vi "ControlProgram6.6_7_test_image_fixedxy.vi"() -> ()   [LabVIEW 2016]
uses:
  <vilib>/Utility/miscctls.llb/LVPoint32TypeDef.ctl
  <vilib>/Platform/TimedLoop/XDataNode/timing_clust.ctl
  <vilib>/Platform/TimedLoop/XDataNode/nitl_modes.ctl
  <vilib>/Platform/TimedLoop/XDataNode/wakeup.ctl
  <vilib>/Instr/_visa.llb/Select Event Type.ctl
  <vilib>/vision/Avi1.llb/AviRefnum.ctl
  <vilib>/Utility/error.llb/DialogType.ctl
  <vilib>/DAQmx/write.llb/DAQmx Write (Analog 1D DBL NChan 1Samp).vi
  <vilib>/DAQmx/read.llb/DAQmx Read (Analog 2D DBL NChan NSamp).vi
  <vilib>/Analysis/baseanly.llb/Mean (DBL).vi
  <vilib>/DAQmx/write.llb/DAQmx Write (Digital Bool 1Line 1Point).vi
  <vilib>/DAQmx/create/channels.llb/DAQmx Create Channel (DO-Digital Output).vi
  <vilib>/DAQmx/create/channels.llb/DAQmx Create Channel (AI-Voltage-Basic).vi
  <vilib>/DAQmx/create/channels.llb/DAQmx Create Channel (AO-Voltage-Basic).vi
  <vilib>/DAQmx/configure/timing.llb/DAQmx Timing (Sample Clock).vi
  <vilib>/DAQmx/miscellaneous.llb/DAQmx Fill In Error Info.vi
  <vilib>/Instr/_visa.llb/VISA Configure Serial Port (Instr).vi
  Arnulf--joystick/git(most_up_to_date)/Logitech-joystick/Old Trap/FAST_Global_var.vi
  <vilib>/Utility/inputDevices.llb/mouseAcquire.vi
  <vilib>/Utility/inputDevices.llb/closeMouse.vi
  <vilib>/platform/TimedLoop/XDataNode/XDataNode.xnode
  <vilib>/Platform/TimedLoop/XDataNode/XDNodeRunTimeDep.lvlib
  <resource>/objmgr/daqmx.rc
  <vilib>/Analysis/NI_AALBase.lvlib
panel:
  in  "Save file index":i32
  out "Saving Move":bool
  out "Move time":string
  out "Primary Video Display":T1(plugin-control)
  out "Flush Sample Start Time":u32=2111292881
  out "Sample flush time (s)":dbl=48.0
  in  "Inject Sample":bool
  out "Cal values":T2={"AX alpha"=612.9626061060078, "BX alpha"=549.6584469744151, "AX kappa"=0.3485731373010688, "BX kappa"=0.3853424216291352, "AX offset"=-0.03900484438240665, "BX offset"=-0.11295550662085417, "AY alpha"=582.7562541114835, "BY alpha"=571.1587543790358, "AY kappa"=0.37498408087930674, "BY kappa"=0.36252029651198364, "AY offset"=-0.21125584642206058, "BY offset"=-0.12469077200400738}
  in  "Inject Pump 1":bool
  in  "Inject Pump 2":bool
  in  "Tab Control 2":T3(tab)
  in  "Force FB script":bool
  in  "Got ADig bead":bool
  in  "Move Cap. 2 (ADig Top)":bool
  in  "Dump beads":bool
  in  "Got DNA bead":bool
  in  "Flow on\ncap 2?":bool=TRUE
  in  "Flow on\ncap 1?":bool=TRUE
  in  "Flow on\ndump?":bool=TRUE
  in  "Raster set":i32=1
  in  "Fish After TA?":bool=TRUE
  in  "Delta after tether":dbl=1700.0
  in  "TA Cancel Save?":bool=TRUE
  in  "Min fish\ndelta (nm)":dbl=1425.0 min=0.0 max=5000.0 step=50.0
  in  "Max fish\ndelta (nm)":dbl=1900.0 min=0.0 max=5000.0 step=25.0
  in  "Fish Speed (ms)":i32=5000
  in  "Wait (ms)":i32=1500
  in  "# attempts":dbl=10.0
  in  "Cutoff force (pN)":dbl=4.5
  in  "Raster after\n tether?":bool=TRUE
  out "Tether":bool
  out "Attempt #":i32
  in  "Flow on\nwhile fish?":bool=TRUE
  in  "Flow on\nafter raster?":bool=TRUE
  in  "Offset raster set":i32
  in  "Offset @ Delta (nm)":dbl=1700.0
  in  "Cal @ Delta (nm)":dbl=2500.0
  in  "Cal stage position":i32=3
  out "Cal Final Sampling Rate":dbl=125000.0
  in  "Cal Averaging":i32=1
  in  "Wait before dip (s)":dbl=3.0
  in  "Start dipping after?":bool
  in  "Start trap delta (nm)":dbl=1700.0
  in  "Repeat Dip":bool
  out "Dip #":i32
  in  "Dip attempts":dbl=3.0
  in  "Cancel Rep\n Dip":bool
  out "Return elasped time":i32
  in  "Return duration":dbl=15.0
  in  "Cancel dwell":bool=TRUE
  in  "Pause dwell":bool
  in  "Start/Return position":dbl=3.0
  in  "Dip duration":dbl=15.0
  in  "Dip position":dbl=4.0
  in  "Dip":bool
  out "Dip elasped time":i32
  in  "Stop":bool=TRUE
  in  "?":T4(tab)
  out "FAST X-Y":bool
  out "FAST Z":bool
  in  "Cal time (s)":dbl=5.0
  in  "Save N sets":bool
  in  "N sets":i32=200
  out "Cal sets to save":i32=500
  in  "Reset data stream":bool
  out "Buffer Overflow":bool
  out "Stage moving":bool
  in  "Comment":string
  in  "Raster scan":bool
  out "Saving":bool
  in  "Save cal":bool
  in  "Save Data":bool
  in  "Stop saving":bool
  out "Calibrating":bool
  out "Progress":dbl(slide) scale=0.0..100.0
  in  "Read Cal":bool
  in  "Fish":bool
  in  "Averaging Number":i32=1250
  out "Final Sampling Rate":dbl=100.0
  in  "Trap position (V)":cluster{"X":dbl, "Y":dbl}={"X"=3.9042624789680316, "Y"=0.2}
  in  "Trap delta (nm)":dbl=2500.0 min=0.0 max=5000.0 step=50.0
  in  "Fixed X":dbl=1.1
  in  "Fixed Y":dbl=0.15
  in  "Shutter 1 (B)":bool
  in  "Shutter 2 (A)":bool
  in  "Pulling direction":bool
  out "Raster scanning...":bool
  out "Current file name":path=path "D:/data/160111/160111_006.dat"
  in  "AX alpha":dbl=612.9626061060078 format="%#_3p"
  in  "BX alpha":dbl=549.6584469744151 format="%#_3g"
  in  "AX kappa":dbl=0.3485731373010688 format="%#_3g"
  in  "BX kappa":dbl=0.3853424216291352 format="%#_3g"
  in  "AX offset":dbl=-0.03900484438240665 format="%#_3g"
  in  "BX offset":dbl=-0.11295550662085417 format="%#_3g"
  in  "AY alpha":dbl=582.7562541114835 format="%#_3g"
  in  "BY alpha":dbl=571.1587543790358 format="%#_3g"
  in  "AY kappa":dbl=0.37498408087930674 format="%#_3g"
  in  "BY kappa":dbl=0.36252029651198364 format="%#_3g"
  in  "AY offset":dbl=-0.21125584642206058 format="%#_3g"
  in  "BY offset":dbl=-0.12469077200400738 format="%#_3g"
  out "Buffer status":u8(slide) scale=0.0..100.0
  in  "Target":bool
  in  "Set Current\nPos to (0,0,0)":bool
  in  "dump spot":string="Dump beads spot"
  in  "up flow spot":string="Upper flow spot"
  in  "low flow spot":string="Lower flow spot"
  in  "up cap":string="Upper capillary (ADig beads)"
  in  "bottom cap":string="Lower capillary (DNA beads)"
  in  "Move to Position 5":bool
  in  "Set Position 5":bool
  in  "Saved stage positions":dbl[][](array[numeric])=[[1.0, 0.0, 0.0, 0.0], [2.0, -0.13716, -3.21132, 0.01436], [3.0, 0.45, -0.73974, 0.005], [4.0, 0.45, -2.1978, 0.005], [5.0, 0.45, -2.63158, -0.02256]]
  in  "Set Position 2":bool
  in  "Move to Position 2":bool
  in  "Set Position 1":bool
  in  "Move to Position 1":bool
  in  "Set Position 4":bool
  in  "Move to Position 4":bool
  in  "Set Position 3":bool
  in  "Move to Position 3":bool
  out "Stage error":errorcluster
  in  "Clear Volume":bool
  out "Sample Flush Meter":u8(slide) scale=0.0..100.0
  out "Flushing Sample":bool
  in  "Flush Sample":bool
  in  "Normal \nRate (ul/hr)  3":dbl=100.0
  in  "Normal \nVolume (ul) 3":dbl=250.0
  in  "Normal \nVolume (ul) 2":dbl
  in  "Normal \nRate (ul/hr)":dbl
  in  "Normal \nVolume (ul)":dbl
  in  "Flush\nRate (ul/min)":dbl
  in  "Flush\nVolume (ul)":dbl
  in  "Flush \nRate (ul/min)  2":dbl
  in  "Flush Pump 2":bool
  in  "Flush\nVolume (ul)  2":dbl
  in  "Flush Pump 1":bool
  in  "Normal \nRate (ul/hr)  2":dbl
  in  "Write Wait":i32=1000
  in  "Flush \nRate (ul/min)  3":dbl=100.0
  in  "Flush\nVolume (ul)  3":dbl=80.0
  out "error out":errorcluster
  in  "Use Mouse to Move Trap?":bool
  in  "Pause Mouse/Mirror Connection":bool
  out "Reference Voltage":cluster{dbl, dbl}={0.0, -0.0}
  out "Saved voltage":cluster{dbl, dbl}={5.766666666666665, 1.45}
  out "Real Coordinates":cluster{"Horizontal":i32, "Vertical":i32}={"Horizontal"=897, "Vertical"=-1271}
  out "CoordinatesMousePressed":T5
  in  "Force Feedback 2":bool
  in  "Offset 2":cluster{"Off Y":dbl, "Off X":dbl}={"Off Y"=1.5, "Off X"=0.17}
  in  "Setpoint voltage 2":cluster{"SP Y":dbl, "SP X":dbl}={"SP Y"=0.6, "SP X"=0.0}
  out "Sum error":dbl(knob) scale=-0.2..0.2
  out "Trap sep":waveform(dbl)[](graph)=[{"t0"=timestamp(4.489999999999949 s since 1904-01-01), "dt"=0.002, "Y"=[-1157.7639781743756, -1157.678951177374, -1157.7582331070425, -1157.7490409992681, -1157.8995617642552], "attributes"=variant("NI_ChannelName"=variant(string "T2 X"))}, {"t0"=timestamp(4.489999999999949 s since 1904-01-01), "dt"=0.002, "Y"=[-909.0775466981794, -909.1316439023619, -909.1322956759037, -909.1570630705896, -909.1264297140281], "attributes"=variant("NI_ChannelName"=variant(string "T2 Y"))}]
  in  "Set reading to\nsetpoint 1":bool
  in  "Offset Y (nm)":dbl format="%0.2f"
  in  "Offset X (nm)":dbl format="%0.2f"
  in  "Remove offsets":bool
  in  "Force Feedback 1":bool
  out "Feedback Output \nVoltage 2":cluster{dbl, dbl} {"?" format="%#_4g"; "?" format="%#_4g"}
  in  "Offset 1":cluster{"Off Y":dbl, "Off X":dbl}={"Off Y"=1.5, "Off X"=0.17}
  in  "Setpoint voltage 1":cluster{"SP Y":dbl, "SP X":dbl}={"SP Y"=0.6, "SP X"=0.0}
  in  "Feedback const":T6={"Ki_B_Y"=0.5, "Ki_B_X"=0.0, "Kp Y"=1.0, "Kp X"=0.0}
  out "Mean Trap Pos X 2 (nm)":dbl=-1157.769953044463 format="%0.2f"
  out "Mean Trp Pos Y 2 (nm)":dbl=-909.1249958122125 format="%0.2f"
  out "T2 X RMS (A)":dbl=0.7168002469275427 format="%0.2f"
  out "T2 Y RMS (A)":dbl=0.25997187037503383 format="%0.2f"
  in  "Set reading to\nsetpoint 2":bool
  in  "Scan range (nm)":dbl=425.0
  in  "Scan speed (nm/s)":dbl=100.0 min=0.0 max=100.0
  in  "Step size (nm)":dbl=1.0
  in  "Save scans":bool=TRUE
  in  "# scans":i32=1
  in  "Load param":bool
  in  "Scan Parameters":T7(array[cluster])
  in  "Trap delta\nafter (nm)":dbl=1550.0
  in  "Stop raster":bool
  out "Scan range (V)":dbl=0.47672462142456534
  out "Scan steps (mirror)":u64=425
  out "Scan increment (V)":dbl=0.0011217049915872126
  out "Time per step (ms)":dbl=10.0
  out "Total raster time (s)":dbl=8.5
  out "N sets to be saved":dbl=850.0
  out "moveX":string
  out "moveY":string
  in  "Grid Movable Trap":bool
  in  "take fixed bead\n Images":bool
  in  "Zoom Factor":sgl=7.0
  in  "Center Point":cluster{"X":i32, "Y":i32}={"X"=335, "Y"=271}
  in  "Intensity Upper":dbl=88.0
  in  "Intensity Lower":dbl=66.0
  out "Window Size":cluster{"Height":i32, "Width":i32}
  in  "Image Index":dbl=1.0 min=1.0
  in  "Save Image":bool
  in  "Averaging":bool
  in  "Reset Averaging":bool
  in  "Save Video":bool
  in  "New Video File":bool
  in  "Video Index":dbl=1.0 min=1.0 step=1.0
  in  "Video Capture Rate (Hz)":dbl=30.0
  in  "Initial Window Size":cluster{"Width":i32, "Height":i32}={"Width"=884, "Height"=619}
  in  "Initial Window Position":cluster{"X Position":i32, "Y Position":i32}={"X Position"=796, "Y Position"=4}
  out "Window Position":cluster{"X Position":i32, "Y Position":i32}={"X Position"=40, "Y Position"=40}
  out "Path Out":path
  in  "Target coordinates":cluster{"X1":dbl, "Y1":dbl, "X2":dbl, "Y2":dbl}={"X1"=328.0, "Y1"=274.0, "X2"=368.0, "Y2"=314.0}
  out "image8bitArray":u8[][](array[numeric])
  out "GreyscaleArray":u32[](array[numeric])
  in  "take background images":bool
  in  "# Samples/channel (in)":i32=40000 format="%.2f"
  out "Buffer size\n(Samples/channel)":u32=511
  out "DAQ rate\n(Samples/s)":dbl=125000.0 format="%#_6p"
  out "# Samples/channel":i32=1250
  out "# Samples/channel/s":dbl=100.0
  out "AvailSampPerChan":u32=9
  out "Data update period (s/set)":dbl=0.01 format="%#_6p"
  out "AvailSampPerChan 2":u32=110
  in  "PC samp per channel":i32=1000
  in  "Sampling Rate":dbl=125000.0 format="%0.0p"
  in  "DAQ Rate2":dbl=1000000.0 format="%#_6p"
  out "Data period (s)":dbl=8e-06 format="%#_6p"
  in  "Save user params":bool
  in  "User":string(combo)
  in  "Load user params":bool
  in  "Tether break\nforce (pN)":dbl=1.0
  in  "Path":path=path "E:/Data"
  out "Mirror task":refnum<k21>
  in  "Conv X (nm/V)":dbl=891.5
  in  "Conv Y (nm/V)":dbl=505.7
  in  "Min value Y":dbl format="%.1g"
  in  "Max value Y":dbl=10.0 format="%.1f"
  in  "Min value X":dbl format="%0.1f"
  in  "Max value X":dbl=10.0 format="%.1f"
  in  "HWP1":string="Half waveplate 1: differential trap power"
  in  "HWP0":string="Half waveplate 0: total trap power"
  in  "Move 1":bool
  in  "\"Degrees\" 1":dbl
  in  "Move 0":bool
  in  "\"Degrees\" 0":dbl
  in  "Y command":enum16{"Fish", "Dump", "Got ADig", "Got DNA"}(ring)
  in  "B command":enum16{"Got DNA", "Got ADig", "Dump", "Fish"}(ring)
  in  "A command":enum16{"Got ADig", "Dump", "Fish", "Got DNA"}(ring)
  in  "X command":enum16{"Dump", "Fish", "Got ADig", "Got DNA"}(ring)
  out "Logitech":bool
  out "START":bool
  out "BACK":bool
  out "Right stick button":bool
  out "Left Y":i8(slide) scale=-128.0..127.0
  out "Left X":i8(slide) scale=-128.0..127.0
  out "Right Y":i8(slide) scale=-128.0..127.0
  out "Right X":i8(slide) scale=-128.0..127.0
  out "X":bool
  out "Y":bool
  out "A":bool
  out "B":bool
  out "RB":bool
  out "LB":bool
  out "R":bool
  out "L":bool
  out "D":bool
  out "U":bool
  out "Left stick button":bool
  out "FAST Z":bool
  out "FAST X-Y":bool
  in  "XY Speed Definitions":T8={"Slow X velocity input"="0.05", "Slow Y velocity input"="0.05", "Fast1 X velocity input"="0.1", "Fast1 Y velocity input"="0.1", "Fast2 X velocity input"="0.2", "Fast2 Y velocity input"="0.2"}
  in  "Z Speed Definitions":cluster{"Slow Z":string, "Fast Z":string}={"Slow Z"="0.025", "Fast Z"="0.05"}
  in  "Z Wait time":string="120"
  in  "X-Y Wait time":string="125"
  in  "USB port":refnum<visa-resource-name>="USB0::0x046D::0xC21D::CC66247B::RAW"
  out "Deflection":T5
  in  "Sampling Rate":dbl=125000.0 format="%0.2f"
  in  "Averaging Number":i32=12500
  in  "DAQ Rate":dbl=1000000.0
  out "Final Sampling Rate":dbl
  in  "Tab Control":T9(tab)
  in  "Downsamp\nfact":dbl=250.0
  out "Bead sep":waveform(dbl)[](graph)=[{"t0"=timestamp(4.489999999999949 s since 1904-01-01), "dt"=0.002, "Y"=[8093.963535945606, 8103.1617772716045, 8385.72390184118, 8245.733099167523, 8154.925676756515], "attributes"=variant("NI_ChannelName"=variant(string "T2"))}, {"t0"=timestamp(4.489999999999949 s since 1904-01-01), "dt"=0.002, "Y"=[1717.924930434114, 1628.723007842151, 1787.6888378897193, 1598.475730715916, 1776.2517588078954], "attributes"=variant("NI_ChannelName"=variant(string "T1"))}]
  out "Force (pN)":waveform(dbl)[](graph)=[{"t0"=timestamp(4.489999999999949 s since 1904-01-01), "dt"=0.002, "Y"=[2821.5994183803123, 2824.8226375853515, 2923.3663028678166, 2874.5254578927593, 2842.869034836209], "attributes"=variant("NI_ChannelName"=variant(string "T2"))}, {"t0"=timestamp(4.489999999999949 s since 1904-01-01), "dt"=0.002, "Y"=[623.5850847499229, 591.0680427774053, 648.761979867749, 579.944408346982, 644.7436619059413], "attributes"=variant("NI_ChannelName"=variant(string "T1"))}]
  out "Mean force (pN)":dbl=1737.5286029210451 format="%0.2f"
  out "Force noise (pN)":dbl=26.83032703631318 format="%0.2f"
  out "Mean Bead Sep\n(nm)":dbl=4949.257225667222 format="%0.2f"
  out "Bead Sep Noise\n(A)":dbl=757.8078481959694 format="%0.2f"
  out "PSD 2":cluster{dbl[], dbl[]}(graph)
  out "PSD 1":cluster{dbl[], dbl[]}(graph)
  out "PSD 1 Sum":dbl(slide) scale=0.0..10.0
  out "PSD 2 Sum":dbl(slide) scale=0.0..10.0
  in  "Start":bool
  out "All signals 2":waveform(dbl)[](graph)=[{"t0"=timestamp(4.489999999999949 s since 1904-01-01), "dt"=0.002, "Y"=[0.0010396217068286443, 0.0010666908927528754, 0.001103298744846499, 0.0010651440823993424, 0.0010656596859401936], "attributes"=variant("NI_ChannelName"=variant(string "A y"))}, {"t0"=timestamp(4.489999999999949 s since 1904-01-01), "dt"=0.002, "Y"=[0.02000680227246931, 0.020097032918054827, 0.02003412926844257, 0.020136734401221615, 0.020087494249822452], "attributes"=variant("NI_ChannelName"=variant(string "A x"))}, {"t0"=timestamp(4.489999999999949 s since 1904-01-01), "dt"=0.002, "Y"=[-0.0014958587831537804, -0.0015046240440107857, -0.0014930229638311983, -0.001533240041751485, -0.0015262793936602433], "attributes"=variant("NI_ChannelName"=variant(string "B y"))}, {"t0"=timestamp(4.489999999999949 s since 1904-01-01), "dt"=0.002, "Y"=[0.0002901198559372817, 0.0002731049385577592, 0.00026511308349727467, 0.0002517073909711183, 0.0002916666665966012], "attributes"=variant("NI_ChannelName"=variant(string "B x"))}, {"t0"=timestamp(4.489999999999949 s since 1904-01-01), "dt"=0.002, "Y"=[-0.001511556786147372, -0.0015167122027053212, -0.0014612914746018214, -0.0014935128282145193, -0.0015064013696263116], "attributes"=variant("NI_ChannelName"=variant(string "A sum"))}, {"t0"=timestamp(4.489999999999949 s since 1904-01-01), "dt"=0.002, "Y"=[-0.0005242945138364382, -0.0005565158674093218, -0.000501095139248956, -0.0005771375336978897, -0.0005165613890095197], "attributes"=variant("NI_ChannelName"=variant(string "B sum"))}, {"t0"=timestamp(4.489999999999949 s since 1904-01-01), "dt"=0.002, "Y"=[0.0013303666019343777, 0.0014257418088905328, 0.0013368108726387405, 0.0013471217058124534, 0.0011782818123890176], "attributes"=variant("NI_ChannelName"=variant(string "Trap x"))}, {"t0"=timestamp(4.489999999999949 s since 1904-01-01), "dt"=0.002, "Y"=[0.0023382505474007294, 0.002231275652833831, 0.002229986798687363, 0.0021810103409340116, 0.002241586486003531], "attributes"=variant("NI_ChannelName"=variant(string "Trap y"))}]
  out "All signals":waveform(dbl)[](graph)=[{"t0"=timestamp(4.489999999999949 s since 1904-01-01), "dt"=0.002, "Y"=[0.0010396217068286443, 0.0010666908927528754, 0.001103298744846499, 0.0010651440823993424, 0.0010656596859401936], "attributes"=variant("NI_ChannelName"=variant(string "A y"))}, {"t0"=timestamp(4.489999999999949 s since 1904-01-01), "dt"=0.002, "Y"=[0.02000680227246931, 0.020097032918054827, 0.02003412926844257, 0.020136734401221615, 0.020087494249822452], "attributes"=variant("NI_ChannelName"=variant(string "A x"))}, {"t0"=timestamp(4.489999999999949 s since 1904-01-01), "dt"=0.002, "Y"=[-0.0014958587831537804, -0.0015046240440107857, -0.0014930229638311983, -0.001533240041751485, -0.0015262793936602433], "attributes"=variant("NI_ChannelName"=variant(string "B y"))}, {"t0"=timestamp(4.489999999999949 s since 1904-01-01), "dt"=0.002, "Y"=[0.0002901198559372817, 0.0002731049385577592, 0.00026511308349727467, 0.0002517073909711183, 0.0002916666665966012], "attributes"=variant("NI_ChannelName"=variant(string "B x"))}, {"t0"=timestamp(4.489999999999949 s since 1904-01-01), "dt"=0.002, "Y"=[-0.001511556786147372, -0.0015167122027053212, -0.0014612914746018214, -0.0014935128282145193, -0.0015064013696263116], "attributes"=variant("NI_ChannelName"=variant(string "A sum"))}, {"t0"=timestamp(4.489999999999949 s since 1904-01-01), "dt"=0.002, "Y"=[-0.0005242945138364382, -0.0005565158674093218, -0.000501095139248956, -0.0005771375336978897, -0.0005165613890095197], "attributes"=variant("NI_ChannelName"=variant(string "B sum"))}, {"t0"=timestamp(4.489999999999949 s since 1904-01-01), "dt"=0.002, "Y"=[0.0013303666019343777, 0.0014257418088905328, 0.0013368108726387405, 0.0013471217058124534, 0.0011782818123890176], "attributes"=variant("NI_ChannelName"=variant(string "Trap x"))}, {"t0"=timestamp(4.489999999999949 s since 1904-01-01), "dt"=0.002, "Y"=[0.0023382505474007294, 0.002231275652833831, 0.002229986798687363, 0.0021810103409340116, 0.002241586486003531], "attributes"=variant("NI_ChannelName"=variant(string "Trap y"))}]
  out "Chart Freq (Hz)":dbl=500.0
  # "Bead Calibration"
  # "Y"
  # "X"
  # "Pump #1 Controls"
  # "Pump #2 Controls"
  # "Sample Pump Controls"
  # "Retract the pumps manually. Change it back to INFUSE when you're done. Suck it up, don't whine."
  # "Shutter 1 (B)"
  # "Move to Lower Cap"
  # "Inject Sample"
  # "Move to Upper Cap"
  # "Shutter 2 (A)"
  # "Select the Joystick input:"
  # "Overflow happens when >40 commands\nsent in 5 seconds. Then 4 consecutive beeps."
  # "Try increasing wait time to reduce 'following error threshold exceeded' occurances."
  # "Left stick controls Z axis.\nRight on stick: neg Z-dir\nUp on stick: neg Z-dir"
  # "Toggles FAST Z"
  # "Toggles FAST X-Y"
  # "The default Newport max velocity is 0.4"
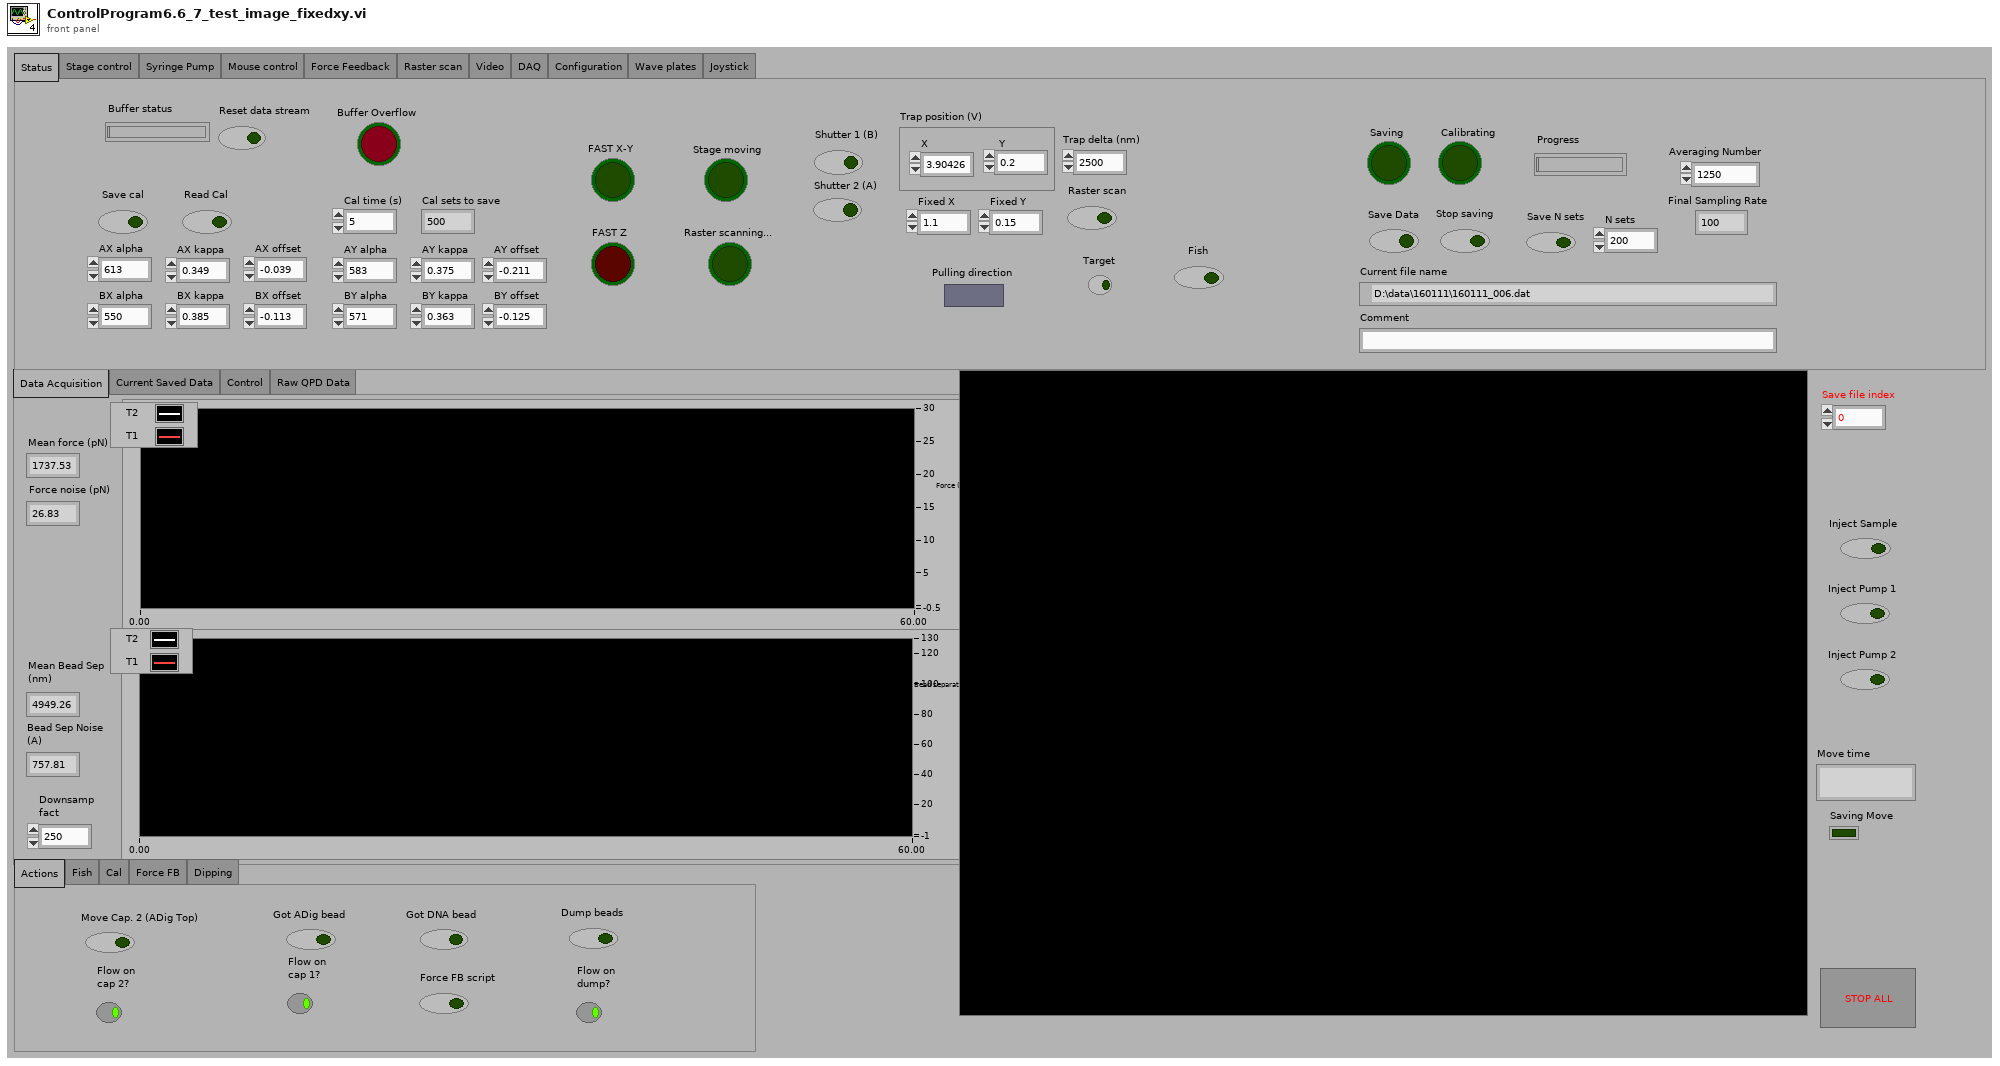
[diagram p1: front panel]
types:
  T1 = typedef "IMAQ Image.ctl" = refnum<image>
  T2 = cluster{"AX alpha":dbl, "BX alpha":dbl, "AX kappa":dbl, "BX kappa":dbl, "AX offset":dbl, "BX offset":dbl, "AY alpha":dbl, "BY alpha":dbl, "AY kappa":dbl, "BY kappa":dbl, "AY offset":dbl, "BY offset":dbl}
  T3 = enum32{"Actions", "Fish", "Cal", "Force FB", "Dipping"}
  T4 = enum32{"Status", "Stage control", "Syringe Pump", "Mouse control", "Force Feedback", "Raster scan", "Video", "DAQ", "Configuration", "Wave plates", "Joystick"}
  T5 = typedef "LVPoint32TypeDef.ctl" = cluster{"Horizontal":i32, "Vertical":i32}
  T6 = cluster{"Ki_B_Y":dbl, "Ki_B_X":dbl, "Kp Y":dbl, "Kp X":dbl}
  T7 = cluster{"Label":string, "Scan range 1":dbl, "Step size 1":dbl, "Scan speed 1":i32, "# scans 2":i32}[]
  T8 = cluster{"Slow X velocity input":string, "Slow Y velocity input":string, "Fast1 X velocity input":string, "Fast1 Y velocity input":string, "Fast2 X velocity input":string, "Fast2 Y velocity input":string}
  T9 = enum32{"Data Acquisition", "Current Saved Data", "Control", "Raw QPD Data"}
  T10 = typedef "Select Event Type.ctl" = u32
  T11 = enum32{"setting", "request", "request control", "info", "statistics", "system settings", "I/O sub system", "HRT control", "camera descriptions", "device specific data", "event sub system settings", "event sub system results", "image memory manager"}
  T12 = typedef "AviRefnum.ctl" = refnum<k1>
  T13 = typedef "XDNodeRunTimeDep.lvlib/timing_clust.ctl" = cluster{"Expected End [f-1]":u64, "Actual End [f-1]":u64, "Finished Late? [f-1]":bool, "Expected End [i-1]":u64, "Actual End [i-1]":u64, "Finished Late? [i-1]":bool, "Expected Start [i]":u64, "Actual Start [i]":u64, "Expected Start [f]":u64, "Actual Start [f]":u64, "Source Name":string, "Structure Name":string, "Period":i64, "Deadline":i64, "Offset":i64, "Start":i64, "Priority":i32, "Timeout":i32, "Mode":T14, "Wakeup Reason":T15, "Error":errorcluster, "Source Type":string, "Secondary Source Type":string, "Global End Time":u64, "Global Start Time":u64, "Frame Duration":u64, "Iteration Duration":u64, "Assigned CPU":i32, "I/O Scan Engine Mode":u32}
  T14 = typedef "XDNodeRunTimeDep.lvlib/nitl_modes.ctl" = enum32{"No Change", "Process missed periods, maintain original phase", "Discard missed periods, maintain original phase", "Process missed periods, ignore original phase", "Discard missed periods, ignore original phase"}
  T15 = typedef "XDNodeRunTimeDep.lvlib/wakeup.ctl" = enum32{"Normal", "Aborted", "Asynchronous wakeup", "Timing source error", "Timed loop error", "Timeout"}
  T16 = typedef "Image Type" = u32
  T17 = typedef "imagedata.ctl" = cluster{"image type":i32, "image depth":i32, "image":u8[], "mask":u8[], "colors":u32[], "Rectangle":cluster{"left":i16, "top":i16, "right":i16, "bottom":i16}}
  T18 = enum16{"open", "replace", "create", "open or create", "replace or create", "replace or create with confirmation"}
  T19 = enum16{"big-endian, network order", "native, host order", "little-endian"}
  T20 = cluster{string, string, string, string, string, string, string, string}
  T21 = cluster{"LB":bool, "RB":bool, "BACK":bool, "Logitech":bool, "START":bool}
  T22 = cluster{"Right X":i8, "Right Y":i8, "Left X":i8, "Left Y":i8}
  T23 = enum32{"Status", "Stage control", "Syringe Pump", "Mouse control", "Force Feedback", "Raster scan", "Video", "DAQ", "Configuration", "Wave plates"}
  T24 = typedef "DialogType.ctl" = u16
  T25 = cluster{"button 1":bool, "button 2":bool, "button 3":bool, "button 4":bool}
  T26 = cluster{"[0]":dbl, "[1]":dbl, "[2]":dbl, "[3]":dbl, "[4]":dbl, "[5]":dbl, "[6]":dbl, "[7]":dbl, "[8]":dbl, "[9]":dbl, "[10]":dbl, "[11]":dbl}
  T27 = cluster{"Label":string, "Scan range 1":dbl, "Step size 1":dbl, "Scan speed 1":i32, "# scans 2":i32}
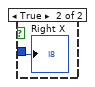
[diagram p5: hidden frame]
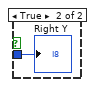
[diagram p6: hidden frame]
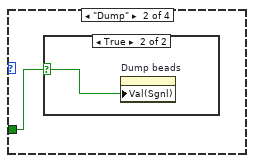
[diagram p10: hidden frame]
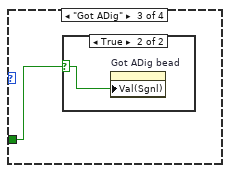
[diagram p12: hidden frame]
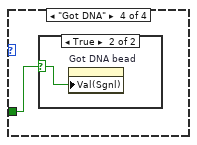
[diagram p14: hidden frame]
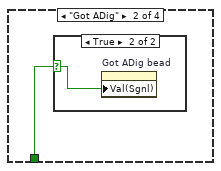
[diagram p17: hidden frame]
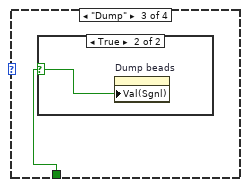
[diagram p19: hidden frame]
diagram:
  w10 = T10 1073684535 items=["Service Request"=1073684491, "Trigger"=3221168138, "Clear"=1073684493, "VXI Signal"=1073684512, "VXI/VME Interrupt"=3221168161, "VXI/VME Sysfail"=1073684509, "VXI/VME Sysreset"=1073684510, "GPIB CIC"=1073684498, "GPIB Talk"=1073684499, "GPIB Listen"=1073684500, "PXI Interrupt"=1073684514, "Serial Break"=1073684515, "Serial TermChar"=1073684516, "Serial CTS"=1073684521, "Serial DSR"=1073684522, "Serial DCD"=1073684524, "Serial RI"=1073684526, "Serial Character"=1073684533, "USB Interrupt"=1073684535, "All Enabled"=1073709055] ("Event Type")
  w49 = 10.0 ("Minimum Value")
  w50 = -10.0 ("Minimum Value")
  w52 = -2.0 ("Minimum Value")
  w53 = 2.0 ("Maximum Value")
  w78 = 10123 items=["Finite Samples"=10178, "Continuous Samples"=10123] ("sample mode")
  w98 = tag "Dev1/port2/line1"  # Shutter 2
  w101 = tag "Dev1/port1/line4"  # Shutter 1
  # "Open the RAW resource"
  # "Enable USB Interrupt Event"
  # "Create channels for movable mirror"
  # "Create channels for detectors"
  n1 = call-poly <vilib>:"DAQmx Create Virtual Channel.vi"("maximum value"=w53, "minimum value"=w52, "physical channels"=tag "Dev1/ai0" ("Physical Channel")) -> ("task out"=w54:refnum<k21>, "error out"=w77:errorcluster)  [unwired: 11 in]
  n2 = call-poly <vilib>:"DAQmx Create Virtual Channel.vi"("task in"=w54, "maximum value"=w53, "minimum value"=w52, "physical channels"=tag "Dev1/ai1", "error in"=w77) -> ("task out"=w75:refnum<k21>, "error out"=w74:errorcluster)  [unwired: 9 in]
  n3 = call-poly <vilib>:"DAQmx Create Virtual Channel.vi"("task in"=w75, "maximum value"=w53, "minimum value"=w52, "physical channels"=tag "Dev1/ai2", "error in"=w74) -> ("task out"=w66:refnum<k21>, "error out"=w65:errorcluster)  [unwired: 9 in]
  n4 = call-poly <vilib>:"DAQmx Create Virtual Channel.vi"("task in"=w66, "maximum value"=w53, "minimum value"=w52, "physical channels"=tag "Dev1/ai3" ("Physical Channel"), "error in"=w65) -> ("task out"=w51:refnum<k21>, "error out"=w71:errorcluster)  [unwired: 9 in]
  n5 = call-poly <vilib>:"DAQmx Create Virtual Channel.vi"("task in"=w51, "maximum value"=w49, "minimum value"=w50, "physical channels"=tag "Dev1/ai4", "error in"=w71) -> ("task out"=w69:refnum<k21>, "error out"=w68:errorcluster)  [unwired: 9 in]
  n6 = call-poly <vilib>:"DAQmx Create Virtual Channel.vi"("task in"=w69, "maximum value"=w49, "minimum value"=w50, "physical channels"=tag "Dev1/ai5", "error in"=w68) -> ("task out"=w64:refnum<k21>, "error out"=w63:errorcluster)  [unwired: 9 in]
  n7 = call-poly <vilib>:"DAQmx Create Virtual Channel.vi"("task in"=w64, "maximum value"=w49, "minimum value"=w50, "physical channels"=tag "Dev1/ai6", "error in"=w63) -> ("task out"=w58:refnum<k21>, "error out"=w56:errorcluster)  [unwired: 9 in]
  n8 = call-poly <vilib>:"DAQmx Create Virtual Channel.vi"("task in"=w58, "maximum value"=w49, "minimum value"=w50, "physical channels"=tag "Dev1/ai7", "error in"=w56) -> ("task out"=w57:refnum<k21>, "error out"=w55:errorcluster)  [unwired: 9 in]
  n9 = call-poly <vilib>:"DAQmx Timing.vi"("task/channels in"=w57, "sample mode"=w78, "samples per channel"="PC samp per channel", "rate"="Sampling Rate", "error in"=w55) -> ("task out"=w61:refnum<k21>, "error out"=w60:errorcluster)  [unwired: 9 in]
  n10 = call-poly <vilib>:"DAQmx Create Virtual Channel.vi"("maximum value"="Max value Y", "minimum value"="Min value Y", "physical channels"=tag "Dev1/ao1" ("Trap X Axis")) -> ("task out"=w46:refnum<k21>, "error out"=w48:errorcluster)  [unwired: 11 in]
  n11 = property class="DAQmx Timing"(reference=w61, error in=w60, "More:AI Convert:Rate"="DAQ Rate2") -> (reference out=w19:refnum<k21>, error out=w18:errorcluster, "SampClk.Rate"=→"DAQ rate\n(Samples/s)":dbl)
  n12 = call-poly <vilib>:"DAQmx Create Virtual Channel.vi"("task in"=w46, "maximum value"="Max value X", "minimum value"="Min value X", "physical channels"=tag "Dev1/ao0" ("Trap Y Axis"), "error in"=w48) -> ("task out"=w37:refnum<k21>, "error out"=w36:errorcluster)  [unwired: 9 in]
  "Mirror task" <- w37
  n13 = property class="DAQmx Buffer"(reference=w19, error in=w18) -> (reference out=w16:refnum<k21>, error out=w15:errorcluster, "Input.OnbrdBufSize"=→"Buffer size\n(Samples/channel)":u32)
  n14 = call <vilib>:"DAQmx Start Task.vi"("task/channels in"=w16, "error in"=w15) -> ("task out"=w38:refnum<k21>)  [unwired: 12 in, 1 out]
  n15 = flat-sequence "Video" {
    tunnel: [w114] -> w13
    tunnel: w13 -> [w155]
    frame #0 {
      n16 = while {
        stop <- w107 continue-if-true
        n17 = call "Close Video Capture.vi"() -> ("error code OUT"=w109:i32)
        n18 = Equal?(x=w109, y=0) -> (x = y?=w107:bool)
      }
      n19 = local write "Stop"(FALSE ("Stop All")) -> ()
    }
    frame #1 {
      n20 = call "DMR_Init.vi"() -> ()  [unwired: 3 out]
    }
    frame #2 {
      # "Setting the destination format to Mono8 makes sure that the image can be displayed in the intensity plot."
      n21 = call "DMR_GetDevice.vi"("search string IN"="DE514724602") -> ("device handle OUT"=w132:i32)  [unwired: 4 in, 2 out]
      n22 = call "DMR_OpenDevice.vi"("device handle IN"=w132) -> ("driver handle OUT"=w115:i32)  [unwired: 4 out]
      n23 = call "DMR_FindList.vi"("flags IN"=u32 0 ("flags"), "list name IN"="" ("String"), "list type IN"=T11."camera descriptions", "driver handle IN"=w115) -> ("list handle OUT"=w118:i32)  [unwired: 2 out]
      n24 = call "DMR_FindList.vi"("flags IN"=u32 0 ("flags"), "list name IN"="Base", "list type IN"=T11."setting", "driver handle IN"=w115) -> ("list handle OUT"=w116:i32)  [unwired: 2 out]
      n25 = call "OBJ_GetHandle.vi"("object name IN"="VideoStandard", "list handle IN"=w118) -> ("object handle OUT"=w112:i32)  [unwired: 3 out]
      n26 = call "OBJ_GetHandle.vi"("object name IN"="PixelFormat", "list handle IN"=w116) -> ("object handle OUT"=w126:i32)  [unwired: 3 out]
      n27 = call "OBJ_SetS.vi"("value index IN"=0, "value IN"="NTSC M", "object handle IN"=w112) -> ()  [unwired: 2 out]
      n28 = call "OBJ_SetS.vi"("value index IN"=0, "value IN"="Mono8" ("value"), "object handle IN"=w126) -> ()  [unwired: 2 out]
      n29 = call "OBJ_GetHandle.vi"("object name IN"="VideoChannel", "list handle IN"=w116) -> ("object handle OUT"=w122:i32)  [unwired: 3 out]
      n30 = while {
        tunnel: [w137] -> w114
        tunnel: w115 -> [w134]
        stop <- w135 continue-if-true
        n31 = call "DMR_ImageRequestSingle.vi"("request control IN"=0, "driver handle IN"=w134) -> ("error code OUT"=w136:i32, "driver handle OUT"=w137:i32)  [unwired: 2 out]
        n32 = Equal To 0?(x=w136) -> (x = 0?=w135:bool)
      }
      n33 = call "OBJ_SetI.vi"("value index IN"=0, "value IN"=0 ("Video channel"), "object handle IN"=w122) -> ()  [unwired: 2 out]
    }
    frame #3 {
      w143 = T16 0 items=["Grayscale (U8)", "Grayscale (I16)", "Grayscale (SGL)", "Complex (CSG)", "RGB (U32)", "HSL (U32)", "RGB (U64)"] ("Image Type")
      w151 = T16 0 items=["Grayscale (U8)", "Grayscale (I16)", "Grayscale (SGL)", "Complex (CSG)", "RGB (U32)", "HSL (U32)", "RGB (U64)"] ("Image Type")
      n34 = for "Create Greyscale map" {
        N: 256 -> [_]
        tunnel: [w157] -> w140 mode=indexing
        workers-P: _ -> [_]
        i -> [w160]
        n35 = To Unsigned Byte Integer(number=w160) -> (unsigned 8bit integer=w156:u8)
        n36 = Join Numbers(hi=w156, lo=w156) -> ((hi.lo)=w159:u16)
        n37 = Join Numbers(hi=w156, lo=w156) -> ((hi.lo)=w158:u16)
        n38 = Join Numbers(hi=w159, lo=w158) -> ((hi.lo)=w157:u32)
      }
      n39 = call "IMAQ Create"("Image Name"="Scaled video", "Image Type"=w143) -> ("New Image"=w142:T1)  [unwired: 2 in, 2 out]
      n40 = call "IMAQ Create"("Image Name"="Main video", "Image Type"=w151) -> ("New Image"=w152:T1)  [unwired: 2 in, 2 out]
      n41 = node-c288(0 ("Processor")) -> (w150:T13)  [unwired: 3 out]
      n42 = Initialize Array(u32 0 ("Window Number (0...15)"), 480 ("dimension size"), 640 ("dimension size")) -> (w145:u32[][])
      n43 = timed-loop {
        tunnel: w155 -> [w177]
        tunnel: [w176] -> w154
        tunnel: w152 -> [w175]
        timing: w150 -> [_]
        timing-out: [_] -> w149
        tunnel: w145 -> [w164]
        tunnel: w142 -> [w162]
        tunnel: w140 -> [w161]
        stop <- w163 stop-if-true
        # "This block performs the \nactual image capture."
        n44 = node-c288() -> ()  [unwired: 2 out]
        n45 = local read "Stop"() -> (w163:bool)
        n46 = Reciprocal(x="Video Capture Rate (Hz)") -> (1/x=w167:dbl)
        n47 = Multiply(x=w167, y=1000.0) -> (x*y=w165:dbl)
        n48 = call "DMR_ImageRequestWaitFor.vi"("queue number IN"=0, "timeout(ms) IN"=500, "driver handle IN"=w177) -> ("error code OUT"=w181:i32, "request number OUT"=w178:i32, "driver handle OUT"=w179:i32)
        n49 = feedback #1(T12 refnum ("Avi Refnum")) -> (w169:T12)
        n50 = case shown="True" "New Video File" {
          tunnel: [T12 refnum ("Avi Refnum") w198] -> w171
          tunnel: [FALSE TRUE] -> w172
          tunnel: w169 -> [_ w194]
          frame False {
          }
          frame True {
            n51 = call "Create new save file.vi"("Ext"=".avi" ("string"), "Index In"="Video Index") -> ("Path Out"=w190:path, "Index Out"=w191:dbl)  [unwired: 1 in]
            "Path Out" <- w190
            n52 = Not Equal?(x=w194, y=T12 refnum ("Avi Refnum")) -> (x != y?=w195:bool)
            n53 = Increment(x=w191) -> (x+1=w200:dbl)
            n54 = case shown="True" w195 {
              tunnel: w194 -> [_ w201]
              frame False {
              }
              frame True {
                n55 = call "IMAQ AVI Close"("Avi Refnum"=w201) -> ()  [unwired: 1 in, 10 out]
              }
            }
            n56 = local write "Video Index"(w200) -> ()
            n57 = call "IMAQ AVI Create"("Frames Per Second"=u32 30, "AVI Path"=w190) -> ("Avi Refnum"=w198:T12)  [unwired: 5 in, 4 out]
          }
        }
        n58 = Equal To 0?(x=w181) -> (x = 0?=w180:bool)
        n59 = Select(t=w171, s=w172, f=w169) -> (s? t:f=w170:T12)
        n60 = feedback-in #1(w170) -> ()
        n61 = case shown="True" w180 {
          tunnel: w179 -> [w202 w231]
          tunnel: w178 -> [_ w230]
          tunnel: [w202 w227] -> w176
          tunnel: w175 -> [_ w210]
          tunnel: w164 -> [_ w215]
          tunnel: w170 -> [_ w213]
          tunnel: w162 -> [_ w211]
          tunnel: w161 -> [_ w204]
          frame False {
          }
          frame True {
            w221 = u32 0 ("X-offset IN")
            n62 = call "DMR_GetImageRequestBufferData.vi"("driver handle IN"=w231, "request number IN"=w230) -> ("width OUT"=w220:i32, "height OUT"=w219:i32, "driver handle OUT"=w226:i32, "request number OUT"=w225:i32, "bytes per pixel OUT"=w222:i32)  [unwired: 13 out]
            n63 = call "DMR_GetImageRequestBufferImageData.vi"("driver handle IN"=w226, "request number IN"=w225, "bytes per pixel IN"=w222, "X-offset IN"=w221, "Y-offset IN"=w221, "height IN"=w219, "width IN"=w220) -> ("driver handle OUT"=w224:u32, "request number OUT"=w223:u32, "image OUT"=w216:u32[][])  [unwired: 10 out]
            n64 = call "DMR_ImageRequestUnlock.vi"("request number IN"=w223, "driver handle IN"=w224) -> ("driver handle OUT"=w229:i32)  [unwired: 1 in, 2 out]
            n65 = case shown="False" "Averaging" {
              tunnel: w216 -> [w307 w312]
              tunnel: [w307 w311] -> w212
              tunnel: w215 -> [_ w309]
              frame False {
              }
              frame True {
                (unwired) 1
                w317 = 1
                n66 = feedback #2(w309) -> (w308:u32[][])
                n67 = Add(x=w312, y=w308) -> (x+y=w313:u32[][])
                n68 = Select(t=w309, s="Reset Averaging", f=w313) -> (s? t:f=w315:u32[][])
                n69 = feedback-in #2(w315) -> ()
                n70 = feedback #3(w317) -> (w310:i32)
                n71 = Divide(x=w313, y=w310) -> (x/y=w314:dbl[][])
                n72 = Increment(x=w310) -> (x+1=w318:i32)
                n73 = To Unsigned Long Integer(number=w314) -> (unsigned 32bit integer=w311:u32[][])
                n74 = Select(t=w317, s="Reset Averaging", f=w318) -> (s? t:f=w316:i32)
                n75 = feedback-in #3(w316) -> ()
              }
            }
            n76 = call "DMR_ImageRequestSingle.vi"("request control IN"=0, "driver handle IN"=w229) -> ("driver handle OUT"=w227:i32)  [unwired: 3 out]
            n77 = disable-structure shown="Disabled" {
              disable-tunnel: w212 -> [w284 _]
              disable-tunnel: w211 -> [w283 _]
              frame Disabled {
                n78 = To Double Precision Float(number=w284) -> (double precision float=w282:dbl[][])
                n79 = In Range and Coerce(upper limit="Intensity Upper", x=w282, lower limit="Intensity Lower") -> (coerced(x)=w281:dbl[][])  [unwired: 1 out]
                n80 = Subtract(x="Intensity Upper", y="Intensity Lower") -> (x-y=w278:dbl)
                n81 = Subtract(x=w281, y="Intensity Lower") -> (x-y=w279:dbl[][])
                n82 = Divide(x=w279, y=w278) -> (x/y=w280:dbl[][])
                n83 = Multiply(x=255.0, y=w280) -> (x*y=w276:dbl[][])
                n84 = To Unsigned Byte Integer(number=w276) -> (unsigned 8bit integer=w285:u8[][])
                n85 = call "IMAQ ArrayToImage"("Image Pixels (U8)"=w285, "Image"=w283) -> ("Image Out"=w272:T1)  [unwired: 4 in, 5 out]
                n86 = First Call?() -> (First Call?: T/F=w273:bool)
                n87 = case shown="True" w273 {
                  tunnel: w272 -> [w286 w297]
                  frame False {
                    n88 = flat-sequence {
                      tunnel: w286 -> [w292]
                      frame #0 {
                        w289 = FALSE ("Get/Set Status? (Set)")
                        w288 = 0 ("Window Number (0...15)")
                        n89 = call "IMAQ WindSize"("Get/Set Status? (Set)"=w289, "Window Number"=w288) -> ("Width & Height out"=→"Window Size":cluster{"Width":i32, "Height":i32})  [unwired: 4 in, 2 out]
                        n90 = call "IMAQ WindMove"("Window Number (0...15)"=w288, "Get/Set Status? (Set)"=w289) -> ("Coordinates (screen)"=→"Window Position":cluster{"X Position":i32, "Y Position":i32})  [unwired: 3 in, 1 out]
                        n91 = call "IMAQ WindDraw"("Resize to Image Size? (Y)"=FALSE, "Window Number (0...15)"=w288, "Image"=w292) -> ()  [unwired: 7 in, 2 out]
                      }
                      frame #1 {
                        n92 = call "IMAQ WindZoom 2"("Center Point"="Center Point", "Zoom to Fit? (False)"=FALSE, "Zoom Factor"="Zoom Factor") -> ()  [unwired: 5 in, 4 out]
                      }
                    }
                  }
                  frame True {
                    n93 = flat-sequence {
                      tunnel: w297 -> [w300]
                      tunnel: [w298] -> w296
                      tunnel: w296 -> [w302]
                      frame #0 {
                        w299 = TRUE ("Resize to Image Size? (Y)")
                        w298 = 0 ("Window Number (0...15)")
                        n94 = call "IMAQ WindNonTearing"("Window Number"=w298, "NonTearing? (True)"=w299) -> ()  [unwired: 8 in, 2 out]
                        n95 = call "IMAQ WindDraw"("Resize to Image Size? (Y)"=w299, "Window Number (0...15)"=w298, "Image"=w300) -> ()  [unwired: 7 in, 2 out]
                      }
                      frame #1 {
                        n96 = call "IMAQ WindSize"("Scrollbars? (N)"=FALSE, "Width & Height"="Initial Window Size", "Window Number"=w302) -> ()  [unwired: 3 in, 3 out]
                        n97 = call "IMAQ WindMove"("Window Number (0...15)"=w302, "Coordinates (screen)"="Initial Window Position") -> ()  [unwired: 3 in, 2 out]
                      }
                    }
                  }
                }
              }
              frame Enabled {
              }
            }
            n98 = To Unsigned Byte Integer(number=w212) -> (unsigned 8bit integer=w203:u8[][])
            "image8bitArray" <- w203
            n99 = call "IMAQ ArrayToImage"("Image Pixels (U8)"=w203, "Image"=w210) -> ("Image Out"=w208:T1)  [unwired: 4 in, 5 out]
            n100 = case shown="True" "take fixed bead\n Images" {
              tunnel: w203 -> [_ w251]
              tunnel: w204 -> [_ w250]
              frame False {
              }
              frame True {
                n101 = local write "take fixed bead\n Images"(FALSE ("Save 10 Images")) -> ()
                n102 = while {
                  tunnel: w251 -> [w253]
                  tunnel: w250 -> [w252]
                  i -> [w255]
                  stop <- w254 stop-if-true
                  n103 = flat-sequence {
                    tunnel: w253 -> [w265]
                    tunnel: w252 -> [w264]
                    frame #0 {
                      n104 = local read "Image Index"() -> (w261:dbl)
                      n105 = call "Create new save file.vi"("Insert"="fixed_" ("string"), "Ext"=".bmp" ("string"), "Index In"=w261) -> ("Path Out"=w262:path, "Index Out"=w258:dbl)
                      n106 = call <vilib>:"Flatten Pixmap.vi"("colors"=w264, "8-bit pixmap"=w265) -> ("image data"=w263:T17)  [unwired: 4 in, 5 out]
                      n107 = Increment(x=w258) -> (x+1=w257:dbl)
                      n108 = call <vilib>:"Write BMP File.vi"("image data"=w263, "path to BMP file"=w262) -> ()  [unwired: 1 in, 9 out]
                      n109 = local write "Image Index"(w257) -> ()
                    }
                    frame #1 {
                      n110 = Wait (ms)(milliseconds to wait=u32 50) -> ()  [unwired: 1 out]
                    }
                  }
                  n111 = Equal?(x=w255, y=9) -> (x = y?=w254:bool)
                }
              }
            }
            n112 = case shown="True" "Save Video" {
              tunnel: w213 -> [_ w306]
              tunnel: w208 -> [_ w305]
              frame False {
              }
              frame True {
                n113 = call "IMAQ AVI Write Frame"("Image"=w305, "Avi Refnum"=w306) -> ()  [unwired: 2 in, 8 out]
              }
            }
            n114 = case shown="True" "take background images" {
              tunnel: w204 -> [_ w233]
              tunnel: w203 -> [_ w232]
              frame False {
              }
              frame True {
                n115 = while {
                  tunnel: w233 -> [w235]
                  tunnel: w232 -> [w234]
                  i -> [w238]
                  stop <- w236 stop-if-true
                  n116 = flat-sequence {
                    tunnel: w235 -> [w240]
                    tunnel: w234 -> [w239]
                    frame #0 {
                      n117 = local read "Image Index"() -> (w246:dbl)
                      n118 = call "Create new save file.vi"("Insert"="background_" ("string"), "Ext"=".bmp" ("string"), "Index In"=w246) -> ("Path Out"=w242:path, "Index Out"=w243:dbl)
                      n119 = call <vilib>:"Flatten Pixmap.vi"("colors"=w240, "8-bit pixmap"=w239) -> ("image data"=w241:T17)  [unwired: 4 in, 5 out]
                      n120 = Increment(x=w243) -> (x+1=w247:dbl)
                      n121 = local write "Image Index"(w247) -> ()
                      n122 = call <vilib>:"Write BMP File.vi"("image data"=w241, "path to BMP file"=w242) -> ()  [unwired: 1 in, 9 out]
                    }
                    frame #1 {
                      n123 = Wait (ms)(milliseconds to wait=u32 50) -> ()  [unwired: 1 out]
                    }
                  }
                  n124 = Equal?(x=w238, y=9) -> (x = y?=w236:bool)
                }
              }
            }
            n125 = case shown="False" "Target" {
              tunnel: w208 -> [w267 w271]
              tunnel: [w267 w269] -> w207
              frame False {
              }
              frame True {
                n126 = local read "Target coordinates"() -> (w268:cluster{"X1":dbl, "Y1":dbl, "X2":dbl, "Y2":dbl})
                n127 = call "IMAQ Overlay Oval"("Color"=u32 16711680, "Bounding Rectangle"=w268, "Image"=w271) -> ("Image Out"=w269:T1)  [unwired: 7 in, 1 out]
              }
            }
            "Primary Video Display" <- w207
            n128 = case shown="True" "Save Image" {
              tunnel: w203 -> [_ w321]
              tunnel: w204 -> [_ w320]
              frame False {
              }
              frame True {
                n129 = call <vilib>:"Flatten Pixmap.vi"("colors"=w320, "8-bit pixmap"=w321) -> ("image data"=w327:T17)  [unwired: 4 in, 5 out]
                n130 = call "Create new save file.vi"("Insert"="video_frame_" ("string"), "Ext"=".bmp" ("string"), "Index In"="Image Index") -> ("Path Out"=w323:path, "Index Out"=w328:dbl)
                n131 = Increment(x=w328) -> (x+1=w322:dbl)
                n132 = local write "Image Index"(w322) -> ()
                n133 = call <vilib>:"Write BMP File.vi"("image data"=w327, "path to BMP file"=w323) -> ()  [unwired: 1 in, 9 out]
              }
            }
            "GreyscaleArray" <- w204
          }
        }
        n134 = node-c288(w165) -> ()  [unwired: 1 out]
      }
      n135 = node-c288(w149) -> ()  [unwired: 1 out]
      n136 = call "DMR_CloseDevice2.vi"("driver handle IN"=w154) -> ()  [unwired: 3 in, 2 out]
    }
    frame #4 {
      n137 = call "DMR_Close.vi"() -> ()  [unwired: 1 out]
    }
  }
  n138 = while {
    tunnel: [w401] -> w84
    tunnel: [w575] -> w85
    tunnel: [w399] -> w83
    tunnel: [w683] -> w80
    tunnel: w38 -> [w386]
    tunnel: w37 -> [w679]
    tunnel: w36 -> [w684]
    stop <- w683 stop-if-true
    w438 = "NI_ChannelName" ("name")
    w342 = "NI_ChannelName" ("name")
    w503 = -1
    # "Negate these value to make Force feedback work in X. 6-14-18 A.T."
    # "BX - AX"
    # "BY - AY"
    # "Scan # counter"
    # "DAQ loop iteration\ncounter (for timing)"
    # "Step counter"
    # "Force feedback"
    # "Raster scan"
    # "Rewire everything"
    # "Invert these because changed\nfrom PSD to QPD"
    # "Trap Y"
    # "Trap X"
    # "Convert to\npN"
    # "Convert to\nnm"
    # "Subtract\noffset"
    # "Normalize by\nsum"
    # "B sum"
    # "BX"
    # "BY"
    # "AX"
    # "AY"
    # "A sum"
    # "Close files when done saving"
    n139 = disable-structure shown="Disabled" {
      frame Disabled {
        n140 = property class="DAQmx Read"() -> ("AvailSampPerChan"=→"AvailSampPerChan 2":u32)  [unwired: 2 in, 2 out]
      }
      frame Enabled {
      }
    }
    n141 = local read "Averaging Number"() -> (w409:i32)
    n142 = local read "Averaging Number"() -> (w411:i32)
    "# Samples/channel" <- w411
    n143 = local read "Sampling Rate"() -> (w682:dbl)
    n144 = call-poly <vilib>:"DAQmx Read.vi"("task/channels in"=w386, "number of samples per channel"=w409, "timeout"=10.0) -> ("task out"=w385:refnum<k21>, "data"=w410:dbl[][], "error out"=w504:errorcluster)  [unwired: 10 in]
    n145 = Unbundle By Name(w504) -> ("status"=w623:bool)
    n146 = Divide(x=w682, y="Cal Averaging") -> (x/y=→"Cal Final Sampling Rate":dbl)
    n147 = Divide(x=w682, y=w411) -> (x/y=→"Final Sampling Rate" →"# Samples/channel/s":dbl)
    n148 = Index Array(array=w410, index (row)=4) -> (element=w500:dbl[])  [unwired: 1 in]
    n149 = disable-structure shown="Disabled" {
      frame Disabled {
        n150 = local read "Buffer size\n(Samples/channel)"() -> (w701:u32)
        n151 = property class="DAQmx Read"() -> ("AvailSampPerChan"=w702:u32)  [unwired: 2 in, 2 out]
        "AvailSampPerChan" <- w702
        n152 = Divide(x=w702, y=w701) -> (x/y=→"Buffer status":dbl)
      }
      frame Enabled {
      }
    }
    n153 = Index Array(array=w410, index (row)=5) -> (element=w499:dbl[])  [unwired: 1 in]
    n154 = Index Array(array=w410, index (row)=0) -> (element=w361:dbl[])  [unwired: 1 in]
    n155 = Index Array(array=w410, index (row)=3) -> (element=w360:dbl[])  [unwired: 1 in]
    n156 = Index Array(array=w410, index (row)=1) -> (element=w359:dbl[])  [unwired: 1 in]
    n157 = Index Array(array=w410, index (row)=7) -> (element=w357:dbl[])  [unwired: 1 in]
    n158 = Index Array(array=w410, index (row)=2) -> (element=w362:dbl[])  [unwired: 1 in]
    n159 = Index Array(array=w410, index (row)=6) -> (element=w358:dbl[])  [unwired: 1 in]
    n160 = case shown="True" w623 {
      frame False {
      }
      frame True {
        n161 = call <vilib>:"Beep.vi"() -> ()  [unwired: 12 in]
        "Buffer Overflow" <- TRUE
      }
    }
    n162 = Divide(x=w362, y=w358) -> (x/y=w356:dbl[])
    n163 = Divide(x=w361, y=w358) -> (x/y=w355:dbl[])
    n164 = Divide(x=w360, y=w357) -> (x/y=w354:dbl[])
    n165 = Divide(x=w359, y=w357) -> (x/y=w353:dbl[])
    n166 = local read "Cal values"() -> (w615:T2)
    n167 = Build Array(w356, w355, w354, w353) -> (w352:dbl[][])
    n168 = Unbundle(w615) -> ("AX alpha"=w603:dbl, "BX alpha"=w599:dbl, "AX kappa"=w595:dbl, "BX kappa"=w591:dbl, "AX offset"=w609:dbl, "BX offset"=w607:dbl, "AY alpha"=w606:dbl, "BY alpha"=w601:dbl, "AY kappa"=w597:dbl, "BY kappa"=w593:dbl, "AY offset"=w613:dbl, "BY offset"=w611:dbl)
    n169 = Multiply(x=w359, y=w503) -> (x*y=w501:dbl[])
    n170 = Multiply(x=w361, y=w503) -> (x*y=w502:dbl[])
    n171 = local write "AX alpha"(w603) -> ()
    n172 = local write "BY offset"(w611) -> ()
    n173 = Build Array(w502, w362, w501, w360, w358, w357, w500, w499) -> (w435:dbl[][])
    n174 = local write "BX alpha"(w599) -> ()
    n175 = case shown="True" "Reset data stream" {
      selector: "Reset data stream" -> [_ w850]
      tunnel: w385 -> [w842 w848]
      tunnel: [w842 w846] -> w575
      tunnel: w504 -> [w841 w845]
      tunnel: [w841 w843] -> _
      frame False {
      }
      frame True {
        n176 = Not(x=w850) -> (.not. x?=w849:bool)
        n177 = call <vilib>:"DAQmx Stop Task.vi"("task/channels in"=w848, "error in"=w845) -> ("task out"=w847:refnum<k21>, "error out"=w844:errorcluster)  [unwired: 12 in]
        n178 = local write "Reset data stream"(w849) -> ()
        n179 = local write "Buffer Overflow"(w849) -> ()
        n180 = call <vilib>:"DAQmx Start Task.vi"("task/channels in"=w847, "error in"=w844) -> ("task out"=w846:refnum<k21>, "error out"=w843:errorcluster)  [unwired: 12 in]
      }
    }
    n181 = call-poly <vilib>:"Mean.vi"("X"=w499) -> ("mean"=w629:dbl)  [unwired: 1 out]
    n182 = local write "AY offset"(w613) -> ()
    n183 = call-poly <vilib>:"Mean.vi"("X"=w500) -> ("mean"=w630:dbl)  [unwired: 1 out]
    n184 = call-poly <vilib>:"Mean.vi"("X"=w362) -> ("mean"=w636:dbl)  [unwired: 1 out]
    n185 = call-poly <vilib>:"Mean.vi"("X"=w360) -> ("mean"=w634:dbl)  [unwired: 1 out]
    n186 = call-poly <vilib>:"Mean.vi"("X"=w358) -> ("mean"=w633:dbl)  [unwired: 1 out]
    n187 = call-poly <vilib>:"Mean.vi"("X"=w357) -> ("mean"=w632:dbl)  [unwired: 1 out]
    n188 = local read "Averaging Number"() -> (w408:i32)
    n189 = local write "BY kappa"(w593) -> ()
    n190 = local write "AX kappa"(w595) -> ()
    n191 = call-poly <vilib>:"Mean.vi"("X"=w501) -> ("mean"=w635:dbl)  [unwired: 1 out]
    n192 = local write "AY kappa"(w597) -> ()
    n193 = call-poly <vilib>:"Mean.vi"("X"=w502) -> ("mean"=w637:dbl)  [unwired: 1 out]
    n194 = local read "DAQ rate\n(Samples/s)"() -> (w414:dbl)
    n195 = Build Array(w630, w629) -> (w628:dbl[])
    n196 = local write "BX kappa"(w591) -> ()
    n197 = local write "BY alpha"(w601) -> ()
    n198 = local write "AX offset"(w609) -> ()
    n199 = local write "BX offset"(w607) -> ()
    n200 = local write "AY alpha"(w606) -> ()
    n201 = Build Array(w637, w636, w635, w634, w633, w632) -> (w626:dbl[])
    n202 = local read "Total raster time (s)"() -> (w382:dbl)
    n203 = Divide(x=w408, y=w414) -> (x/y=w378:dbl)
    "Data update period (s/set)" <- w378
    n204 = Reciprocal(x=w414) -> (1/x=w415:dbl)
    "Data period (s)" <- w415
    n205 = Divide(x=w382, y=w378) -> (x/y=w381:dbl)
    n206 = Divide(x="Cal time (s)", y=w378) -> (x/y=w377:dbl)
    n207 = Divide(x=w637, y=w633) -> (x/y=w667:dbl)
    n208 = Divide(x=w636, y=w633) -> (x/y=w373:dbl)
    n209 = Round Toward -Infinity(1:w381) -> (0:w380:dbl)
    n210 = Divide(x=w635, y=w632) -> (x/y=w674:dbl)
    n211 = Divide(x=w634, y=w632) -> (x/y=w375:dbl)
    n212 = Round Toward -Infinity(1:w377) -> (0:→"Cal sets to save":dbl)
    n213 = local write "N sets to be saved"(w380) -> ()
    n214 = Build Array("Force Feedback 1", "Force Feedback 2") -> (w338:bool[])
    n215 = Boolean Array To Number(Boolean array=w338) -> (number=w337:u32)
    n216 = Negate(x=w373) -> (-x=w372:dbl)
    n217 = Negate(x=w375) -> (-x=w374:dbl)
    n218 = Subtract(x=w667, y="AY offset") -> (x-y=w649:dbl)
    n219 = Subtract(x=w373, y="AX offset") -> (x-y=w650:dbl)
    n220 = Subtract(x=w674, y="BY offset") -> (x-y=w648:dbl)
    n221 = Subtract(x=w375, y="BX offset") -> (x-y=w651:dbl)
    n222 = Subtract(x=w674, y=w667) -> (x-y=w665:dbl)
    n223 = Subtract(x=w374, y=w372) -> (x-y=w666:dbl)
    n224 = feedback #4(0.0) -> (w574:dbl)
    n225 = Multiply(x="Downsamp\nfact", y=w415) -> (x*y=w350:dbl)
    n226 = Multiply(x=w649, y="AY alpha") -> (x*y=w583:dbl)
    n227 = Multiply(x=w650, y="AX alpha") -> (x*y=w581:dbl)
    n228 = Multiply(x=w651, y="BX alpha") -> (x*y=w582:dbl)
    n229 = Multiply(x=w648, y="BY alpha") -> (x*y=w584:dbl)
    n230 = Add(x=w378, y=w574) -> (x+y=w572:dbl)
    n231 = feedback-in #4(w572) -> ()
    n232 = Square(x=w583) -> (x^2=w659:dbl)
    n233 = Square(x=w581) -> (x^2=w660:dbl)
    n234 = Square(x=w584) -> (x^2=w661:dbl)
    n235 = Square(x=w582) -> (x^2=w662:dbl)
    n236 = Bundle(w665, w666) -> (w369:cluster{dbl, dbl})  [unwired: 1 in]
    n237 = case shown="True" "Set reading to\nsetpoint 1" {
      tunnel: w369 -> [_ w839]
      frame False {
      }
      frame True {
        n238 = property on="Setpoint voltage 1" class="Clust (strict)"("Val(Sgnl)"=w839) -> ()  [unwired: 2 in, 2 out]
        n239 = local read "Trap position (V)"() -> (w838:cluster{"X":dbl, "Y":dbl})
        n240 = local write "Set reading to\nsetpoint 1"(FALSE ("Set reading to\nsetpoint")) -> ()
        n241 = Unbundle(w838) -> ("X"=w837:dbl, "Y"=w836:dbl)
        n242 = Bundle("Y"=w836, "X"=w837) -> (w835:cluster{"Y":dbl, "X":dbl})  [unwired: 1 in]
        n243 = property on="Offset 1" class="Clust (strict)"("Val(Sgnl)"=w835) -> ()  [unwired: 2 in, 2 out]
      }
    }
    n244 = Reciprocal(x=w350) -> (1/x=→"Chart Freq (Hz)":dbl)
    n245 = To Time Stamp(1:w572) -> (0:w349:timestamp)
    n246 = Add(x=w659, y=w660) -> (x+y=w663:dbl)
    n247 = Add(x=w661, y=w662) -> (x+y=w673:dbl)
    n248 = Multiply(x=w581, y="AX kappa") -> (x*y=w577:dbl)
    n249 = Bundle("A y", "A x", "B y", "B x", "A sum", "B sum", "Trap x", "Trap y") -> (w563:T20)  [unwired: 1 in]
    n250 = Multiply(x=w582, y="BX kappa") -> (x*y=w578:dbl)
    n251 = Square Root(x=w663) -> (sqrt(x)=w677:dbl)
    n252 = Square Root(x=w673) -> (sqrt(x)=w676:dbl)
    n253 = Multiply(x=w583, y="AY kappa") -> (x*y=w579:dbl)
    n254 = Multiply(x=w584, y="BY kappa") -> (x*y=w580:dbl)
    n255 = Subtract(x=w629, y="Fixed Y") -> (x-y=w664:dbl)
    n256 = Subtract(x=w630, y="Fixed X") -> (x-y=w668:dbl)
    n257 = Cluster To Array(cluster=w563) -> (array=w562:string[])
    n258 = for {
      tunnel: w435 -> [w828] mode=indexing
      tunnel: w350 -> [w827]
      tunnel: "Downsamp\nfact" -> [w833]
      tunnel: [w831] -> w368 mode=indexing
      tunnel: w349 -> [w834]
      tunnel: w562 -> [w830] mode=indexing
      tunnel: w342 -> [w829]
      n259 = call "Downsample 1D array.vi"("Ave N"=w833, "Arrray In"=w828) -> ("Array Out"=w826:dbl[])  [unwired: 9 in]
      n260 = Bundle By Name("Y"=w826, "dt"=w827, "t0"=w834) -> (w832:waveform(dbl))  [unwired: 1 in]
      n261 = Set Waveform Attribute(5:w830, 6:w829, 7:w832) -> (3:w831:waveform(dbl))  [unwired: 1 in, 2 out]
    }
    "All signals" <- w368
    n262 = Square(x=w579) -> (x^2=w652:dbl)
    n263 = Square(x=w577) -> (x^2=w653:dbl)
    n264 = Square(x=w580) -> (x^2=w654:dbl)
    n265 = Square(x=w578) -> (x^2=w655:dbl)
    n266 = Add(x=w652, y=w653) -> (x+y=w656:dbl)
    n267 = Add(x=w654, y=w655) -> (x+y=w657:dbl)
    n268 = Multiply(x=w664, y="Conv Y (nm/V)") -> (x*y=w586:dbl)
    n269 = Multiply(x=w668, y="Conv X (nm/V)") -> (x*y=w587:dbl)
    n270 = feedback #5() -> (w624:cluster{"B_Y":dbl, "B_X":dbl})  [unwired: 1 in]
    n271 = case shown="1" w337 {
      tunnel: [w1187 w1204 w1214] -> w402
      tunnel: [w1186 w1203 w1215] -> w400
      tunnel: w369 -> [_ w1202 w1217]
      tunnel: [cluster{"B_Y":dbl, "B_X":dbl} {"B_Y"=0.0, "B_X"=0.0} ("Sum error past") w1196 w1212] -> w625
      tunnel: w624 -> [_ w1201 w1213]
      tunnel: w679 -> [w1187 w1199 w1208]
      tunnel: w684 -> [w1186 w1198 w1216]
      tunnel: [0.0 ("B_X") w1191 w1206] -> w335
      tunnel: [cluster{"B_Y":dbl, "B_X":dbl} {"B_Y"=0.0, "B_X"=0.0} ("Sum error past") w1190 w1205] -> w334
      tunnel: "Feedback const" -> [_ w1189 w1207]
      frame 0, Default {
        # "Force feedback"
      }
      frame 1 {
        n272 = local write "Force Feedback 2"(FALSE) -> ()
        n273 = call "ForceFeedback2.vi"("PSD/Mirror Voltages"=w1202, "Sum error"=w1201, "task/channels in"=w1199, "error in"=w1198, "Desired voltage"="Setpoint voltage 1", "Feedback const"=w1189, "offset"="Offset 1") -> ("task out"=w1204:refnum<k21>, "Sum error past"=w1196:cluster{"B_Y":dbl, "B_X":dbl}, "Output Voltage"=w1190:cluster{dbl, dbl}, "error out"=w1203:errorcluster)  [unwired: 8 in, 1 out]
        n274 = local read "Pulling direction"() -> (w1195:bool)
        n275 = Unbundle(w1196) -> ("B_Y"=w1194:dbl, "B_X"=w1193:dbl)
        n276 = Select(t=w1194, s=w1195, f=w1193) -> (s? t:f=w1191:dbl)
      }
      frame 2 {
        n277 = local write "Force Feedback 1"(FALSE) -> ()
        n278 = call "ForceFeedback2.vi"("PSD/Mirror Voltages"=w1217, "Sum error"=w1213, "task/channels in"=w1208, "error in"=w1216, "Desired voltage"="Setpoint voltage 2", "Feedback const"=w1207, "offset"="Offset 2") -> ("task out"=w1214:refnum<k21>, "Sum error past"=w1212:cluster{"B_Y":dbl, "B_X":dbl}, "Output Voltage"=w1205:cluster{dbl, dbl}, "error out"=w1215:errorcluster)  [unwired: 8 in, 1 out]
        n279 = local read "Pulling direction"() -> (w1209:bool)
        n280 = Unbundle(w1212) -> ("B_Y"=w1211:dbl, "B_X"=w1210:dbl)
        n281 = Select(t=w1211, s=w1209, f=w1210) -> (s? t:f=w1206:dbl)
      }
    }
    "Sum error" <- w335
    "Feedback Output \nVoltage 2" <- w334
    n282 = feedback-in #5(w625) -> ()
    n283 = Square Root(x=w656) -> (sqrt(x)=w585:dbl)
    n284 = Square Root(x=w657) -> (sqrt(x)=w678:dbl)
    n285 = Add(x=w585, y=w678) -> (x+y=w658:dbl)
    n286 = case shown="True" "Set reading to\nsetpoint 2" {
      tunnel: w369 -> [_ w696]
      frame False {
      }
      frame True {
        n287 = local read "Trap position (V)"() -> (w699:cluster{"X":dbl, "Y":dbl})
        n288 = property on="Setpoint voltage 2" class="Clust (strict)"("Val(Sgnl)"=w696) -> ()  [unwired: 2 in, 2 out]
        n289 = local write "Set reading to\nsetpoint 2"(FALSE) -> ()
        n290 = Unbundle(w699) -> ("X"=w698:dbl, "Y"=w697:dbl)
        n291 = Bundle("Y"=w697, "X"=w698) -> (w695:cluster{"Y":dbl, "X":dbl})  [unwired: 1 in]
        n292 = property on="Offset 2" class="Clust (strict)"("Val(Sgnl)"=w695) -> ()  [unwired: 2 in, 2 out]
      }
    }
    n293 = Build Array(w667, w373, w674, w375, w633, w632, w585, w678, w677, w676, w587, w586) -> ()  [unwired: 1 out]
    n294 = Divide(x=w658, y=2.0) -> (x/y=w622:dbl)
    n295 = Bundle("AX/Asum", "AY/Asum", "BX/Bsum", "BY/Bsum") -> (w344:cluster{string, string, string, string})  [unwired: 1 in]
    n296 = Index Array(array=w368, index=6) -> (element=w440:waveform(dbl))
    n297 = Index Array(array=w368, index=7) -> (element=w442:waveform(dbl))
    n298 = Cluster To Array(cluster=w344) -> (array=w343:string[])
    n299 = for {
      tunnel: w352 -> [w694] mode=indexing
      tunnel: "Downsamp\nfact" -> [w693]
      tunnel: w350 -> [w692]
      tunnel: w349 -> [w690]
      tunnel: w343 -> [w688] mode=indexing
      tunnel: w342 -> [w687]
      tunnel: [w686] -> w341 mode=indexing
      n300 = call "Downsample 1D array.vi"("Ave N"=w693, "Arrray In"=w694) -> ("Array Out"=w691:dbl[])  [unwired: 9 in]
      n301 = Bundle By Name("Y"=w691, "dt"=w692, "t0"=w690) -> (w689:waveform(dbl))  [unwired: 1 in]
      n302 = Set Waveform Attribute(5:w688, 6:w687, 7:w689) -> (3:w686:waveform(dbl))  [unwired: 1 in, 2 out]
    }
    "All signals 2" <- w341
    n303 = local read "Fixed X"() -> (w489:dbl)
    n304 = local read "Fixed Y"() -> (w491:dbl)
    n305 = Unbundle By Name(w440) -> ("Y"=w493:dbl[])
    n306 = Unbundle By Name(w442) -> ("Y"=w492:dbl[])
    n307 = Index Array(array=w368, index=0) -> (element=w447:waveform(dbl))
    n308 = Index Array(array=w368, index=1) -> (element=w559:waveform(dbl))
    n309 = Index Array(array=w368, index=4) -> (element=w553:waveform(dbl))
    n310 = Subtract(x=w493, y=w489) -> (x-y=w490:dbl[])
    n311 = Subtract(x=w492, y=w491) -> (x-y=w487:dbl[])
    n312 = Unbundle By Name(w447) -> ("Y"=w551:dbl[])
    n313 = Unbundle By Name(w559) -> ("Y"=w550:dbl[])
    n314 = Unbundle By Name(w553) -> ("Y"=w549:dbl[])
    n315 = Index Array(array=w368, index=5) -> (element=w552:waveform(dbl))
    n316 = local read "Conv X (nm/V)"() -> (w488:dbl)
    n317 = local read "Conv Y (nm/V)"() -> (w486:dbl)
    n318 = Index Array(array=w368, index=2) -> (element=w363:waveform(dbl))
    n319 = Index Array(array=w368, index=3) -> (element=w556:waveform(dbl))
    n320 = Set Waveform Attribute(5:"T2 X", 6:w438, 7:w440) -> (3:w439:waveform(dbl))  [unwired: 1 in, 2 out]
    n321 = Set Waveform Attribute(5:"T2 Y", 6:w438, 7:w442) -> (3:w441:waveform(dbl))  [unwired: 1 in, 2 out]
    n322 = Unbundle By Name(w552) -> ("Y"=w546:dbl[])
    n323 = Unbundle By Name(w363) -> ("Y"=w548:dbl[])
    n324 = Unbundle By Name(w556) -> ("Y"=w547:dbl[])
    n325 = Divide(x=w551, y=w549) -> (x/y=w367:dbl[])
    n326 = Divide(x=w550, y=w549) -> (x/y=w366:dbl[])
    n327 = local read "AY offset"() -> (w537:dbl)
    n328 = local read "AX offset"() -> (w535:dbl)
    n329 = Multiply(x=w490, y=w488) -> (x*y=w432:dbl[])
    n330 = Multiply(x=w487, y=w486) -> (x*y=w434:dbl[])
    n331 = Divide(x=w547, y=w546) -> (x/y=w364:dbl[])
    n332 = Subtract(x=w366, y=w535) -> (x-y=w538:dbl[])
    n333 = local read "BX offset"() -> (w545:dbl)
    n334 = Subtract(x=w367, y=w537) -> (x-y=w539:dbl[])
    n335 = Divide(x=w548, y=w546) -> (x/y=w365:dbl[])
    n336 = local read "AY alpha"() -> (w536:dbl)
    n337 = local read "AX alpha"() -> (w534:dbl)
    n338 = call-poly <vilib>:"Mean.vi"("X"=w434) -> ("mean"=w469:dbl)  [unwired: 1 out]
    "Mean Trp Pos Y 2 (nm)" <- w469
    n339 = Subtract(x=w365, y=w367) -> (x-y=w459:dbl[])
    n340 = Subtract(x=w364, y=w366) -> (x-y=w458:dbl[])
    n341 = local read "BY offset"() -> (w542:dbl)
    n342 = Subtract(x=w432, y="Offset X (nm)") -> (x-y=w431:dbl[])
    n343 = Subtract(x=w434, y="Offset Y (nm)") -> (x-y=w433:dbl[])
    n344 = Subtract(x=w365, y=w542) -> (x-y=w544:dbl[])
    n345 = Subtract(x=w364, y=w545) -> (x-y=w543:dbl[])
    n346 = Subtract(x=w469, y=w434) -> (x-y=w468:dbl[])
    n347 = call-poly <vilib>:"Mean.vi"("X"=w432) -> ("mean"=w473:dbl)  [unwired: 1 out]
    "Mean Trap Pos X 2 (nm)" <- w473
    n348 = Build Array(w459, w458) -> (w456:dbl[][])
    n349 = Index Array(array=w456, index (row)=0) -> (element=w454:dbl[])  [unwired: 1 in]
    n350 = Index Array(array=w456, index (row)=1) -> (element=w453:dbl[])  [unwired: 1 in]
    n351 = call-poly <vilib>:"Mean.vi"("X"=w454) -> ("mean"=w452:dbl)  [unwired: 1 out]
    n352 = call-poly <vilib>:"Mean.vi"("X"=w453) -> ("mean"=w451:dbl)  [unwired: 1 out]
    n353 = Bundle("mean"=w452, "mean"=w451) -> ()  [unwired: 1 in, 1 out]
    n354 = local read "BX alpha"() -> (w540:dbl)
    n355 = Multiply(x=w539, y=w536) -> (x*y=w527:dbl[])
    n356 = Multiply(x=w538, y=w534) -> (x*y=w526:dbl[])
    n357 = Square(x=w468) -> (x^2=w467:dbl[])
    n358 = Subtract(x=w473, y=w432) -> (x-y=w472:dbl[])
    n359 = Bundle By Name(cluster=w441, "Y"=w433) -> (w484:waveform(dbl))
    n360 = Bundle By Name(cluster=w439, "Y"=w431) -> (w485:waveform(dbl))
    n361 = local read "BY alpha"() -> (w541:dbl)
    n362 = local read "Raster scanning..."() -> (w384:bool)
    n363 = local read "Saving"() -> (w588:bool)
    n364 = local read "Tether"() -> (w589:bool)
    n365 = Square(x=w472) -> (x^2=w471:dbl[])
    n366 = call-poly <vilib>:"Mean.vi"("X"=w467) -> ("mean"=w466:dbl)  [unwired: 1 out]
    n367 = Square(x=w527) -> (x^2=w533:dbl[])
    n368 = Multiply(x=w544, y=w541) -> (x*y=w525:dbl[])
    n369 = Square(x=w526) -> (x^2=w532:dbl[])
    n370 = Multiply(x=w543, y=w540) -> (x*y=w524:dbl[])
    n371 = Less?(x=w622, y="Tether break\nforce (pN)") -> (x < y?=w620:bool)
    n372 = call-poly <vilib>:"Mean.vi"("X"=w471) -> ("mean"=w470:dbl)  [unwired: 1 out]
    n373 = Build Array(w485, w484) -> (w403:waveform(dbl)[])
    "Trap sep" <- w403
    n374 = Square Root(x=w466) -> (sqrt(x)=w465:dbl)
    n375 = Square(x=w525) -> (x^2=w531:dbl[])
    n376 = Square(x=w524) -> (x^2=w530:dbl[])
    n377 = Add(x=w533, y=w532) -> (x+y=w529:dbl[])
    n378 = Square Root(x=w470) -> (sqrt(x)=w463:dbl)
    n379 = Compound Arithmetic op=AND(w588, w589, w620) -> (w619:bool)
    n380 = Multiply(x=w465, y=10) -> (x*y=→"T2 Y RMS (A)":dbl)
    n381 = Square Root(x=w529) -> (sqrt(x)=w427:dbl[])
    n382 = Add(x=w531, y=w530) -> (x+y=w528:dbl[])
    n383 = Set Waveform Attribute(5:"T2", 6:"NI_ChannelName" ("name"), 7:w447) -> (3:w446:waveform(dbl))  [unwired: 1 in, 2 out]
    n384 = Set Waveform Attribute(5:"T1", 6:"NI_ChannelName" ("name"), 7:w363) -> (3:w444:waveform(dbl))  [unwired: 1 in, 2 out]
    n385 = case shown="True" w619 {
      selector: w619 -> [_ w857]
      tunnel: w384 -> [w851 w853]
      tunnel: [w851 w853] -> w383
      frame False {
      }
      frame True {
        n386 = flat-sequence {
          frame #0 {
            n387 = local write "Cancel Rep\n Dip"(TRUE) -> ()
          }
          frame #1 {
            n388 = local write "Cancel Rep\n Dip"(FALSE ("Cancel Rep\n Dip")) -> ()
          }
        }
        n389 = call <vilib>:"Beep.vi"() -> ()  [unwired: 12 in]
        n390 = Not(x=w857) -> (.not. x?=w852:bool)
        n391 = And(x=w853, y="Fish After TA?") -> (x .and. y?=w855:bool)
        n392 = local write "Force Feedback 1"(w852) -> ()
        n393 = local write "Tether"(w852) -> ()
        n394 = case shown="True" w855 {
          selector: w855 -> [_ w860]
          frame False {
          }
          frame True {
            n395 = property on="Fish" class="Bool (strict)"("Val(Sgnl)"=w860) -> ()  [unwired: 2 in, 2 out]
          }
        }
        n396 = local write "Force Feedback 2"(w852) -> ()
        n397 = property on="Stop saving" class="Bool (strict)"("Val(Sgnl)"="TA Cancel Save?") -> ()  [unwired: 2 in, 2 out]
      }
    }
    n398 = Square Root(x=w528) -> (sqrt(x)=w426:dbl[])
    n399 = Multiply(x=w463, y=10) -> (x*y=→"T2 X RMS (A)":dbl)
    n400 = Bundle By Name(cluster=w446, "Y"=w427) -> (w450:waveform(dbl))
    n401 = Bundle By Name(cluster=w444, "Y"=w426) -> (w506:waveform(dbl))
    n402 = Add(x=w427, y=w426) -> (x+y=w425:dbl[])
    n403 = case shown="True" "Remove offsets" {
      selector: "Remove offsets" -> [_ w824]
      frame False {
      }
      frame True {
        n404 = local read "Mean Trp Pos Y 2 (nm)"() -> (w822:dbl)
        n405 = Not(x=w824) -> (.not. x?=w825:bool)
        n406 = local read "Mean Trap Pos X 2 (nm)"() -> (w823:dbl)
        n407 = local write "Remove offsets"(w825) -> ()
        n408 = local write "Offset Y (nm)"(w822) -> ()
        n409 = local write "Offset X (nm)"(w823) -> ()
      }
    }
    n410 = Build Array(w450, w506) -> (→"Bead sep":waveform(dbl)[])
    n411 = local read "AY kappa"() -> (w523:dbl)
    n412 = local read "AX kappa"() -> (w522:dbl)
    n413 = Divide(x=w425, y=2) -> (x/y=w423:dbl[])
    n414 = local read "BX kappa"() -> (w520:dbl)
    n415 = local read "BY kappa"() -> (w521:dbl)
    n416 = call-poly <vilib>:"Mean.vi"("X"=w423) -> ("mean"=w422:dbl)  [unwired: 1 out]
    "Mean Bead Sep\n(nm)" <- w422
    n417 = local read "Calibrating"() -> (w336:bool)
    n418 = Multiply(x=w527, y=w523) -> (x*y=w516:dbl[])
    n419 = Multiply(x=w526, y=w522) -> (x*y=w517:dbl[])
    n420 = Square(x=w516) -> (x^2=w515:dbl[])
    n421 = Square(x=w517) -> (x^2=w514:dbl[])
    n422 = Subtract(x=w423, y=w422) -> (x-y=w421:dbl[])
    n423 = Multiply(x=w525, y=w521) -> (x*y=w518:dbl[])
    n424 = Multiply(x=w524, y=w520) -> (x*y=w519:dbl[])
    n425 = Or(x=w383, y="Raster scan") -> (x .or. y?=w398:bool)
    n426 = Add(x=w515, y=w514) -> (x+y=w511:dbl[])
    n427 = Square(x=w421) -> (x^2=w420:dbl[])
    n428 = Square Root(x=w511) -> (sqrt(x)=w483:dbl[])
    n429 = Square(x=w518) -> (x^2=w513:dbl[])
    n430 = Square(x=w519) -> (x^2=w512:dbl[])
    n431 = call-poly <vilib>:"Mean.vi"("X"=w420) -> ("mean"=w419:dbl)  [unwired: 1 out]
    n432 = Add(x=w513, y=w512) -> (x+y=w510:dbl[])
    n433 = Bundle By Name(cluster=w446, "Y"=w483) -> (w509:waveform(dbl))
    n434 = local read "Saving"() -> (w618:bool)
    n435 = Or(x=w336, y=w618) -> ()  [unwired: 1 out]
    n436 = Square Root(x=w419) -> (sqrt(x)=w418:dbl)
    n437 = Square Root(x=w510) -> (sqrt(x)=w482:dbl[])
    n438 = Multiply(x=10, y=w418) -> (x*y=→"Bead Sep Noise\n(A)":dbl)
    n439 = Bundle By Name(cluster=w444, "Y"=w482) -> (w508:waveform(dbl))
    n440 = Add(x=w483, y=w482) -> (x+y=w481:dbl[])
    n441 = Build Array(w509, w508) -> (→"Force (pN)":waveform(dbl)[])
    n442 = Divide(x=w481, y=2) -> (x/y=w478:dbl[])
    n443 = call-poly <vilib>:"Mean.vi"("X"=w478) -> ("mean"=w479:dbl)  [unwired: 1 out]
    "Mean force (pN)" <- w479
    n444 = Subtract(x=w479, y=w478) -> (x-y=w477:dbl[])
    n445 = Square(x=w477) -> (x^2=w476:dbl[])
    n446 = call-poly <vilib>:"Mean.vi"("X"=w476) -> ("mean"=w475:dbl)  [unwired: 1 out]
    n447 = flat-sequence {
      tunnel: w336 -> [w903]
      tunnel: w618 -> [_]
      tunnel: w336 -> [_]
      tunnel: w618 -> [_]
      tunnel: w435 -> [w890]
      tunnel: [w890] -> w639
      tunnel: w504 -> [w889]
      tunnel: [w889] -> w638
      tunnel: w626 -> [w888]
      tunnel: [w888] -> w631
      tunnel: w628 -> [w887]
      tunnel: [w887] -> w627
      tunnel: [w884] -> w617
      tunnel: [w881] -> w616
      tunnel: [w878] -> w498
      tunnel: [w877] -> w497
      tunnel: [w874] -> w496
      tunnel: w405 -> [w871]
      tunnel: ["Save Data"] -> w404
      tunnel: [w864] -> w371
      tunnel: w639 -> [w1084]
      tunnel: w638 -> [w1083]
      tunnel: w631 -> [_]
      tunnel: w627 -> [_]
      tunnel: w617 -> [w1082]
      tunnel: w616 -> [w1081]
      tunnel: w498 -> [w1080]
      tunnel: w497 -> [w1079]
      tunnel: w496 -> [w1078]
      tunnel: w404 -> [w1077]
      tunnel: w403 -> [w1076]
      tunnel: w371 -> [w1074]
      frame #0 {
        w870 = 0.0
        # "1: old trap\n0: fleezers"
        # "Create files if saving data"
        n448 = local read "Save N sets"() -> (w873:bool)
        n449 = local read "Fixed X"() -> (w869:dbl)
        n450 = local read "Trap position (V)"() -> (w898:cluster{"X":dbl, "Y":dbl})
        n451 = local read "Fixed Y"() -> (w868:dbl)
        n452 = local read "Sampling Rate"() -> (w901:dbl)
        n453 = Or(x=w873, y="Save Data") -> (x .or. y?=w872:bool)
        n454 = Build Array(w872, "Save cal", w871) -> (w892:bool[])
        n455 = Compound Arithmetic op=OR("Save Data", "Save cal", w871) -> (w894:bool)
        n456 = Boolean Array To Number(Boolean array=w892) -> (number=w891:u32)
        n457 = Unbundle(w898) -> ("X"=w867:dbl, "Y"=w866:dbl)
        n458 = Build Array(w867, w866, w869, w868, w870, w870) -> (w897:dbl[])
        n459 = feedback #6(refnum<k0> refnum) -> (w863:refnum<file>)
        n460 = feedback #7(0) -> (w895:i32)
        n461 = feedback #8(refnum<k0> refnum) -> (w885:refnum<file>)
        n462 = feedback #9() -> (w879:dbl)  [unwired: 1 in]
        n463 = feedback #10(FALSE) -> (w875:bool)
        n464 = feedback #11(refnum<k0> refnum) -> (w882:refnum<file>)
        n465 = case shown="True" w894 {
          tunnel: w903 -> [_ _]
          tunnel: 9 -> [_ w949]
          tunnel: w901 -> [_ w948]
          tunnel: 6 -> [_ w947]
          tunnel: 5 -> [_ w946]
          tunnel: w897 -> [_ w945]
          tunnel: [w909 1] -> w878
          tunnel: w895 -> [w910 _]
          tunnel: w891 -> [_ w921]
          tunnel: [w908 w920] -> w884
          tunnel: w885 -> [w908 _]
          tunnel: [w907 w919] -> w881
          tunnel: w882 -> [w907 _]
          tunnel: 1.0 -> [_ w918]
          tunnel: [w906 w917] -> w877
          tunnel: w879 -> [w906 _]
          tunnel: [w905 w916] -> w874
          tunnel: w875 -> [w905 _]
          tunnel: [w904 w911] -> w864
          tunnel: w863 -> [w904 _]
          frame False {
            n466 = Increment(x=w910) -> (x+1=w909:i32)
          }
          frame True {
            w922 = FALSE ("Save Data")
            w927 = FALSE
            w928 = T19."big-endian, network order" ("byte order (0:big-endian, network order)")
            n467 = local write "Save cal"(w922) -> ()
            n468 = local write "Save Data"(w922) -> ()
            n469 = case shown="4" w921 {
              tunnel: w949 -> [w1024 w1042 w1073]
              tunnel: w948 -> [w1003 w1041 w1050]
              tunnel: w947 -> [w1023 w1039 w1069]
              tunnel: w946 -> [w1022 w1038 w1068]
              tunnel: w945 -> [w1021 w1035 w1065]
              tunnel: [w1020 w1034 w1054] -> w942
              tunnel: [w1001 w1025 w1045] -> w916
              tunnel: ["Averaging Number" 200 w1052] -> _
              tunnel: w918 -> [w1008 w1027 w1051]
              tunnel: [w1004 w1026 w1046] -> w917
              tunnel: [w1001 w1025 w1044] -> w913
              frame 1, Default {
                w1001 = TRUE
                w1009 = 0.0
                # "stage x,yz"
                # "Save N number/length of data. e.g. N =200 \nwill give only 200 long data points"
                # "Time trace"
                n470 = Boolean To (0,1)(Boolean=w1001) -> (0, 1=w1014:i16)
                n471 = local read "Averaging Number"() -> (w1019:i32)
                n472 = Increment(x=w1014) -> (x+1=w1013:i16)
                n473 = Divide(x=w1003, y=w1019) -> (x/y=w1018:dbl)
                n474 = To Double Precision Float(number=w1013) -> (double precision float=w1012:dbl)
                n475 = Reciprocal(x=w1018) -> (1/x=w1017:dbl)
                n476 = Reciprocal(x=w1003) -> (1/x=w1002:dbl)
                n477 = Build Array(w1024, w1002, w1017, w1023, w1022, 0 ("f")) -> (w1016:dbl[])
                n478 = Build Array(w1012, w1008, w1009, w1009, w1009) -> (w1015:dbl[])
                n479 = Build Array (concatenate)(w1016, w1021, w1015) -> (w1020:dbl[])
                n480 = Select(t="N sets", s="Save N sets", f=2147483647) -> (s? t:f=w1004:i32)
              }
              frame 2 {
                w1025 = FALSE
                w1030 = 0.0
                # "Calibration file"
                n481 = Reciprocal(x=w1041) -> (1/x=w1040:dbl)
                n482 = Boolean To (0,1)(Boolean=w1025) -> (0, 1=w1033:i16)
                n483 = To Double Precision Float(number=w1033) -> (double precision float=w1032:dbl)
                n484 = Build Array(w1042, w1040, w1040, w1039, w1038, 1) -> (w1036:dbl[])
                n485 = Build Array(w1032, w1027, w1030, w1030, w1030) -> (w1031:dbl[])
                n486 = Build Array (concatenate)(w1036, w1035, w1031) -> (w1034:dbl[])
                n487 = local read "Cal sets to save"() -> (w1026:i32)
                "Calibrating" <- TRUE ("Calibrating")
              }
              frame 4 {
                w1043 = FALSE ("Raster scan")
                w1061 = 0.0
                w1045 = TRUE
                # "Not using ncycles"
                # "FX curve"
                n488 = Not(x=w1045) -> (.not. x?=w1044:bool)
                n489 = local read "Averaging Number"() -> (w1072:i32)
                n490 = Boolean To (0,1)(Boolean=w1045) -> (0, 1=w1064:i16)
                n491 = local write "Saving Move"(w1043) -> ()
                n492 = Divide(x=w1050, y=w1072) -> (x/y=w1071:dbl)
                n493 = Increment(x=w1064) -> (x+1=w1063:i16)
                n494 = local write "Raster scan"(w1043) -> ()
                n495 = To Double Precision Float(number=w1063) -> (double precision float=w1062:dbl)
                n496 = Reciprocal(x=w1071) -> (1/x=w1070:dbl)
                n497 = Reciprocal(x=w1050) -> (1/x=w1049:dbl)
                n498 = Build Array(w1062, w1051, w1061, w1061, w1061) -> (w1060:dbl[])
                n499 = Build Array(w1073, w1049, w1070, w1069, w1068, 2) -> (w1066:dbl[])
                n500 = local read "Scan range (V)"() -> (w1047:dbl)
                n501 = local read "Pulling direction"() -> (w1058:bool)
                n502 = local read "Scan steps (mirror)"() -> (w1048:u64)
                n503 = local read "# scans"() -> (w1056:i32)
                n504 = local read "N sets to be saved"() -> (w1046:dbl)
                n505 = Not(x=w1058) -> (.not. x?=w1057:bool)
                n506 = local read "Averaging Number"() -> (w1052:i32)
                n507 = Boolean To (0,1)(Boolean=w1057) -> (0, 1=w1059:i16)
                n508 = Build Array(w1059, w1047, w1048, 0, w1056) -> (w1055:dbl[])
                n509 = Build Array (concatenate)(w1066, w1065, w1060, w1055) -> (w1054:dbl[])
              }
            }
            n510 = call "CreateSaveFile.vi"("Index In"="Save file index", "Ext"=".dat", "Insert"="", "Directory"="Path") -> ("Index Out"=w915:i32, "Path Out"=w912:path)  [unwired: 6 in]
            "Current file name" <- w912
            n511 = case shown="True" w913 {
              tunnel: w912 -> [_ w961]
              tunnel: [refnum<k0> refnum w958] -> w911
              frame False {
              }
              frame True {
                # "SY 190201 \nAdding functionality to get time points of start and stop moves. \nWehn timetrace save data starts save time point"
                n512 = Path To String(path=w961) -> (string=w965:string)
                n513 = Get Date/Time In Seconds() -> (seconds since 1Jan1904=w975:timestamp)
                n514 = String Length(string=w965) -> (length=w962:i32)
                n515 = Subtract(x=w962, y=4) -> (x-y=w964:i32)
                n516 = Format Date/Time String(time format string (%c)="%H:%M:%S%3u", seconds (now)=w975, UTC format=TRUE) -> (date/time string=w959:string)
                n517 = call <vilib>:"Space Constant.vi"() -> ("String"=w953:string)
                n518 = String Subset(string=w965, length (rest)=w964) -> (substring=w966:string)  [unwired: 1 in]
                n519 = Concatenate Strings(w966, "_stagetime.txt" ("string")) -> (w968:string)
                n520 = String To Path(string=w968) -> (path=w969:path)
                n521 = Open/Create/Replace File(file path (use dialog)=w969, operation (0:open)=T18."create", access (0:read/write)=enum16{"read/write", "read-only", "write-only"}."write-only") -> (refnum out=w973:refnum<file>, error out=w972:errorcluster)  [unwired: 3 in, 1 out]
                n522 = Deny Access(4:w972, 7:w973) -> (3:w974:refnum<file>)  [unwired: 1 in, 1 out]
                n523 = Concatenate Strings(w959, w953, "start", "\r\n") -> (w960:string)
                n524 = Write to Text File(file (use dialog)=w974, text=w960) -> (refnum out=w958:refnum<file>)  [unwired: 2 in, 2 out]
                n525 = local write "Move time"(w959) -> ()
                n526 = local read "Raster scanning..."() -> (w956:bool)
                n527 = local read "Calibrating"() -> (w957:bool)
                n528 = Or(x=w957, y=w956) -> (x .or. y?=w955:bool)
                n529 = Not(x=w955) -> (.not. x?=w954:bool)
                n530 = local write "Saving Move"(w954) -> ()
              }
            }
            n531 = Open/Create/Replace File(file path (use dialog)=w912, operation (0:open)=T18."create", access (0:read/write)=enum16{"read/write", "read-only", "write-only"}."write-only") -> (refnum out=w935:refnum<file>, error out=w936:errorcluster)  [unwired: 3 in, 1 out]
            n532 = local write "Save file index"(w915) -> ()
            n533 = Array Size(array=w942) -> (size(s)=w944:i32)
            n534 = case shown="True" w916 {
              tunnel: w912 -> [_ w1000]
              tunnel: [refnum<k0> refnum w979] -> w919
              frame False {
              }
              frame True {
                w986 = 0.0
                n535 = Path To String(path=w1000) -> (string=w996:string)
                n536 = Build Array(w986, w986, w986, w986, w986, w986, w986, w986) -> (w983:dbl[])
                n537 = String Length(string=w996) -> (length=w999:i32)
                n538 = Array Size(array=w983) -> (size(s)=w985:i32)
                n539 = Subtract(x=w999, y=4) -> (x-y=w997:i32)
                n540 = To Double Precision Float(number=w985) -> (double precision float=w984:dbl)
                n541 = String Subset(string=w996, length (rest)=w997) -> (substring=w995:string)  [unwired: 1 in]
                n542 = Build Array (concatenate)(w984, w983) -> (w982:dbl[])
                n543 = Concatenate Strings(w995, "_pos.dat" ("string")) -> (w993:string)
                n544 = String To Path(string=w993) -> (path=w992:path)
                n545 = Open/Create/Replace File(file path (use dialog)=w992, operation (0:open)=T18."create", access (0:read/write)=enum16{"read/write", "read-only", "write-only"}."write-only") -> (refnum out=w988:refnum<file>, error out=w989:errorcluster)  [unwired: 3 in, 1 out]
                n546 = Deny Access(4:w989, 7:w988) -> (3:w987:refnum<file>)  [unwired: 1 in, 1 out]
                n547 = Write to Binary File(file (use dialog)=w987, data=w982, 5:FALSE ("prepend array or string size? (T)"), 9:T19."big-endian, network order" ("byte order (0:big-endian, network order)")) -> (refnum out=w979:refnum<file>)  [unwired: 2 in, 2 out]
              }
            }
            n548 = Deny Access(4:w936, 7:w935) -> (0:w926:errorcluster, 3:w934:refnum<file>)  [unwired: 1 in]
            n549 = String Length(string="Comment") -> (length=w941:i32)
            n550 = To Double Precision Float(number=w944) -> (double precision float=w943:dbl)
            n551 = To Double Precision Float(number=w941) -> (double precision float=w940:dbl)
            n552 = Build Array (concatenate)(w943, w942, w940) -> (w931:dbl[])
            n553 = Write to Binary File(file (use dialog)=w934, data=w931, error in=w926, 5:w927, 9:w928) -> (refnum out=w930:refnum<file>, error out=w925:errorcluster)  [unwired: 1 in, 1 out]
            n554 = Write to Binary File(file (use dialog)=w930, data="Comment", error in=w925, 5:w927, 9:w928) -> (refnum out=w920:refnum<file>)  [unwired: 1 in, 2 out]
            "Saving" <- TRUE
          }
        }
        n555 = feedback-in #6(w864) -> ()
        n556 = feedback-in #7(w878) -> ()
        n557 = feedback-in #8(w884) -> ()
        n558 = feedback-in #9(w877) -> ()
        n559 = feedback-in #10(w874) -> ()
        n560 = feedback-in #11(w881) -> ()
      }
      frame #1 {
        n561 = local read "Saving"() -> (w1075:bool)
        n562 = case shown="True" w1075 {
          tunnel: w1084 -> [_ w1104]
          tunnel: w1083 -> [_ w1103]
          tunnel: w1082 -> [_ w1102]
          tunnel: w1081 -> [_ w1101]
          tunnel: w1080 -> [_ w1092]
          tunnel: w1079 -> [_ w1093]
          tunnel: w1078 -> [_ w1096]
          tunnel: w1077 -> [_ w1088]
          tunnel: w1076 -> [_ w1087]
          tunnel: w1074 -> [_ w1085]
          frame False {
            (unwired) FALSE ("Calibrating")
          }
          frame True {
            n563 = local read "Stop"() -> (w1099:bool)
            n564 = Less Or Equal?(x=w1092, y=w1093) -> (x <= y?=w1100:bool)
            n565 = Divide(x=w1092, y=w1093) -> (x/y=w1091:dbl)
            n566 = Or(x=w1099, y="Stop saving") -> (x .or. y?=w1086:bool)
            n567 = Multiply(x=100.0, y=w1091) -> (x*y=w1090:dbl)
            n568 = Not(x=w1086) -> (.not. x?=w1098:bool)
            n569 = And(x=w1100, y=w1098) -> (x .and. y?=w1097:bool)
            n570 = case shown="False" w1097 {
              tunnel: w1102 -> [w1109 w1134]
              tunnel: w1103 -> [_ w1133]
              tunnel: w1104 -> [_ w1132]
              tunnel: w1101 -> [w1108 w1131]
              tunnel: w1096 -> [w1105 _]
              tunnel: [0.0 ("Progress") w1130] -> w1095
              tunnel: w1090 -> [_ w1130]
              tunnel: w1088 -> [_ _]
              tunnel: w1087 -> [_ w1129]
              tunnel: w1085 -> [w1106 w1126]
              frame False {
                n571 = flat-sequence {
                  tunnel: w1109 -> [w1114]
                  tunnel: w1108 -> [w1113]
                  tunnel: w1106 -> [w1112]
                  tunnel: w1105 -> [w1111]
                  frame #0 {
                    n572 = local read "Saving Move"() -> (w1110:bool)
                    n573 = case shown="True" w1111 {
                      tunnel: w1113 -> [_ w1124]
                      frame False {
                      }
                      frame True {
                        n574 = Close File(refnum=w1124) -> ()  [unwired: 1 in, 2 out]
                      }
                    }
                    n575 = case shown="True" w1110 {
                      tunnel: w1112 -> [_ w1119]
                      frame False {
                      }
                      frame True {
                        n576 = Get Date/Time In Seconds() -> (seconds since 1Jan1904=w1123:timestamp)
                        n577 = call <vilib>:"Space Constant.vi"() -> ("String"=w1118:string)
                        n578 = Format Date/Time String(time format string (%c)="%H:%M:%S%3u", seconds (now)=w1123, UTC format=TRUE) -> (date/time string=w1116:string)
                        n579 = Concatenate Strings(w1116, w1118, "end") -> (w1115:string)
                        n580 = Write to Text File(file (use dialog)=w1119, text=w1115) -> (refnum out=w1120:refnum<file>)  [unwired: 2 in, 2 out]
                        n581 = Close File(refnum=w1120) -> ()  [unwired: 1 in, 2 out]
                        n582 = local write "Move time"(w1116) -> ()
                      }
                    }
                    n583 = Close File(refnum=w1114) -> ()  [unwired: 1 in, 2 out]
                  }
                  frame #1 {
                    w1125 = FALSE
                    n584 = local write "Saving"(w1125) -> ()
                    n585 = local write "Stop saving"(w1125) -> ()
                    n586 = local write "Saving Move"(w1125) -> ()
                    n587 = local write "Calibrating"(w1125) -> ()
                    n588 = call <vilib>:"Beep.vi"() -> ()  [unwired: 12 in]
                  }
                }
              }
              frame True {
                n589 = local read "Calibrating"() -> (w1128:bool)
                n590 = local read "Saving Move"() -> (w1127:bool)
                n591 = case shown="False" w1128 {
                  tunnel: w1134 -> [w1167 w1183]
                  tunnel: w1133 -> [_ w1182]
                  tunnel: w1132 -> [w1154 w1176]
                  tunnel: w1131 -> [w1153 _]
                  tunnel: w1129 -> [w1145 _]
                  frame False {
                    n592 = local read "Averaging Number"() -> (w1161:i32)
                    n593 = Array Subset(array=w1154, index (row)=0 ("index"), length (row)=6 ("length")) -> (w1150:dbl[][])  [unwired: 2 in]
                    n594 = Array Subset(array=w1154, index (row)=6 ("index"), length (row)=2 ("length")) -> (w1149:dbl[][])  [unwired: 2 in]
                    n595 = Array Size(array=w1149) -> (size(s)=w1160:i32[])
                    n596 = Array Size(array=w1150) -> (size(s)=w1157:i32[])
                    n597 = Index Array(array=w1145, index=0) -> (element=w1142:waveform(dbl))
                    n598 = Index Array(array=w1145, index=1) -> (element=w1141:waveform(dbl))
                    n599 = for {
                      tunnel: w1150 -> [w1171] mode=indexing
                      tunnel: w1161 -> [w1173]
                      tunnel: [w1172] -> w1148 mode=indexing
                      n600 = call "Downsample 1D array.vi"("Ave N"=w1173, "Arrray In"=w1171) -> ("Array Out"=w1172:dbl[])  [unwired: 9 in]
                    }
                    n601 = Unbundle By Name(w1142) -> ()  [unwired: 1 out]
                    n602 = Unbundle By Name(w1141) -> ()  [unwired: 1 out]
                    n603 = Multiply Array Elements(1:w1157) -> (0:w1156:i32)
                    n604 = for {
                      tunnel: w1149 -> [w1170] mode=indexing
                      tunnel: w1161 -> [w1169]
                      tunnel: [w1168] -> w1152 mode=indexing
                      n605 = call "Downsample 1D array.vi"("Ave N"=w1169, "Arrray In"=w1170) -> ("Array Out"=w1168:dbl[])  [unwired: 9 in]
                    }
                    n606 = Multiply Array Elements(1:w1160) -> (0:w1159:i32)
                    n607 = Divide(x=w1156, y=w1161) -> (x/y=w1162:dbl)
                    n608 = Divide(x=w1159, y=w1161) -> (x/y=w1158:dbl)
                    n609 = Transpose 2D Array(2D array=w1148) -> (transposed array=w1147:dbl[][])
                    n610 = Transpose 2D Array(2D array=w1152) -> (transposed array=w1146:dbl[][])
                    n611 = Reshape Array(w1147, w1162) -> (w1151:dbl[])
                    n612 = Reshape Array(w1146, w1158) -> (w1155:dbl[])
                    n613 = call <vilib>:"Write File+ [SGL].vi"("1D array"=w1155, "refnum"=w1153) -> ()  [unwired: 7 in, 3 out]
                    n614 = call <vilib>:"Write File+ [SGL].vi"("1D array"=w1151, "refnum"=w1167) -> ()  [unwired: 7 in, 3 out]
                  }
                  frame True {
                    n615 = Array Subset(array=w1176, index (row)=0 ("index"), length (row)=6 ("length")) -> (w1174:dbl[][])  [unwired: 2 in]
                    n616 = Transpose 2D Array(2D array=w1174) -> (transposed array=w1180:dbl[][])
                    n617 = Array Size(array=w1174) -> (size(s)=w1175:i32[])
                    n618 = Multiply Array Elements(1:w1175) -> (0:w1181:i32)
                    n619 = Reshape Array(w1180, w1181) -> (w1179:dbl[])
                    n620 = call <vilib>:"Write File+ [SGL].vi"("1D array"=w1179, "error in (no error)"=w1182, "refnum"=w1183) -> ()  [unwired: 6 in, 3 out]
                  }
                }
                n621 = case shown="True" w1127 {
                  tunnel: w1126 -> [_ w1135]
                  frame False {
                  }
                  frame True {
                    n622 = event shown="[0] \"Move time\": Value Change" {
                      selector: _ -> [_ _]
                      dyn-events: _ -> [_ _]
                      timeout: 1 -> [_ _]
                      tunnel: w1135 -> [w1140 _]
                      event "Move time": Value Change {
                        n623 = event-data() -> ("NewVal"=w1139:string)  [unwired: 1 in, 5 out]
                        n624 = Concatenate Strings(w1139, "\r\n") -> (w1137:string)
                        n625 = Write to Text File(file (use dialog)=w1140, text=w1137) -> ()  [unwired: 2 in, 3 out]
                      }
                      event Timeout {
                        n626 = event-data() -> ()  [unwired: 1 in, 3 out]
                      }
                    }
                  }
                }
              }
            }
            "Progress" <- w1095
          }
        }
      }
    }
    n627 = Square Root(x=w475) -> (sqrt(x)=→"Force noise (pN)":dbl)
    n628 = local read "Flushing Sample"() -> (w407:bool)
    n629 = case shown="True" w407 {
      frame False {
      }
      frame True {
        n630 = local read "Flush Sample Start Time"() -> (w818:u32)
        n631 = local read "Sample flush time (s)"() -> (w811:dbl)
        n632 = Tick Count (ms)() -> (millisecond timer value=w819:u32)
        n633 = Subtract(x=w819, y=w818) -> (x-y=w809:u32)
        n634 = Multiply(x=u32 1000, y=w811) -> (x*y=w810:dbl)
        n635 = Divide(x=w809, y=w810) -> (x/y=w814:dbl)
        n636 = Greater?(x=w809, y=w810) -> (0:w817:bool)
        n637 = Not(x=w817) -> (.not. x?=w816:bool)
        n638 = Boolean To (0,1)(Boolean=w816) -> (0, 1=w815:i16)
        n639 = Compound Arithmetic op=MULTIPLY(w815, w814, 100.0 ("value")) -> (→"Sample Flush Meter":dbl)
        n640 = case shown="True" w817 {
          frame False {
          }
          frame True {
            w821 = FALSE ("Inject Sample")
            n641 = property on="Clear Volume" class="Bool (strict)"("Val(Sgnl)"=TRUE ("Value (Signaling)")) -> ()  [unwired: 2 in, 2 out]
            n642 = local write "Inject Sample"(w821) -> ()
            n643 = local write "Flushing Sample"(w821) -> ()
          }
        }
      }
    }
    n644 = feedback #12(0) -> (w391:i32)
    n645 = feedback #13(0) -> (w388:i32)
    n646 = feedback #14(0) -> (w393:i32)
    n647 = case shown="True" w398 {
      tunnel: w402 -> [w710 w768]
      tunnel: [w710 w752] -> w401
      tunnel: w400 -> [w709 w767]
      tunnel: [w709 w751] -> w399
      tunnel: "Raster scan" -> [w708 w745]
      tunnel: [w708 w744] -> w396
      tunnel: [0 w743] -> w394
      tunnel: w393 -> [_ w737]
      tunnel: w391 -> [_ w725]
      tunnel: [0 w728] -> w390
      tunnel: w388 -> [_ w734]
      tunnel: [0 w733] -> w387
      frame False {
      }
      frame True {
        # "Reset step counter"
        # "Current position"
        # "Initial values"
        n648 = local read "Conv Y (nm/V)"() -> (w720:dbl)
        n649 = local read "Conv X (nm/V)"() -> (w721:dbl)
        n650 = local read "Trap delta (nm)"() -> (w719:dbl)
        n651 = disable-structure shown="Disabled" {
          frame Disabled {
            n652 = local write "Raster scan"(FALSE ("Raster scan")) -> ()
            n653 = property on="Reset data stream" class="Bool (strict)"("Val(Sgnl)"=TRUE) -> ()  [unwired: 2 in, 2 out]
          }
          frame Enabled {
          }
        }
        n654 = local read "Data update period (s/set)"() -> (w742:dbl)
        n655 = local read "Time per step (ms)"() -> (w739:dbl)
        n656 = Select(t=w720, s="Pulling direction", f=w721) -> (s? t:f=w718:dbl)
        n657 = Divide(x=w719, y=w718) -> (x/y=w717:dbl)
        n658 = local read "Fixed X"() -> (w761:dbl)
        n659 = local read "Fixed Y"() -> (w762:dbl)
        n660 = local read "Fixed X"() -> (w723:dbl)
        n661 = local read "Fixed Y"() -> (w722:dbl)
        n662 = local read "Trap position (V)"() -> (w724:cluster{"X":dbl, "Y":dbl})
        n663 = Select(t=w722, s="Pulling direction", f=w723) -> (s? t:f=w716:dbl)
        n664 = local read "Scan steps (mirror)"() -> (w750:u64)
        n665 = Unbundle(w724) -> ("X"=w714:dbl, "Y"=w715:dbl)
        n666 = Multiply(x=w742, y=1000.0) -> (x*y=w740:dbl)
        n667 = local read "Stop raster"() -> (w757:bool)
        n668 = local read "Stop saving"() -> (w758:bool)
        n669 = Select(t=w761, s="Pulling direction", f=w762) -> (s? t:f=w769:dbl)
        n670 = Add(x=w717, y=w716) -> ()  [unwired: 1 out]
        n671 = local write "Saving Move"(FALSE) -> ()
        n672 = Divide(x=w739, y=w740) -> (x/y=w738:dbl)
        n673 = Quotient & Remainder(x=w737, y=w738) -> (x-y*floor(x/y)=w736:dbl)  [unwired: 1 out]
        n674 = Not(x=w757) -> (.not. x?=w756:bool)
        n675 = Select(t=w715, s="Pulling direction", f=w714) -> (s? t:f=w712:dbl)
        n676 = Not(x=w758) -> (.not. x?=w755:bool)
        n677 = Multiply(x=u64 2, y=w750) -> (x*y=w746:u64)
        n678 = Equal To 0?(x=w736) -> (x = 0?=w735:bool)
        n679 = Less?(x=w725, y=w746) -> (x < y?=w747:bool)
        n680 = Compound Arithmetic op=AND(w747, w756, w755, w735) -> (w748:bool)
        n681 = Not(x=w747) -> (.not. x?=w731:bool)
        n682 = feedback #15() -> (w753:dbl)  [unwired: 1 in]
        n683 = case shown="True" w748 {
          tunnel: w769 -> [_ w804]
          tunnel: w712 -> [_ w786]
          tunnel: w768 -> [w781 w803]
          tunnel: w767 -> [w780 w802]
          tunnel: [w781 w801] -> w752
          tunnel: [w780 w800] -> w751
          tunnel: [w777 w789] -> w754
          tunnel: w725 -> [w778 w784]
          tunnel: w753 -> [w777 w783]
          tunnel: w745 -> [w779 w788]
          tunnel: [w779 w788] -> w744
          tunnel: [w778 w787] -> w729
          frame False {
          }
          frame True {
            # "Go forward or backward?"
            n684 = local read "Scan increment (V)"() -> (w782:dbl)
            n685 = local read "Scan steps (mirror)"() -> (w793:u64)
            n686 = Multiply(x=w782, y=w784) -> (x*y=w785:dbl)
            n687 = Less?(x=w784, y=w793) -> (x < y?=w792:bool)
            n688 = Add(x=w786, y=w785) -> (x+y=w795:dbl)
            n689 = Subtract(x=w783, y=w782) -> (x-y=w794:dbl)
            n690 = Select(t=w795, s=w792, f=w794) -> (s? t:f=w789:dbl)
            n691 = local read "Pulling direction"() -> (w791:bool)
            n692 = Build Array(w789, w804) -> (w798:dbl[])
            n693 = Build Array(w804, w789) -> (w797:dbl[])
            n694 = Select(t=w798, s=w791, f=w797) -> (s? t:f=w796:dbl[])
            n695 = call-poly <vilib>:"DAQmx Write.vi"("task/channels in"=w803, "auto start"=TRUE, "data"=w796, "error in"=w802) -> ("task out"=w801:refnum<k21>, "error out"=w800:errorcluster)  [unwired: 9 in, 1 out]
            n696 = Increment(x=w784) -> (x+1=w787:i32)
            "Raster scanning..." <- TRUE ("Raster scanning...")
          }
        }
        n697 = feedback-in #15(w754) -> ()
        n698 = case shown="True" w731 {
          tunnel: w734 -> [w774 w776]
          tunnel: [w774 w775] -> w733
          frame False {
          }
          frame True {
            n699 = Increment(x=w776) -> (x+1=w775:i32)
          }
        }
        n700 = local read "# scans"() -> (w732:i32)
        n701 = local read "Stop saving"() -> (w760:bool)
        n702 = Greater Or Equal?(x=w733, y=w732) -> (x >= y?=w726:bool)
        n703 = Not(x=w726) -> (.not. x?=w727:bool)
        n704 = And(x=w731, y=w727) -> (x .and. y?=w730:bool)
        n705 = Compound Arithmetic op=OR(w726, "Stop raster", w760) -> (w763:bool)
        n706 = case shown="True" w763 {
          frame False {
          }
          frame True {
            n707 = flat-sequence {
              frame #0 {
                n708 = Wait (ms)(milliseconds to wait=u32 300) -> ()  [unwired: 1 out]
              }
              frame #1 {
                n709 = property on="Trap delta (nm)" class="DigNum (strict)"("Val(Sgnl)"="Trap delta\nafter (nm)") -> ()  [unwired: 2 in, 2 out]
              }
            }
          }
        }
        n710 = And(x="Flow on\nafter raster?", y=w763) -> (x .and. y?=w764:bool)
        n711 = case shown="True" w764 {
          frame False {
          }
          frame True {
            n712 = property on="Inject Sample" class="Bool (strict)"("Val(Sgnl)"=TRUE ("Value (Signaling)")) -> ()  [unwired: 2 in, 2 out]
          }
        }
        n713 = case shown="True" w730 {
          tunnel: w729 -> [w772 _]
          tunnel: [w772 0] -> w728
          frame False {
          }
          frame True {
          }
        }
        n714 = Not(x=w763) -> (.not. x?=w766:bool)
        n715 = local write "Raster scanning..."(w766) -> ()
        n716 = Increment(x=w737) -> (x+1=w743:i32)
      }
    }
    n717 = And(x="Save scans", y=w396) -> (x .and. y?=w405:bool)
    n718 = feedback-in #12(w390) -> ()
    n719 = feedback-in #13(w387) -> ()
    n720 = feedback-in #14(w394) -> ()
    n721 = local read "Stop"() -> (w683:bool)
  }
  n722 = local write "Progress"(u8 0 ("Progress")) -> ()
  n723 = local write "Calibrating"(FALSE ("Calibrating")) -> ()
  n724 = VISA Open(VISA resource name="USB port") -> (VISA resource name=w12:refnum<visa-resource-name>, error out=w11:errorcluster)  [unwired: 1 in, 3 out]
  n725 = VISA Enable Event(8:w11, 10:w10, 11:w12) -> (0:w7:errorcluster, 3:w8:refnum<visa-resource-name>)  [unwired: 1 out]
  n726 = call-poly "VISA Configure Serial Port"("VISA resource name"=refnum<visa-resource-name> "COM5", "baud rate (9600)"=u32 19200) -> ("VISA resource name out"=w2:refnum<visa-resource-name>, "error out"=w28:errorcluster)  [unwired: 12 in]
  n727 = while {
    tunnel: w2 -> [w1267]
    shift-right: [w1263] -> w4
    shift-left: w8 -> [w1266]
    shift-right: [w1264] -> w3
    shift-left: w7 -> [w1265]
    stop <- w1262 stop-if-true
    n728 = global read "FAST_Global_var.vi" "FAST L"() -> (→"FAST Z" →"FAST Z":bool)
    n729 = global read "FAST_Global_var.vi" "FAST R"() -> (→"FAST X-Y" →"FAST X-Y":bool)
    n730 = call "LogitechSubVi.vi"("USB port"=w1266, "VISA resource name in 2 (for the Newport)"=w1267, "error in (no error)"=w1265, "X-Y Wait time"="X-Y Wait time", "Z Wait time"="Z Wait time", "XY Speed Definitions"="XY Speed Definitions", "Z Speed Definitions"="Z Speed Definitions") -> ("Right stick button"=→"Right stick button":bool, "Left stick button"=→"Left stick button":bool, "USB port out"=w1263:refnum<visa-resource-name>, "error out"=w1264:errorcluster, "A B X Y"=w1256:cluster{"A":bool, "B":bool, "X":bool, "Y":bool}, "LB RB"=w1255:T21, "U D L R"=w1261:cluster{"U":bool, "D":bool, "L":bool, "R":bool}, "Sticks"=w1254:T22)  [unwired: 5 in]
    n731 = Unbundle By Name(w1255) -> ("LB"=w1249:bool, "RB"=w1248:bool, "BACK"=w1222:bool, "Logitech"=w1221:bool, "START"=w1223:bool)
    "RB" <- w1248
    "LB" <- w1249
    "BACK" <- w1222
    "START" <- w1223
    "Logitech" <- w1221
    n732 = case shown="True" w1223 {
      selector: w1223 -> [_ w1271]
      frame False {
      }
      frame True {
        n733 = property on="Move to Position 2" class="Bool (strict)"("Val(Sgnl)"=w1271) -> ()  [unwired: 2 in, 2 out]
      }
    }
    n734 = case shown="True" w1221 {
      frame False {
      }
      frame True {
        n735 = local read "Inject Sample"() -> (w1268:bool)
        n736 = Not(x=w1268) -> (.not. x?=w1269:bool)
        n737 = property on="Inject Sample" class="Bool (strict)"("Val(Sgnl)"=w1269) -> ()  [unwired: 2 in, 2 out]
      }
    }
    n738 = case shown="True" w1249 {
      frame False {
      }
      frame True {
        n739 = local read "Shutter 1 (B)"() -> (w1315:bool)
        n740 = Not(x=w1315) -> (.not. x?=w1314:bool)
        n741 = property on="Shutter 1 (B)" class="Bool (strict)"("Val(Sgnl)"=w1314) -> ()  [unwired: 2 in, 2 out]
      }
    }
    n742 = case shown="True" w1222 {
      selector: w1222 -> [_ w1270]
      frame False {
      }
      frame True {
        n743 = property on="Move to Position 1" class="Bool (strict)"("Val(Sgnl)"=w1270) -> ()  [unwired: 2 in, 2 out]
      }
    }
    n744 = Unbundle By Name(w1261) -> ("U"=→"U":bool, "D"=→"D":bool, "L"=→"L":bool, "R"=→"R":bool)
    n745 = Unbundle By Name(w1256) -> ("A"=w1244:bool, "B"=w1242:bool, "X"=w1247:bool, "Y"=w1240:bool)
    "A" <- w1244
    "B" <- w1242
    "X" <- w1247
    "Y" <- w1240
    n746 = case shown="\"Fish\"" "A command" {
      tunnel: w1244 -> [w1294 w1296 w1298 w1301]
      frame "Got ADig", Default {
        n747 = case shown="True" w1294 {
          selector: w1294 -> [_ w1295]
          frame False {
          }
          frame True {
            n748 = property on="Got ADig bead" class="Bool (strict)"("Val(Sgnl)"=w1295) -> ()  [unwired: 2 in, 2 out]
          }
        }
      }
      frame "Dump" {
        n749 = case shown="True" w1296 {
          selector: w1296 -> [_ w1297]
          frame False {
          }
          frame True {
            n750 = property on="Dump beads" class="Bool (strict)"("Val(Sgnl)"=w1297) -> ()  [unwired: 2 in, 2 out]
          }
        }
      }
      frame "Fish" {
        n751 = case shown="True" w1298 {
          frame False {
          }
          frame True {
            n752 = local read "Fish"() -> (w1299:bool)
            n753 = Not(x=w1299) -> (.not. x?=w1300:bool)
            n754 = property on="Fish" class="Bool (strict)"("Val(Sgnl)"=w1300) -> ()  [unwired: 2 in, 2 out]
          }
        }
      }
      frame "Got DNA" {
        n755 = case shown="True" w1301 {
          selector: w1301 -> [_ w1302]
          frame False {
          }
          frame True {
            n756 = property on="Got DNA bead" class="Bool (strict)"("Val(Sgnl)"=w1302) -> ()  [unwired: 2 in, 2 out]
          }
        }
      }
    }
    n757 = case shown="True" w1248 {
      frame False {
      }
      frame True {
        n758 = local read "Shutter 2 (A)"() -> (w1313:bool)
        n759 = Not(x=w1313) -> (.not. x?=w1312:bool)
        n760 = property on="Shutter 2 (A)" class="Bool (strict)"("Val(Sgnl)"=w1312) -> ()  [unwired: 2 in, 2 out]
      }
    }
    n761 = Unbundle By Name(w1254) -> ("Right X"=w1226:i8, "Right Y"=w1228:i8, "Left X"=w1230:i8, "Left Y"=w1235:i8)
    n762 = Not Equal?(x=w1235, y=i8 0) -> (x != y?=w1236:bool)
    n763 = case shown="True" w1236 {
      tunnel: w1235 -> [_ w1275]
      frame False {
      }
      frame True {
        "Left Y" <- w1275
      }
    }
    n764 = case shown="\"Got DNA\", Default" "B command" {
      tunnel: w1242 -> [w1285 w1287 w1289 w1291]
      frame "Got DNA", Default {
        n765 = case shown="True" w1285 {
          selector: w1285 -> [_ w1286]
          frame False {
          }
          frame True {
            n766 = property on="Got DNA bead" class="Bool (strict)"("Val(Sgnl)"=w1286) -> ()  [unwired: 2 in, 2 out]
          }
        }
      }
      frame "Got ADig" {
        n767 = case shown="True" w1287 {
          selector: w1287 -> [_ w1288]
          frame False {
          }
          frame True {
            n768 = property on="Got ADig bead" class="Bool (strict)"("Val(Sgnl)"=w1288) -> ()  [unwired: 2 in, 2 out]
          }
        }
      }
      frame "Dump" {
        n769 = case shown="True" w1289 {
          selector: w1289 -> [_ w1290]
          frame False {
          }
          frame True {
            n770 = property on="Dump beads" class="Bool (strict)"("Val(Sgnl)"=w1290) -> ()  [unwired: 2 in, 2 out]
          }
        }
      }
      frame "Fish" {
        n771 = case shown="True" w1291 {
          frame False {
          }
          frame True {
            n772 = local read "Fish"() -> (w1292:bool)
            n773 = Not(x=w1292) -> (.not. x?=w1293:bool)
            n774 = property on="Fish" class="Bool (strict)"("Val(Sgnl)"=w1293) -> ()  [unwired: 2 in, 2 out]
          }
        }
      }
    }
    n775 = Not Equal?(x=w1226, y=i8 0) -> (x != y?=w1227:bool)
    n776 = Not Equal?(x=w1228, y=i8 0) -> (x != y?=w1229:bool)
    n777 = Not Equal?(x=w1230, y=i8 0) -> (x != y?=w1231:bool)
    n778 = case shown="True" w1231 {
      tunnel: w1230 -> [_ w1274]
      frame False {
      }
      frame True {
        "Left X" <- w1274
      }
    }
    n779 = case shown="False" w1227 {
      tunnel: w1226 -> [_ w1272]
      frame False {
      }
      frame True {
        "Right X" <- w1272
      }
    }
    n780 = case shown="False" w1229 {
      tunnel: w1228 -> [_ w1273]
      frame False {
      }
      frame True {
        "Right Y" <- w1273
      }
    }
    n781 = case shown="\"Dump\", Default" "X command" {
      tunnel: w1247 -> [w1303 w1305 w1308 w1310]
      frame "Dump", Default {
        n782 = case shown="True" w1303 {
          selector: w1303 -> [_ w1304]
          frame False {
          }
          frame True {
            n783 = property on="Dump beads" class="Bool (strict)"("Val(Sgnl)"=w1304) -> ()  [unwired: 2 in, 2 out]
          }
        }
      }
      frame "Fish" {
        n784 = case shown="True" w1305 {
          frame False {
          }
          frame True {
            n785 = local read "Fish"() -> (w1307:bool)
            n786 = Not(x=w1307) -> (.not. x?=w1306:bool)
            n787 = property on="Fish" class="Bool (strict)"("Val(Sgnl)"=w1306) -> ()  [unwired: 2 in, 2 out]
          }
        }
      }
      frame "Got ADig" {
        n788 = case shown="True" w1308 {
          selector: w1308 -> [_ w1309]
          frame False {
          }
          frame True {
            n789 = property on="Got ADig bead" class="Bool (strict)"("Val(Sgnl)"=w1309) -> ()  [unwired: 2 in, 2 out]
          }
        }
      }
      frame "Got DNA" {
        n790 = case shown="True" w1310 {
          selector: w1310 -> [_ w1311]
          frame False {
          }
          frame True {
            n791 = property on="Got DNA bead" class="Bool (strict)"("Val(Sgnl)"=w1311) -> ()  [unwired: 2 in, 2 out]
          }
        }
      }
    }
    n792 = case shown="\"Fish\", Default" "Y command" {
      tunnel: w1240 -> [w1276 w1279 w1281 w1283]
      frame "Fish", Default {
        n793 = case shown="True" w1276 {
          frame False {
          }
          frame True {
            n794 = local read "Fish"() -> (w1277:bool)
            n795 = Not(x=w1277) -> (.not. x?=w1278:bool)
            n796 = property on="Fish" class="Bool (strict)"("Val(Sgnl)"=w1278) -> ()  [unwired: 2 in, 2 out]
          }
        }
      }
      frame "Dump" {
        n797 = case shown="True" w1279 {
          selector: w1279 -> [_ w1280]
          frame False {
          }
          frame True {
            n798 = property on="Dump beads" class="Bool (strict)"("Val(Sgnl)"=w1280) -> ()  [unwired: 2 in, 2 out]
          }
        }
      }
      frame "Got ADig" {
        n799 = case shown="True" w1281 {
          selector: w1281 -> [_ w1282]
          frame False {
          }
          frame True {
            n800 = property on="Got ADig bead" class="Bool (strict)"("Val(Sgnl)"=w1282) -> ()  [unwired: 2 in, 2 out]
          }
        }
      }
      frame "Got DNA" {
        n801 = case shown="True" w1283 {
          selector: w1283 -> [_ w1284]
          frame False {
          }
          frame True {
            n802 = property on="Got DNA bead" class="Bool (strict)"("Val(Sgnl)"=w1284) -> ()  [unwired: 2 in, 2 out]
          }
        }
      }
    }
    n803 = local read "Stop"() -> (w1262:bool)
  }
  n804 = VISA Close(VISA resource name=w4, error in (no error)=w3) -> (error out=w5:errorcluster)
  n805 = call <vilib>:"Simple Error Handler.vi"("error in (no error)"=w5) -> ()  [unwired: 1 in, 8 out]
  n806 = node-c288(i64 100 ("Period"), 2 ("Processor")) -> (w30:T13)  [unwired: 2 in]
  n807 = timed-loop {
    timing: w30 -> [_]
    timing-out: [_] -> w29
    tunnel: w2 -> [w1316]
    tunnel: w28 -> [w1318]
    tunnel: [w1316] -> w27
    stop <- w1317 stop-if-true
    n808 = node-c288() -> ()  [unwired: 1 in, 1 out]
    n809 = event shown="[8] \"Grid Movable Trap\": Value Change" {
      selector: _ -> [_ _ _ _ _ _ _ _ _ _ _ _ _ _ _ _]
      dyn-events: _ -> [_ _ _ _ _ _ _ _ _ _ _ _ _ _ _ _]
      timeout: _ -> [_ _ _ _ _ _ _ _ _ _ _ _ _ _ _ _]
      tunnel: w1316 -> [w1325 w1377 w1397 w1415 w1432 w1453 w1501 w1516 _ w1672 _ _ _ _ _ _]
      tunnel: w1318 -> [w1324 w1376 w1396 w1414 w1431 w1452 w1500 w1515 _ w1670 _ _ _ _ _ _]
      tunnel: [_ _ _ _ _ _ _ _ _ _ _ _ _ _ _ w1860] -> w1317
      event "Got DNA bead": Value Change {
        n810 = event-data() -> ()  [unwired: 1 in, 5 out]
        n811 = flat-sequence {
          tunnel: w1324 -> [w1328]
          tunnel: ["Cal @ Delta (nm)"] -> w1320
          tunnel: w1325 -> [w1330]
          tunnel: [w1344] -> w1323
          tunnel: w1320 -> [w1343]
          tunnel: w1323 -> [w1365]
          tunnel: [w1365] -> w1322
          tunnel: w1322 -> [w1367]
          tunnel: [w1367] -> w1321
          tunnel: w1321 -> [w1369]
          frame #0 {
            n812 = local read "Saved stage positions"() -> (w1331:dbl[][])
            n813 = property on="Inject Sample" class="Bool (strict)"("Val(Sgnl)"=TRUE ("Value (Signaling)")) -> ()  [unwired: 2 in, 2 out]
            n814 = disable-structure shown="Disabled" {
              frame Disabled {
                n815 = property on="Inject Pump 2" class="Bool (strict)"("Val(Sgnl)"=FALSE ("Inject Pump 2")) -> ()  [unwired: 2 in, 2 out]
              }
              frame Enabled {
              }
            }
            n816 = local write "Stage moving"(TRUE ("Stage moving")) -> ()
            n817 = property on="Trap delta (nm)" class="DigNum (strict)"("Val(Sgnl)"="Cal @ Delta (nm)") -> ()  [unwired: 2 in, 2 out]
            n818 = call "move to saved stage position.vi"("error in"=w1328, "Stage VISA resource name in"=w1330, "Position"="Cal stage position", "Saved Stage Positions"=w1331) -> ()  [unwired: 2 out]
          }
          frame #1 {
            n819 = local write "Stage moving"(FALSE ("Stage moving")) -> ()
            n820 = property on="Inject Sample" class="Bool (strict)"("Val(Sgnl)"=FALSE ("Value (Signaling)")) -> ()  [unwired: 2 in, 2 out]
            n821 = call <vilib>:"Beep.vi"() -> ()  [unwired: 12 in]
          }
          frame #2 {
            # "increased from 1000 to 5000 v6.4. \nMar.7,2018."
            n822 = Wait (ms)(milliseconds to wait=u32 5000) -> ()  [unwired: 1 out]
          }
          frame #3 {
            n823 = property on="Save cal" class="Bool (strict)"("Val(Sgnl)"=TRUE ("Value (Signaling)")) -> ()  [unwired: 2 in, 2 out]
          }
          frame #4 {
            n824 = Wait (ms)(milliseconds to wait=u32 2000) -> ()  [unwired: 1 out]
          }
          frame #5 {
            n825 = while {
              stop <- w1340 stop-if-true
              n826 = local read "Saving"() -> (w1341:bool)
              n827 = Not(x=w1341) -> (.not. x?=w1340:bool)
              n828 = Wait (ms)(milliseconds to wait=u32 100) -> ()  [unwired: 1 out]
            }
          }
          frame #6 {
            n829 = Wait (ms)(milliseconds to wait=u32 2000) -> ()  [unwired: 1 out]
          }
          frame #7 {
            n830 = stacked-sequence {
              tunnel: [_ _ _ _ _ _ w1359 _] -> w1344
              tunnel: w1343 -> [_ _ _ _ _ _ _ w1364]
              frame #0 {
                n831 = property on="Trap delta (nm)" class="DigNum (strict)"("Val(Sgnl)"="Offset @ Delta (nm)") -> ()  [unwired: 2 in, 2 out]
                n832 = Replace Array Subset(array=i32[] [0], new element="Offset raster set", index=0) -> (w1348:i32[])
                n833 = property on="Scan Parameters" class="Arr (strict)"("Index Values"=w1348) -> ()  [unwired: 2 in, 2 out]
              }
              frame #1 {
                n834 = Wait (ms)(milliseconds to wait=u32 200) -> ()  [unwired: 1 out]
              }
              frame #2 {
                n835 = property on="Load param" class="Bool (strict)"("Val(Sgnl)"=TRUE ("Load param")) -> ()  [unwired: 2 in, 2 out]
              }
              frame #3 {
                n836 = Wait (ms)(milliseconds to wait=u32 200) -> ()  [unwired: 1 out]
              }
              frame #4 {
                # "Only continue if there is no buffer\noverflow error"
                n837 = local read "Buffer Overflow"() -> (w1354:bool)
                n838 = Not(x=w1354) -> (.not. x?=w1353:bool)
                n839 = case shown="True" w1353 {
                  frame False {
                  }
                  frame True {
                    n840 = property on="Raster scan" class="Bool (strict)"("Val(Sgnl)"=TRUE ("Value (Signaling)")) -> ()  [unwired: 2 in, 2 out]
                  }
                }
              }
              frame #5 {
                n841 = local read "Buffer Overflow"() -> (w1357:bool)
                n842 = Not(x=w1357) -> (.not. x?=w1356:bool)
                n843 = case shown="True" w1356 {
                  frame False {
                  }
                  frame True {
                    n844 = Wait (ms)(milliseconds to wait=u32 2000) -> ()  [unwired: 1 out]
                  }
                }
              }
              frame #6 {
                n845 = local read "Buffer Overflow"() -> (w1360:bool)
                n846 = Not(x=w1360) -> (.not. x?=w1359:bool)
                n847 = case shown="True" w1359 {
                  frame False {
                  }
                  frame True {
                    n848 = while {
                      stop <- w1362 stop-if-true
                      n849 = local read "Saving"() -> (w1363:bool)
                      n850 = Not(x=w1363) -> (.not. x?=w1362:bool)
                      n851 = Wait (ms)(milliseconds to wait=u32 100) -> ()  [unwired: 1 out]
                    }
                  }
                }
              }
              frame #7 {
                n852 = property on="Trap delta (nm)" class="DigNum (strict)"("Val(Sgnl)"=w1364) -> ()  [unwired: 2 in, 2 out]
              }
            }
          }
          frame #8 {
            n853 = case shown="True" w1365 {
              frame False {
              }
              frame True {
                n854 = property on="Read Cal" class="Bool (strict)"("Val(Sgnl)"=TRUE ("Value (Signaling)")) -> ()  [unwired: 2 in, 2 out]
              }
            }
          }
          frame #9 {
            n855 = case shown="True" w1367 {
              frame False {
              }
              frame True {
                n856 = Wait (ms)(milliseconds to wait=u32 1000) -> ()  [unwired: 1 out]
              }
            }
          }
          frame #10 {
            n857 = case shown="True" w1369 {
              frame False {
              }
              frame True {
                n858 = property on="Fish" class="Bool (strict)"("Val(Sgnl)"=TRUE ("Value (Signaling)")) -> ()  [unwired: 2 in, 2 out]
                n859 = case shown="False" "Flow on\nwhile fish?" {
                  frame False {
                    n860 = property on="Inject Sample" class="Bool (strict)"("Val(Sgnl)"=FALSE) -> ()  [unwired: 2 in, 2 out]
                  }
                  frame True {
                    n861 = property on="Inject Sample" class="Bool (strict)"("Val(Sgnl)"=TRUE ("Value (Signaling)")) -> ()  [unwired: 2 in, 2 out]
                  }
                }
              }
            }
          }
        }
        n862 = local write "Got DNA bead"(FALSE) -> ()
      }
      event "Dump beads": Value Change {
        n863 = event-data() -> ()  [unwired: 1 in, 5 out]
        n864 = flat-sequence {
          tunnel: w1376 -> [w1380]
          tunnel: w1377 -> [w1381]
          tunnel: [w1381] -> w1375
          tunnel: [w1380] -> w1374
          tunnel: w1375 -> [w1384]
          tunnel: w1374 -> [w1383]
          frame #0 {
            w1378 = FALSE ("Fish")
            n865 = local read "Saving"() -> (w1379:bool)
            n866 = local write "Force Feedback 2"(w1378) -> ()
            n867 = local write "Pause dwell"(w1378) -> ()
            n868 = local write "Force Feedback 1"(w1378) -> ()
            n869 = local write "Dump beads"(w1378) -> ()
            n870 = property on="Stop saving" class="Bool (strict)"("Val(Sgnl)"=w1379) -> ()  [unwired: 2 in, 2 out]
            n871 = local write "Fish"(w1378) -> ()
          }
          frame #1 {
            n872 = local read "Saved stage positions"() -> (w1386:dbl[][])
            n873 = case shown="True" "Flow on\ndump?" {
              frame False {
              }
              frame True {
                n874 = property on="Inject Sample" class="Bool (strict)"("Val(Sgnl)"=TRUE ("Value (Signaling)")) -> ()  [unwired: 2 in, 2 out]
              }
            }
            n875 = local write "Stage moving"(TRUE ("Stage moving")) -> ()
            n876 = call "move to saved stage position.vi"("error in"=w1383, "Stage VISA resource name in"=w1384, "Position"=5, "Saved Stage Positions"=w1386) -> ()  [unwired: 2 out]
          }
          frame #2 {
            n877 = local read "Shutter 1 (B)"() -> (w1391:bool)
            n878 = local read "Shutter 2 (A)"() -> (w1390:bool)
            n879 = call <vilib>:"Beep.vi"() -> ()  [unwired: 12 in]
            n880 = case shown="True" w1391 {
              frame False {
              }
              frame True {
                n881 = property on="Shutter 1 (B)" class="Bool (strict)"("Val(Sgnl)"=FALSE ("Value (Signaling)")) -> ()  [unwired: 2 in, 2 out]
              }
            }
            n882 = case shown="True" w1390 {
              frame False {
              }
              frame True {
                n883 = property on="Shutter 2 (A)" class="Bool (strict)"("Val(Sgnl)"=FALSE) -> ()  [unwired: 2 in, 2 out]
              }
            }
            n884 = local write "Stage moving"(FALSE ("Stage moving")) -> ()
            n885 = local write "Tether"(FALSE ("Tether")) -> ()
          }
          frame #3 {
            n886 = property on="Move Cap. 2 (ADig Top)" class="Bool (strict)"("Val(Sgnl)"=TRUE ("Value (Signaling)")) -> ()  [unwired: 2 in, 2 out]
          }
        }
      }
      event "Move Cap. 2 (ADig Top)": Value Change {
        n887 = event-data() -> ()  [unwired: 1 in, 5 out]
        n888 = flat-sequence {
          tunnel: w1397 -> [w1401]
          tunnel: w1396 -> [w1400]
          frame #0 {
            n889 = local read "Saved stage positions"() -> (w1399:dbl[][])
            n890 = case shown="True" "Flow on\ncap 2?" {
              frame False {
              }
              frame True {
                n891 = property on="Inject Sample" class="Bool (strict)"("Val(Sgnl)"=TRUE ("Value (Signaling)")) -> ()  [unwired: 2 in, 2 out]
              }
            }
            n892 = local write "Move Cap. 2 (ADig Top)"(FALSE ("Move Cap. 2 (ADig Top)")) -> ()
            n893 = local write "Stage moving"(TRUE ("Stage moving")) -> ()
            n894 = call "move to saved stage position.vi"("error in"=w1400, "Stage VISA resource name in"=w1401, "Position"=2, "Saved Stage Positions"=w1399) -> ()  [unwired: 2 out]
          }
          frame #1 {
            # "Make sure you don't reverse\nwhich is ON and OFF"
            n895 = local read "Cal @ Delta (nm)"() -> (w1409:dbl)
            n896 = local write "Stage moving"(FALSE ("Stage moving")) -> ()
            n897 = call <vilib>:"Beep.vi"() -> ()  [unwired: 12 in]
            n898 = property on="Trap delta (nm)" class="DigNum (strict)"("Val(Sgnl)"=w1409) -> ()  [unwired: 2 in, 2 out]
            n899 = property class="TabCtl (strict)"("Val(Sgnl)"=T4."Status" ("Value (Signaling)")) -> ()  [unwired: 2 in, 2 out]
            n900 = disable-structure shown="Disabled" {
              frame Disabled {
                n901 = property on="Inject Pump 1" class="Bool (strict)"("Val(Sgnl)"=TRUE ("Inject Pump 2")) -> ()  [unwired: 2 in, 2 out]
              }
              frame Enabled {
              }
            }
            n902 = local read "Shutter 2 (A)"() -> (w1408:bool)
            n903 = case shown="False" w1408 {
              frame False {
                n904 = property on="Shutter 2 (A)" class="Bool (strict)"("Val(Sgnl)"=TRUE ("Value (Signaling)")) -> ()  [unwired: 2 in, 2 out]
              }
              frame True {
              }
            }
            n905 = property on="Inject Sample" class="Bool (strict)"("Val(Sgnl)"=FALSE ("Value (Signaling)")) -> ()  [unwired: 2 in, 2 out]
          }
        }
      }
      event "Got ADig bead": Value Change {
        n906 = event-data() -> ()  [unwired: 1 in, 5 out]
        n907 = flat-sequence {
          tunnel: w1415 -> [w1419]
          tunnel: w1414 -> [w1418]
          frame #0 {
            n908 = local read "Saved stage positions"() -> (w1421:dbl[][])
            n909 = property on="Inject Pump 1" class="Bool (strict)"("Val(Sgnl)"=FALSE ("Inject Pump 2")) -> ()  [unwired: 2 in, 2 out]
            n910 = case shown="True" "Flow on\ncap 1?" {
              frame False {
              }
              frame True {
                n911 = property on="Inject Sample" class="Bool (strict)"("Val(Sgnl)"=TRUE ("Value (Signaling)")) -> ()  [unwired: 2 in, 2 out]
              }
            }
            n912 = local write "Stage moving"(TRUE ("Stage moving")) -> ()
            n913 = call "move to saved stage position.vi"("error in"=w1418, "Stage VISA resource name in"=w1419, "Position"=1, "Saved Stage Positions"=w1421) -> ()  [unwired: 2 out]
          }
          frame #1 {
            n914 = local read "Shutter 1 (B)"() -> (w1425:bool)
            n915 = disable-structure shown="Disabled" {
              frame Disabled {
                n916 = property on="Inject Pump 2" class="Bool (strict)"("Val(Sgnl)"=TRUE ("Inject Pump 2")) -> ()  [unwired: 2 in, 2 out]
              }
              frame Enabled {
              }
            }
            n917 = local write "Stage moving"(FALSE ("Stage moving")) -> ()
            n918 = case shown="False" w1425 {
              frame False {
                n919 = property on="Shutter 1 (B)" class="Bool (strict)"("Val(Sgnl)"=TRUE ("Value (Signaling)")) -> ()  [unwired: 2 in, 2 out]
              }
              frame True {
              }
            }
            n920 = property on="Inject Sample" class="Bool (strict)"("Val(Sgnl)"=FALSE ("Value (Signaling)")) -> ()  [unwired: 2 in, 2 out]
            n921 = call <vilib>:"Beep.vi"() -> ()  [unwired: 12 in]
          }
        }
        n922 = local write "Got ADig bead"(FALSE ("Got ADig bead")) -> ()
      }
      event "Set Position 1", "Set Position 2", "Set Position 3", "Set Position 4", "Set Position 5": Value Change {
        n923 = event-data() -> ()  [unwired: 1 in, 5 out]
        n924 = Build Array("Set Position 1", "Set Position 2", "Set Position 3", "Set Position 4", "Set Position 5") -> (w1444:bool[])
        n925 = Boolean Array To Number(Boolean array=w1444) -> (number=w1443:u32)
        n926 = call "Read Stage Position.vi"("error in"=w1431, "VISA resource name in"=w1432) -> ("Current Position"=w1429:cluster{dbl, dbl, dbl}, "error out"=→"Stage error":errorcluster)  [unwired: 1 in, 1 out]
        n927 = Logarithm Base 2(1:w1443) -> (0:w1437:dbl)
        n928 = Cluster To Array(cluster=w1429) -> (array=w1439:dbl[])
        n929 = Increment(x=w1437) -> (x+1=w1440:dbl)
        n930 = Build Array (concatenate)(w1440, w1439) -> (w1438:dbl[])
        n931 = Replace Array Subset(array="Saved stage positions", new element=w1438, index (row)=w1437) -> (w1441:dbl[][])  [unwired: 1 in]
        n932 = local write "Saved stage positions"(w1441) -> ()
      }
      event "Move to Position 2", "Move to Position 4", "Move to Position 3", "Move to Position 5", "Move to Position 1": Value Change {
        w1447 = FALSE
        n933 = event-data() -> ()  [unwired: 1 in, 5 out]
        n934 = Build Array("Move to Position 1", "Move to Position 2", "Move to Position 3", "Move to Position 4", "Move to Position 5") -> (w1456:bool[])
        n935 = Boolean Array To Number(Boolean array=w1456) -> (number=w1455:u32)
        n936 = Logarithm Base 2(1:w1455) -> (0:w1454:dbl)
        n937 = flat-sequence {
          tunnel: w1454 -> [w1465]
          tunnel: w1453 -> [w1464]
          tunnel: w1452 -> [w1463]
          tunnel: [w1458] -> w1446
          tunnel: w1446 -> [w1475]
          frame #0 {
            # "only change move time when \nsaving move in T and calibrating is F"
            n938 = local read "Saved stage positions"() -> (w1466:dbl[][])
            n939 = property on="Saving Move" class="Bool (strict)"() -> ("Value"=w1460:bool)  [unwired: 2 in, 2 out]
            n940 = property on="Calibrating" class="Bool (strict)"() -> ("Value"=w1461:bool)  [unwired: 2 in, 2 out]
            n941 = Not(x=w1461) -> (.not. x?=w1459:bool)
            n942 = Increment(x=w1465) -> (x+1=w1458:dbl)
            n943 = And(x=w1460, y=w1459) -> (x .and. y?=w1462:bool)
            n944 = case shown="True" w1462 {
              frame False {
              }
              frame True {
                n945 = Get Date/Time In Seconds() -> (seconds since 1Jan1904=w1472:timestamp)
                n946 = Format Date/Time String(time format string (%c)="%H:%M:%S%3u", seconds (now)=w1472, UTC format=TRUE) -> (date/time string=w1471:string)
                n947 = call <vilib>:"Space Constant.vi"() -> ("String"=w1470:string)
                n948 = Concatenate Strings(w1471, w1470, "moving") -> (w1468:string)
                n949 = property on="Move time" class="Str"("Val(Sgnl)"=w1468) -> ()  [unwired: 2 in, 2 out]
              }
            }
            n950 = call "move to saved stage position.vi"("error in"=w1463, "Stage VISA resource name in"=w1464, "Position"=w1458, "Saved Stage Positions"=w1466) -> ()  [unwired: 2 out]
            n951 = call <vilib>:"Beep.vi"() -> ()  [unwired: 12 in]
            "Stage moving" <- TRUE ("Stage moving")
          }
          frame #1 {
            n952 = property on="Saving Move" class="Bool (strict)"() -> ("Value"=w1477:bool)  [unwired: 2 in, 2 out]
            n953 = property on="Calibrating" class="Bool (strict)"() -> ("Value"=w1478:bool)  [unwired: 2 in, 2 out]
            n954 = call <vilib>:"Beep.vi"() -> ()  [unwired: 12 in]
            n955 = Not(x=w1478) -> (.not. x?=w1476:bool)
            n956 = local write "Stage moving"(FALSE ("Stage moving")) -> ()
            n957 = And(x=w1477, y=w1476) -> (x .and. y?=w1479:bool)
            n958 = case shown="True" w1479 {
              tunnel: w1475 -> [_ w1483]
              frame False {
              }
              frame True {
                n959 = Get Date/Time In Seconds() -> (seconds since 1Jan1904=w1487:timestamp)
                n960 = Format Date/Time String(time format string (%c)="%H:%M:%S%3u", seconds (now)=w1487, UTC format=TRUE) -> (date/time string=w1486:string)
                n961 = Number To Decimal String(number=w1483, width (-)=i16 1) -> (decimal integer string=w1481:string)
                n962 = call <vilib>:"Space Constant.vi"() -> ("String"=w1484:string)
                n963 = Concatenate Strings(w1486, w1484, w1481) -> (w1485:string)
                n964 = property on="Move time" class="Str"("Val(Sgnl)"=w1485) -> ()  [unwired: 2 in, 2 out]
              }
            }
          }
        }
        n965 = local write "Move to Position 1"(w1447) -> ()
        n966 = local write "Move to Position 2"(w1447) -> ()
        n967 = local write "Move to Position 3"(w1447) -> ()
        n968 = local write "Move to Position 4"(w1447) -> ()
        n969 = local write "Move to Position 5"(w1447) -> ()
      }
      event "Set Current\nPos to (0,0,0)": Value Change {
        w1491 = ";" ("string")
        # "DH is \"Define Home\" -KW"
        n970 = event-data() -> ()  [unwired: 1 in, 5 out]
        n971 = local write "Set Current\nPos to (0,0,0)"(FALSE ("Set Current\nPos to (0,0,0)")) -> ()
        n972 = call-poly "VISA Configure Serial Port"("VISA resource name"=w1501, "baud rate (9600)"=u32 19200, "error in (no error)"=w1500) -> ("VISA resource name out"=w1495:refnum<visa-resource-name>, "error out"=w1494:errorcluster)  [unwired: 11 in]
        n973 = Concatenate Strings("1DH" ("string"), w1491, "2DH" ("string"), w1491, "3DH" ("string"), "\r") -> (w1493:string)
        n974 = VISA Write(VISA resource name=w1495, write buffer=w1493, error in (no error)=w1494) -> (error out=w1492:errorcluster)  [unwired: 2 out]
        n975 = local write "Stage error"(w1492) -> ()
      }
      event "Dip": Value Change {
        n976 = event-data() -> ()  [unwired: 1 in, 5 out]
        n977 = property on="Calibrating" class="Bool (strict)"() -> ("Value"=w1508:bool)  [unwired: 2 in, 2 out]
        n978 = Not(x=w1508) -> (.not. x?=w1506:bool)
        n979 = property on="Saving Move" class="Bool (strict)"() -> ("Value"=w1507:bool)  [unwired: 2 in, 2 out]
        n980 = And(x=w1507, y=w1506) -> (x .and. y?=w1505:bool)
        n981 = flat-sequence {
          tunnel: w1516 -> [w1520]
          tunnel: w1515 -> [w1519]
          tunnel: [w1521] -> w1513
          tunnel: [w1520] -> w1511
          tunnel: [w1519] -> w1509
          tunnel: w1505 -> [w1518]
          tunnel: ["Dip position"] -> w1504
          tunnel: [w1537] -> w1514
          tunnel: w1513 -> [w1537]
          tunnel: [w1536] -> w1512
          tunnel: w1511 -> [w1536]
          tunnel: [w1535] -> w1510
          tunnel: w1509 -> [w1535]
          tunnel: w1505 -> [w1531]
          tunnel: w1504 -> [w1530]
          tunnel: w1514 -> [w1568]
          tunnel: w1512 -> [w1567]
          tunnel: w1510 -> [w1566]
          tunnel: w1505 -> [w1564]
          tunnel: ["Start/Return position"] -> w1503
          tunnel: w1505 -> [w1577]
          tunnel: w1503 -> [w1576]
          frame #0 {
            n982 = local read "Saved stage positions"() -> (w1521:dbl[][])
            n983 = case shown="True" w1518 {
              frame False {
              }
              frame True {
                n984 = Get Date/Time In Seconds() -> (seconds since 1Jan1904=w1529:timestamp)
                n985 = call <vilib>:"Space Constant.vi"() -> ("String"=w1525:string)
                n986 = Format Date/Time String(time format string (%c)="%H:%M:%S%3u", seconds (now)=w1529, UTC format=TRUE) -> (date/time string=w1526:string)
                n987 = Concatenate Strings(w1526, w1525, "moving") -> (w1524:string)
                n988 = property on="Move time" class="Str"("Val(Sgnl)"=w1524) -> ()  [unwired: 2 in, 2 out]
              }
            }
            n989 = local write "Stage moving"(TRUE) -> ()
            n990 = call "move to saved stage position.vi"("error in"=w1519, "Stage VISA resource name in"=w1520, "Position"="Dip position", "Saved Stage Positions"=w1521) -> ()  [unwired: 2 out]
          }
          frame #1 {
            n991 = node-c288() -> (w1534:T13)  [unwired: 4 in]
            n992 = case shown="True" w1531 {
              tunnel: w1530 -> [_ w1541]
              frame False {
              }
              frame True {
                n993 = Get Date/Time In Seconds() -> (seconds since 1Jan1904=w1546:timestamp)
                n994 = Number To Decimal String(number=w1541, width (-)=i16 1) -> (decimal integer string=w1540:string)
                n995 = Format Date/Time String(time format string (%c)="%H:%M:%S%3u", seconds (now)=w1546, UTC format=TRUE) -> (date/time string=w1539:string)
                n996 = call <vilib>:"Space Constant.vi"() -> ("String"=w1543:string)
                n997 = Concatenate Strings(w1539, w1543, w1540) -> (w1538:string)
                n998 = property on="Move time" class="Str"("Val(Sgnl)"=w1538) -> ()  [unwired: 2 in, 2 out]
              }
            }
            n999 = timed-loop {
              timing: w1534 -> [_]
              timing-out: [_] -> w1533
              i -> [w1557]
              stop <- w1550 stop-if-true
              n1000 = node-c288() -> ()  [unwired: 1 in, 1 out]
              n1001 = local read "Cancel Rep\n Dip"() -> (w1547:bool)
              n1002 = Greater Or Equal?(x=w1557, y="Dip duration") -> (x >= y?=w1553:bool)
              n1003 = local read "Dump beads"() -> (w1548:bool)
              n1004 = Or(x=w1553, y="Cancel dwell") -> (x .or. y?=w1552:bool)
              n1005 = Not(x="Pause dwell") -> (.not. x?=w1554:bool)
              n1006 = node-c288() -> ()  [unwired: 1 in, 1 out]
              n1007 = And(x=w1554, y=w1552) -> (x .and. y?=w1551:bool)
              n1008 = Compound Arithmetic op=OR(w1551, w1548, w1547) -> (w1550:bool)
              "Dip elasped time" <- w1557
            }
            n1009 = local write "Stage moving"(FALSE ("Stage moving")) -> ()
            n1010 = node-c288(w1533) -> ()  [unwired: 1 out]
          }
          frame #2 {
            w1562 = FALSE ("Cancel dwell")
            n1011 = case shown="True" w1564 {
              frame False {
              }
              frame True {
                n1012 = Get Date/Time In Seconds() -> (seconds since 1Jan1904=w1575:timestamp)
                n1013 = Format Date/Time String(time format string (%c)="%H:%M:%S%3u", seconds (now)=w1575, UTC format=TRUE) -> (date/time string=w1572:string)
                n1014 = call <vilib>:"Space Constant.vi"() -> ("String"=w1571:string)
                n1015 = Concatenate Strings(w1572, w1571, "moving") -> (w1569:string)
                n1016 = property on="Move time" class="Str"("Val(Sgnl)"=w1569) -> ()  [unwired: 2 in, 2 out]
              }
            }
            n1017 = local write "Cancel dwell"(w1562) -> ()
            n1018 = local write "Cancel Rep\n Dip"(w1562) -> ()
            n1019 = local write "Stage moving"(TRUE) -> ()
            n1020 = call "move to saved stage position.vi"("error in"=w1566, "Stage VISA resource name in"=w1567, "Position"="Start/Return position", "Saved Stage Positions"=w1568) -> ()  [unwired: 2 out]
          }
          frame #3 {
            n1021 = case shown="True" w1577 {
              tunnel: w1576 -> [_ w1579]
              frame False {
              }
              frame True {
                n1022 = Get Date/Time In Seconds() -> (seconds since 1Jan1904=w1587:timestamp)
                n1023 = Number To Decimal String(number=w1579, width (-)=i16 1) -> (decimal integer string=w1580:string)
                n1024 = call <vilib>:"Space Constant.vi"() -> ("String"=w1584:string)
                n1025 = Format Date/Time String(time format string (%c)="%H:%M:%S%3u", seconds (now)=w1587, UTC format=TRUE) -> (date/time string=w1581:string)
                n1026 = Concatenate Strings(w1581, w1584, w1580) -> (w1582:string)
                n1027 = property on="Move time" class="Str"("Val(Sgnl)"=w1582) -> ()  [unwired: 2 in, 2 out]
              }
            }
            n1028 = local write "Stage moving"(FALSE ("Stage moving")) -> ()
          }
          frame #4 {
            n1029 = local write "Dip"(FALSE ("Dip")) -> ()
          }
        }
      }
      event "Grid Movable Trap": Value Change {
        n1030 = event-data() -> ()  [unwired: 1 in, 6 out]
        n1031 = flat-sequence {
          frame #0 {
            n1032 = local write "Shutter 1 (B)"(FALSE ("Shutter 1 (B)")) -> ()
          }
          frame #1 {
            n1033 = while {
              i -> [w1599]
              stop <- w1591 stop-if-true
              n1034 = Multiply(x=0.5, y=w1599) -> (x*y=w1597:dbl)
              n1035 = Add(x=0.0, y=w1597) -> (x+y=w1595:dbl)
              n1036 = while {
                tunnel: w1595 -> [w1605]
                tunnel: 0.5 ("x") -> [w1600]
                i -> [w1609]
                stop <- w1608 stop-if-true
                n1037 = flat-sequence {
                  tunnel: w1609 -> [w1624]
                  tunnel: [w1614] -> w1606
                  tunnel: w1605 -> [w1616]
                  tunnel: [w1619] -> w1603
                  tunnel: [w1618] -> w1601
                  tunnel: w1600 -> [w1612]
                  tunnel: [w1628] -> w1604
                  tunnel: w1603 -> [w1628]
                  tunnel: [w1627] -> w1602
                  tunnel: w1601 -> [w1627]
                  tunnel: w1604 -> [w1631]
                  tunnel: w1602 -> [w1630]
                  frame #0 {
                    w1610 = i16 2 ("precision (6)")
                    w1611 = i16 5 ("width (-)")
                    w1613 = 100.0 ("y")
                    n1038 = Multiply(x=w1612, y=w1624) -> (x*y=w1625:dbl)
                    n1039 = Add(x=0.0, y=w1625) -> (x+y=w1614:dbl)
                    n1040 = Multiply(x=w1616, y=w1613) -> (x*y=w1617:dbl)
                    n1041 = Multiply(x=w1614, y=w1613) -> (x*y=w1615:dbl)
                    n1042 = Build Array(w1614, w1616) -> (w1623:dbl[])
                    n1043 = Number To Fractional String(number=w1616, width (-)=w1611, precision (6)=w1610) -> (F-format string=→"moveY":string)  [unwired: 1 in]
                    n1044 = Number To Decimal String(number=w1617) -> (decimal integer string=w1618:string)  [unwired: 1 in]
                    n1045 = Number To Decimal String(number=w1615) -> (decimal integer string=w1619:string)  [unwired: 1 in]
                    n1046 = Number To Fractional String(number=w1614, width (-)=w1611, precision (6)=w1610) -> (F-format string=→"moveX":string)  [unwired: 1 in]
                    n1047 = Array To Cluster(array=w1623) -> (cluster=w1622:cluster{"[0]":dbl, "[1]":dbl})
                    n1048 = property on="Trap position (V)" class="Clust (strict)"("Val(Sgnl)"=w1622) -> ()  [unwired: 2 in, 2 out]
                  }
                  frame #1 {
                    n1049 = Wait (ms)(milliseconds to wait=u32 1000) -> ()  [unwired: 1 out]
                  }
                  frame #2 {
                    n1050 = while {
                      tunnel: w1631 -> [w1633]
                      tunnel: w1630 -> [w1632]
                      i -> [w1636]
                      stop <- w1634 stop-if-true
                      n1051 = flat-sequence {
                        tunnel: w1633 -> [w1640]
                        tunnel: w1632 -> [w1639]
                        frame #0 {
                          w1637 = "_" ("string")
                          n1052 = local read "Image Index"() -> (w1649:dbl)
                          n1053 = Concatenate Strings("GridMove_" ("string"), w1640, w1637, w1639, w1637) -> (w1638:string)
                          n1054 = call "Create new save file.vi"("Insert"=w1638, "Ext"=".bmp" ("string"), "Index In"=w1649) -> ("Path Out"=w1645:path, "Index Out"=w1647:dbl)
                          n1055 = local read "GreyscaleArray"() -> (w1643:u32[])
                          n1056 = local read "image8bitArray"() -> (w1644:u8[][])
                          n1057 = Increment(x=w1647) -> (x+1=w1646:dbl)
                          n1058 = local write "Image Index"(w1646) -> ()
                          n1059 = call <vilib>:"Flatten Pixmap.vi"("colors"=w1643, "8-bit pixmap"=w1644) -> ("image data"=w1642:T17)  [unwired: 4 in, 5 out]
                          n1060 = call <vilib>:"Write BMP File.vi"("image data"=w1642, "path to BMP file"=w1645) -> ()  [unwired: 1 in, 9 out]
                        }
                        frame #1 {
                          n1061 = Wait (ms)(milliseconds to wait=u32 50) -> ()  [unwired: 1 out]
                        }
                      }
                      n1062 = Equal?(x=w1636, y=9) -> (x = y?=w1634:bool)
                    }
                  }
                  frame #3 {
                    n1063 = Wait (ms)(milliseconds to wait=u32 100) -> ()  [unwired: 1 out]
                  }
                }
                n1064 = Equal?(x=w1606, y=5.0) -> (x = y?=w1608:bool)
              }
              n1065 = local read "Stop"() -> (w1593:bool)
              n1066 = Equal?(x=w1595, y=2.0) -> (x = y?=w1592:bool)
              n1067 = Or(x=w1593, y=w1592) -> (x .or. y?=w1591:bool)
            }
          }
          frame #2 {
            n1068 = property on="Shutter 2 (A)" class="Bool (strict)"("Val(Sgnl)"=FALSE ("Shutter 2 (A)")) -> ()  [unwired: 2 in, 2 out]
            n1069 = property on="Inject Sample" class="Bool (strict)"("Val(Sgnl)"=TRUE ("Inject Sample")) -> ()  [unwired: 2 in, 2 out]
          }
          frame #3 {
            n1070 = Wait (ms)(milliseconds to wait=u32 10000) -> ()  [unwired: 1 out]
          }
          frame #4 {
            n1071 = property on="Inject Sample" class="Bool (strict)"("Val(Sgnl)"=FALSE ("Inject Sample")) -> ()  [unwired: 2 in, 2 out]
          }
          frame #5 {
            n1072 = while {
              i -> [w1658]
              stop <- w1656 stop-if-true
              n1073 = flat-sequence {
                frame #0 {
                  n1074 = local read "image8bitArray"() -> (w1667:u8[][])
                  n1075 = local read "GreyscaleArray"() -> (w1666:u32[])
                  n1076 = local read "Image Index"() -> (w1665:dbl)
                  n1077 = call "Create new save file.vi"("Insert"="background_" ("string"), "Ext"=".bmp" ("string"), "Index In"=w1665) -> ("Path Out"=w1660:path, "Index Out"=w1662:dbl)
                  n1078 = call <vilib>:"Flatten Pixmap.vi"("colors"=w1666, "8-bit pixmap"=w1667) -> ("image data"=w1659:T17)  [unwired: 4 in, 5 out]
                  n1079 = Increment(x=w1662) -> (x+1=w1661:dbl)
                  n1080 = call <vilib>:"Write BMP File.vi"("image data"=w1659, "path to BMP file"=w1660) -> ()  [unwired: 1 in, 9 out]
                  n1081 = local write "Image Index"(w1661) -> ()
                }
                frame #1 {
                  n1082 = Wait (ms)(milliseconds to wait=u32 500) -> ()  [unwired: 1 out]
                }
              }
              n1083 = Equal?(x=w1658, y=9) -> (x = y?=w1656:bool)
            }
          }
          frame #6 {
            n1084 = local write "Grid Movable Trap"(FALSE ("Grid Movable Trap")) -> ()
          }
        }
      }
      event "Repeat Dip": Value Change {
        n1085 = event-data() -> ()  [unwired: 1 in, 6 out]
        n1086 = local read "Saved stage positions"() -> (w1673:dbl[][])
        n1087 = local read "Calibrating"() -> (w1676:bool)
        n1088 = local read "Saving Move"() -> (w1675:bool)
        n1089 = Not(x=w1676) -> (.not. x?=w1674:bool)
        n1090 = And(x=w1675, y=w1674) -> (x .and. y?=w1671:bool)
        n1091 = flat-sequence {
          tunnel: w1673 -> [w1680]
          tunnel: w1672 -> [w1679]
          tunnel: w1671 -> [w1678]
          tunnel: w1670 -> [w1677]
          frame #0 {
            n1092 = while {
              tunnel: w1680 -> [w1700]
              tunnel: w1679 -> [w1697]
              tunnel: w1678 -> [w1694]
              tunnel: w1678 -> [w1693]
              tunnel: w1677 -> [w1692]
              tunnel: w1677 -> [w1691]
              i -> [w1701]
              stop <- w1682 stop-if-true
              n1093 = flat-sequence {
                tunnel: w1700 -> [w1706]
                tunnel: [w1706] -> w1698
                tunnel: w1697 -> [w1705]
                tunnel: [w1705] -> w1695
                tunnel: w1694 -> [w1704]
                tunnel: w1692 -> [w1703]
                tunnel: [w1702] -> w1687
                tunnel: [w1719] -> w1699
                tunnel: w1698 -> [w1719]
                tunnel: [w1718] -> w1696
                tunnel: w1695 -> [w1718]
                tunnel: w1693 -> [w1717]
                tunnel: w1687 -> [w1716]
                tunnel: w1681 -> [w1715]
                tunnel: w1699 -> [w1753]
                tunnel: w1696 -> [w1752]
                tunnel: w1693 -> [w1751]
                tunnel: w1691 -> [w1750]
                tunnel: [w1749] -> w1686
                tunnel: w1693 -> [w1764]
                tunnel: w1686 -> [w1763]
                tunnel: w1681 -> [w1762]
                frame #0 {
                  n1094 = case shown="True" w1704 {
                    frame False {
                    }
                    frame True {
                      n1095 = Get Date/Time In Seconds() -> (seconds since 1Jan1904=w1714:timestamp)
                      n1096 = call <vilib>:"Space Constant.vi"() -> ("String"=w1710:string)
                      n1097 = Format Date/Time String(time format string (%c)="%H:%M:%S%3u", seconds (now)=w1714, UTC format=TRUE) -> (date/time string=w1711:string)
                      n1098 = Concatenate Strings(w1711, w1710, "moving") -> (w1708:string)
                      n1099 = property on="Move time" class="Str"("Val(Sgnl)"=w1708) -> ()  [unwired: 2 in, 2 out]
                    }
                  }
                  n1100 = local read "Dip position"() -> (w1702:dbl)
                  n1101 = local write "Stage moving"(TRUE) -> ()
                  n1102 = call "move to saved stage position.vi"("error in"=w1703, "Stage VISA resource name in"=w1705, "Position"=w1702, "Saved Stage Positions"=w1706) -> ()  [unwired: 2 out]
                }
                frame #1 {
                  # "IN DIPPING POSITION"
                  n1103 = node-c288() -> (w1722:T13)  [unwired: 4 in]
                  n1104 = case shown="True" w1717 {
                    tunnel: w1716 -> [_ w1727]
                    frame False {
                    }
                    frame True {
                      n1105 = Get Date/Time In Seconds() -> (seconds since 1Jan1904=w1731:timestamp)
                      n1106 = Format Date/Time String(time format string (%c)="%H:%M:%S%3u", seconds (now)=w1731, UTC format=TRUE) -> (date/time string=w1726:string)
                      n1107 = Number To Decimal String(number=w1727, width (-)=i16 1) -> (decimal integer string=w1724:string)
                      n1108 = call <vilib>:"Space Constant.vi"() -> ("String"=w1725:string)
                      n1109 = Concatenate Strings(w1726, w1725, w1724) -> (w1723:string)
                      n1110 = property on="Move time" class="Str"("Val(Sgnl)"=w1723) -> ()  [unwired: 2 in, 2 out]
                    }
                  }
                  n1111 = timed-loop {
                    timing: w1722 -> [_]
                    timing-out: [_] -> w1721
                    tunnel: w1715 -> [w1732]
                    i -> [w1742]
                    stop <- w1734 stop-if-true
                    n1112 = node-c288() -> ()  [unwired: 1 in, 1 out]
                    n1113 = local read "Cancel dwell"() -> (w1740:bool)
                    n1114 = local read "Dip duration"() -> (w1741:dbl)
                    n1115 = local write "Dip elasped time"(w1742) -> ()
                    n1116 = local read "Dump beads"() -> (w1735:bool)
                    n1117 = To Double Precision Float(number=w1742) -> (double precision float=w1743:dbl)
                    n1118 = local read "Pause dwell"() -> (w1744:bool)
                    n1119 = Greater Or Equal?(x=w1743, y=w1741) -> (x >= y?=w1739:bool)
                    n1120 = Or(x=w1739, y=w1740) -> (x .or. y?=w1738:bool)
                    n1121 = Not(x=w1744) -> (.not. x?=w1737:bool)
                    n1122 = local read "Cancel Rep\n Dip"() -> (w1733:bool)
                    n1123 = And(x=w1737, y=w1738) -> (x .and. y?=w1736:bool)
                    n1124 = node-c288() -> ()  [unwired: 1 in, 1 out]
                    n1125 = Compound Arithmetic op=OR(w1733, w1736, w1735, w1732) -> (w1734:bool)
                  }
                  n1126 = local write "Stage moving"(FALSE) -> ()
                  n1127 = node-c288(w1721) -> ()  [unwired: 1 out]
                }
                frame #2 {
                  n1128 = case shown="True" w1751 {
                    frame False {
                    }
                    frame True {
                      n1129 = Get Date/Time In Seconds() -> (seconds since 1Jan1904=w1761:timestamp)
                      n1130 = call <vilib>:"Space Constant.vi"() -> ("String"=w1757:string)
                      n1131 = Format Date/Time String(time format string (%c)="%H:%M:%S%3u", seconds (now)=w1761, UTC format=TRUE) -> (date/time string=w1758:string)
                      n1132 = Concatenate Strings(w1758, w1757, "moving") -> (w1755:string)
                      n1133 = property on="Move time" class="Str"("Val(Sgnl)"=w1755) -> ()  [unwired: 2 in, 2 out]
                    }
                  }
                  n1134 = local read "Start/Return position"() -> (w1749:dbl)
                  n1135 = local write "Stage moving"(TRUE) -> ()
                  n1136 = call "move to saved stage position.vi"("error in"=w1750, "Stage VISA resource name in"=w1752, "Position"=w1749, "Saved Stage Positions"=w1753) -> ()  [unwired: 2 out]
                }
                frame #3 {
                  # "IN RETURN POSITION"
                  n1137 = node-c288() -> (w1767:T13)  [unwired: 4 in]
                  n1138 = timed-loop {
                    timing: w1767 -> [_]
                    timing-out: [_] -> w1766
                    tunnel: w1762 -> [w1777]
                    i -> [w1788]
                    stop <- w1779 stop-if-true
                    n1139 = node-c288() -> ()  [unwired: 1 in, 1 out]
                    n1140 = local read "Return duration"() -> (w1786:dbl)
                    n1141 = local read "Dump beads"() -> (w1780:bool)
                    n1142 = local read "Cancel dwell"() -> (w1784:bool)
                    n1143 = local write "Return elasped time"(w1788) -> ()
                    n1144 = To Double Precision Float(number=w1788) -> (double precision float=w1789:dbl)
                    n1145 = local read "Pause dwell"() -> (w1787:bool)
                    n1146 = Greater Or Equal?(x=w1789, y=w1786) -> (x >= y?=w1785:bool)
                    n1147 = Or(x=w1785, y=w1784) -> (x .or. y?=w1783:bool)
                    n1148 = local read "Cancel Rep\n Dip"() -> (w1778:bool)
                    n1149 = Not(x=w1787) -> (.not. x?=w1782:bool)
                    n1150 = node-c288() -> ()  [unwired: 1 in, 1 out]
                    n1151 = And(x=w1782, y=w1783) -> (x .and. y?=w1781:bool)
                    n1152 = Compound Arithmetic op=OR(w1778, w1781, w1780, w1777) -> (w1779:bool)
                  }
                  n1153 = case shown="True" w1764 {
                    tunnel: w1763 -> [_ w1772]
                    frame False {
                    }
                    frame True {
                      n1154 = Get Date/Time In Seconds() -> (seconds since 1Jan1904=w1776:timestamp)
                      n1155 = Format Date/Time String(time format string (%c)="%H:%M:%S%3u", seconds (now)=w1776, UTC format=TRUE) -> (date/time string=w1769:string)
                      n1156 = Number To Decimal String(number=w1772, width (-)=i16 1) -> (decimal integer string=w1771:string)
                      n1157 = call <vilib>:"Space Constant.vi"() -> ("String"=w1770:string)
                      n1158 = Concatenate Strings(w1769, w1770, w1771) -> (w1768:string)
                      n1159 = property on="Move time" class="Str"("Val(Sgnl)"=w1768) -> ()  [unwired: 2 in, 2 out]
                    }
                  }
                  n1160 = local write "Stage moving"(FALSE) -> ()
                  n1161 = node-c288(w1766) -> ()  [unwired: 1 out]
                }
              }
              n1162 = local read "Tether"() -> (w1683:bool)
              n1163 = Not(x=w1683) -> (.not. x?=w1681:bool)
              n1164 = Increment(x=w1701) -> (x+1=w1689:i32)
              "Dip #" <- w1689
              n1165 = property on="Cancel Rep\n Dip" class="Bool (strict)"() -> ("Value"=w1685:bool)  [unwired: 2 in, 2 out]
              n1166 = To Double Precision Float(number=w1689) -> (double precision float=w1688:dbl)
              n1167 = Greater Or Equal?(x=w1688, y="Dip attempts") -> (x >= y?=w1684:bool)
              n1168 = Compound Arithmetic op=OR(w1685, w1684, w1681) -> (w1682:bool)
            }
          }
          frame #1 {
            w1794 = FALSE
            n1169 = local write "Cancel Rep\n Dip"(w1794) -> ()
            n1170 = call <vilib>:"Beep.vi"() -> ()  [unwired: 12 in]
            n1171 = local write "Repeat Dip"(w1794) -> ()
          }
        }
      }
      event "Force FB script": Value Change {
        n1172 = event-data() -> ()  [unwired: 1 in, 5 out]
        n1173 = flat-sequence {
          frame #0 {
            n1174 = disable-structure shown="Disabled" {
              frame Disabled {
                n1175 = local read "# Samples/channel"() -> (w1797:i32)
                n1176 = local write "# Samples/channel (in)"(w1797) -> ()
              }
              frame Enabled {
              }
            }
            n1177 = local write "Force FB script"(FALSE ("Force FB script")) -> ()
            n1178 = property on="Trap delta (nm)" class="DigNum (strict)"("Val(Sgnl)"="Start trap delta (nm)") -> ()  [unwired: 2 in, 2 out]
          }
          frame #1 {
            n1179 = Wait (ms)(milliseconds to wait=u32 500) -> ()  [unwired: 1 out]
          }
          frame #2 {
            n1180 = property on="Set reading to\nsetpoint 1" class="Bool (strict)"("Val(Sgnl)"=TRUE ("Value (Signaling)")) -> ()  [unwired: 2 in, 2 out]
          }
          frame #3 {
            n1181 = Wait (ms)(milliseconds to wait=u32 300) -> ()  [unwired: 1 out]
          }
          frame #4 {
            n1182 = local write "Force Feedback 1"(TRUE ("Force Feedback")) -> ()
            n1183 = property on="Tabs" class="TabCtl (strict)"("Val(Sgnl)"=T23."Force Feedback" ("Value (Signaling)")) -> ()  [unwired: 2 in, 2 out]
          }
          frame #5 {
            n1184 = property on="Save Data" class="Bool (strict)"("Val(Sgnl)"=TRUE ("Value (Signaling)")) -> ()  [unwired: 2 in, 2 out]
          }
          frame #6 {
            n1185 = Multiply(x="Wait before dip (s)", y=1000) -> (x*y=w1804:dbl)
            n1186 = Wait (ms)(milliseconds to wait=w1804) -> ()  [unwired: 1 out]
          }
          frame #7 {
            n1187 = case shown="True" "Start dipping after?" {
              selector: "Start dipping after?" -> [_ w1809]
              frame False {
              }
              frame True {
                n1188 = property on="Dip" class="Bool (strict)"("Val(Sgnl)"=w1809) -> ()  [unwired: 2 in, 2 out]
              }
            }
            n1189 = property on="Remove offsets" class="Bool (strict)"("Val(Sgnl)"=TRUE ("Value (Signaling)")) -> ()  [unwired: 2 in, 2 out]
          }
        }
      }
      event "Move 0": Value Change {
        n1190 = event-data() -> ()  [unwired: 1 in, 5 out]
        n1191 = local write "Move 0"(FALSE) -> ()
        n1192 = call "HalfWavePlate.vi"("Degrees"="\"Degrees\" 0", "Motor"=0) -> ()  [unwired: 1 in]
      }
      event "Move 1": Value Change {
        n1193 = event-data() -> ()  [unwired: 1 in, 5 out]
        n1194 = local write "Move 1"(FALSE) -> ()
        n1195 = call "HalfWavePlate.vi"("Degrees"="\"Degrees\" 1", "Motor"=1) -> ()  [unwired: 1 in]
      }
      event "Save user params": Value Change {
        n1196 = event-data() -> ()  [unwired: 1 in, 6 out]
        n1197 = local write "Save user params"(FALSE) -> ()
        n1198 = call "save control values.vi"("User"="User") -> ()  [unwired: 8 in, 1 out]
      }
      event "Load user params": Value Change {
        # "Exceptions. Don't load these parameters."
        n1199 = event-data() -> ()  [unwired: 1 in, 6 out]
        n1200 = local write "Load user params"(FALSE) -> ()
        n1201 = flat-sequence {
          tunnel: [w1842] -> w1833
          tunnel: [w1841] -> w1831
          tunnel: [w1840] -> w1829
          tunnel: [w1839] -> w1827
          tunnel: [w1838] -> w1825
          tunnel: [w1837] -> w1823
          tunnel: [w1836] -> w1821
          tunnel: [w1835] -> w1818
          tunnel: [w1850] -> w1834
          tunnel: w1833 -> [w1850]
          tunnel: [w1849] -> w1832
          tunnel: w1831 -> [w1849]
          tunnel: [w1848] -> w1830
          tunnel: w1829 -> [w1848]
          tunnel: [w1847] -> w1828
          tunnel: w1827 -> [w1847]
          tunnel: [w1846] -> w1826
          tunnel: w1825 -> [w1846]
          tunnel: [w1845] -> w1824
          tunnel: w1823 -> [w1845]
          tunnel: [w1844] -> w1822
          tunnel: w1821 -> [w1844]
          tunnel: [w1843] -> w1819
          tunnel: w1818 -> [w1843]
          tunnel: w1834 -> [w1859]
          tunnel: w1832 -> [w1858]
          tunnel: w1830 -> [w1857]
          tunnel: w1828 -> [w1856]
          tunnel: w1826 -> [w1855]
          tunnel: w1824 -> [w1854]
          tunnel: w1822 -> [w1853]
          tunnel: w1819 -> [w1852]
          frame #0 {
            n1202 = local read "Force Feedback 2"() -> (w1835:bool)
            n1203 = local read "Force Feedback 1"() -> (w1836:bool)
            n1204 = local read "Shutter 1 (B)"() -> (w1842:bool)
            n1205 = local read "Shutter 2 (A)"() -> (w1841:bool)
            n1206 = local read "Inject Sample"() -> (w1839:bool)
            n1207 = local read "Trap delta (nm)"() -> (w1838:dbl)
            n1208 = local read "Save file index"() -> (w1837:i32)
            n1209 = local read "Fish"() -> (w1840:bool)
          }
          frame #1 {
            n1210 = local read "User"() -> (w1851:string)
            n1211 = call "retrieve control values.vi"("User"=w1851) -> ()  [unwired: 10 in, 1 out]
          }
          frame #2 {
            n1212 = local write "Force Feedback 1"(w1853) -> ()
            n1213 = local write "Force Feedback 2"(w1852) -> ()
            n1214 = local write "Trap delta (nm)"(w1855) -> ()
            n1215 = local write "Save file index"(w1854) -> ()
            n1216 = local write "Inject Sample"(w1856) -> ()
            n1217 = local write "Shutter 2 (A)"(w1858) -> ()
            n1218 = local write "Shutter 1 (B)"(w1859) -> ()
            n1219 = local write "Fish"(w1857) -> ()
          }
        }
      }
      event "Stop": Value Change {
        n1220 = event-data() -> ()  [unwired: 1 in, 5 out]
        n1221 = local read "Stop"() -> (w1860:bool)
      }
    }
    n1222 = node-c288() -> ()  [unwired: 1 in, 1 out]
  }
  n1223 = call-poly <vilib>:"DAQmx Create Virtual Channel.vi"("lines"=w98) -> ("task out"=w97:refnum<k21>)  [unwired: 13 in, 1 out]
  n1224 = call-poly <vilib>:"DAQmx Create Virtual Channel.vi"("lines"=w101) -> ("task out"=w100:refnum<k21>)  [unwired: 13 in, 1 out]
  n1225 = node-c288(2 ("Processor")) -> (w82:T13)  [unwired: 3 in]
  n1226 = timed-loop {
    timing: w82 -> [_]
    timing-out: [_] -> w81
    stop <- w1863 stop-if-true
    n1227 = node-c288() -> ()  [unwired: 1 in, 1 out]
    n1228 = case shown="\"Control\"" "Tab Control" {
      frame "Control" {
        n1229 = case shown="True" "Start" {
          frame False {
          }
          frame True {
            w1876 = T24 3 items=["no dialog", "OK message", "continue or stop message", "OK message + warnings", "continue/stop + warnings"] ("type of dialog (OK msg:1)")
            n1230 = call "InitializeAcquireFF.vi"("DAQ Rate"="DAQ Rate", "Averaging Number"="Averaging Number", "Sampling Rate"="Sampling Rate") -> ("error out"=w1870:errorcluster, "task out"=w1869:refnum<k21>, "Final Sampling Rate"=→"Final Sampling Rate":dbl)  [unwired: 4 in, 2 out]
            n1231 = while {
              tunnel: [w1888] -> w1875
              tunnel: [w1887] -> w1868
              tunnel: "Averaging Number" -> [w1886]
              tunnel: w1870 -> [w1885]
              tunnel: w1869 -> [w1883]
              stop <- w1884 continue-if-true
              n1232 = call "Acquire2_QPD.vi"("task/channels in"=w1883, "Save Data?"=FALSE ("Take Data?"), "Averaging Number"=w1886, "error in"=w1885) -> ("PSD 1"=→"PSD 1":cluster{dbl[], dbl[]}, "PSD 1 Sum"=→"PSD 1 Sum":dbl, "PSD 2"=→"PSD 2":cluster{dbl[], dbl[]}, "PSD 2 Sum"=→"PSD 2 Sum":dbl, "task out"=w1888:refnum<k21>, "error out"=w1887:errorcluster)  [unwired: 14 in, 4 out]
              n1233 = local read "Start"() -> (w1884:bool)
            }
            n1234 = call <vilib>:"DAQmx Clear Task.vi"("task in"=w1875, "error in"=w1868) -> ("error out"=w1877:errorcluster)  [unwired: 13 in]
            n1235 = call <vilib>:"Simple Error Handler.vi"("type of dialog (OK msg:1)"=w1876, "error in (no error)"=w1877) -> ()  [unwired: 3 in, 5 out]
          }
        }
      }
      frame "Current Saved Data" {
      }
      frame "Data Acquisition" {
      }
      frame "Raw QPD Data" {
      }
    }
    n1236 = local read "Stop"() -> (w1863:bool)
    n1237 = node-c288() -> ()  [unwired: 1 in, 1 out]
  }
  n1238 = node-c288(2 ("Processor")) -> (w34:T13)  [unwired: 3 in]
  n1239 = timed-loop {
    timing: w34 -> [_]
    timing-out: [_] -> w33
    stop <- w1889 stop-if-true
    n1240 = node-c288() -> ()  [unwired: 1 in, 1 out]
    n1241 = event shown="[0] \"Pause Mouse/Mirror Connection\": Value Change" {
      selector: _ -> [_ _]
      dyn-events: _ -> [_ _]
      timeout: _ -> [_ _]
      tunnel: [w1982 _] -> w1890
      tunnel: [_ w1983] -> w1889
      event "Pause Mouse/Mirror Connection": Value Change {
        n1242 = event-data() -> ("NewVal"=w1982:bool)  [unwired: 1 in]
      }
      event "Stop": Value Change {
        n1243 = event-data() -> ("NewVal"=w1983:bool)  [unwired: 1 in]
      }
    }
    n1244 = case shown="True" w1890 {
      frame False {
      }
      frame True {
        n1245 = call "InitializeMouseControl.vi"() -> ("error out 2"=w1899:errorcluster, "task out"=w1900:refnum<k21>, "error out"=w1902:errorcluster, "device ID"=w1901:refnum<k1>)  [unwired: 8 in]
        n1246 = while {
          tunnel: w1902 -> [w1914]
          tunnel: w1901 -> [w1913]
          tunnel: w1900 -> [w1912]
          tunnel: w1899 -> [w1911]
          tunnel: [w1910] -> w1897
          tunnel: [w1909] -> w1896
          tunnel: [w1908] -> w1893
          tunnel: [w1907] -> w1894
          stop <- w1906 stop-if-true
          n1247 = case shown="True" "Use Mouse to Move Trap?" {
            tunnel: w1913 -> [w1921 w1944]
            tunnel: w1914 -> [w1920 w1943]
            tunnel: w1912 -> [w1919 w1942]
            tunnel: w1911 -> [w1918 w1941]
            tunnel: [w1921 w1940] -> w1908
            tunnel: [w1920 w1939] -> w1907
            tunnel: [w1919 w1938] -> w1910
            tunnel: [w1918 w1937] -> w1909
            frame False {
              (unwired) FALSE ("button 1")
            }
            frame True {
              w1932 = 0.0 ("y")
              w1934 = 10
              n1248 = local read "Deflection"() -> (w1945:T5)
              n1249 = call-poly <vilib>:"Acquire Input Data.vi"("device ID"=w1944, "error in (no error)"=w1943) -> ("device ID"=w1940:refnum<k1>, "button info"=w1958:T25, "error out"=w1939:errorcluster)  [unwired: 14 in, 1 out]
              n1250 = Unbundle By Name(w1945) -> ("Horizontal"=w1947:i32, "Vertical"=w1946:i32)
              n1251 = local read "Saved voltage"() -> (w1923:cluster{dbl, dbl})
              n1252 = Divide(x=w1947, y=30) -> (x/y=w1950:dbl)
              n1253 = Divide(x=w1946, y=-20) -> (x/y=w1951:dbl)
              n1254 = Unbundle By Name(w1958) -> ("button 1"=w1936:bool, "button 2"=w1952:bool)
              n1255 = Bundle(w1950, w1951) -> (w1928:cluster{dbl, dbl})  [unwired: 1 in]
              n1256 = local write "Reference Voltage"(w1928) -> ()
              n1257 = Add(x=w1928, y=w1923) -> (x+y=w1956:cluster{dbl, dbl})
              n1258 = case shown="True" w1936 {
                frame False {
                  n1259 = stacked-sequence {
                    frame #0 {
                      n1260 = local write "CoordinatesMousePressed"(T5 {"Horizontal"=0, "Vertical"=0} ("Coords when pressed")) -> ()
                      n1261 = local write "Deflection"(T5 {"Horizontal"=0, "Vertical"=0} ("deflaction")) -> ()
                    }
                  }
                }
                frame True {
                  n1262 = local read "CoordinatesMousePressed"() -> (w1981:T5)
                  n1263 = local read "Real Coordinates"() -> (w1980:cluster{"Horizontal":i32, "Vertical":i32})
                  n1264 = Subtract(x=w1980, y=w1981) -> (x-y=w1979:T5)
                  n1265 = local write "Deflection"(w1979) -> ()
                }
              }
              n1266 = Unbundle(w1956) -> (w1933:dbl, w1924:dbl)
              n1267 = case shown="True" w1952 {
                frame False {
                }
                frame True {
                  n1268 = local read "Reference Voltage"() -> (w1962:cluster{dbl, dbl})
                  n1269 = local read "Saved voltage"() -> (w1960:cluster{dbl, dbl})
                  n1270 = Add(x=w1962, y=w1960) -> (x+y=→"Saved voltage":cluster{dbl, dbl})
                  n1271 = local read "Real Coordinates"() -> (w1961:cluster{"Horizontal":i32, "Vertical":i32})
                  n1272 = local write "CoordinatesMousePressed"(w1961) -> ()
                }
              }
              n1273 = Less?(x=w1933, y=w1934) -> (x < y?=w1931:bool)
              n1274 = Greater?(x=w1933, y=w1932) -> (0:w1930:bool)
              n1275 = Greater?(x=w1924, y=w1932) -> (0:w1926:bool)
              n1276 = Less?(x=w1924, y=w1934) -> (x < y?=w1927:bool)
              n1277 = And(x=w1926, y=w1927) -> (x .and. y?=w1925:bool)
              n1278 = And(x=w1931, y=w1930) -> (x .and. y?=w1929:bool)
              n1279 = case shown="False" w1925 {
                tunnel: [w1972 w1976] -> w1935
                tunnel: w1924 -> [w1970 w1976]
                frame False {
                  n1280 = Greater?(x=w1970, y=10.0) -> (0:w1973:bool)
                  n1281 = case shown="True" w1973 {
                    tunnel: [0.0 10.0] -> w1972
                    frame False {
                    }
                    frame True {
                    }
                  }
                }
                frame True {
                }
              }
              n1282 = case shown="False" w1929 {
                tunnel: w1933 -> [w1964 w1969]
                tunnel: [w1965 w1969] -> w1957
                frame False {
                  n1283 = Greater?(x=w1964, y=10.0) -> (0:w1966:bool)
                  n1284 = case shown="True" w1966 {
                    tunnel: [0.0 10.0] -> w1965
                    frame False {
                    }
                    frame True {
                    }
                  }
                }
                frame True {
                }
              }
              n1285 = Bundle(w1957, w1935) -> (w1922:cluster{dbl, dbl})  [unwired: 1 in]
              n1286 = Cluster To Array(cluster=w1922) -> (array=w1953:dbl[])
              n1287 = call-poly <vilib>:"DAQmx Write.vi"("task/channels in"=w1942, "data"=w1953, "error in"=w1941) -> ("task out"=w1955:refnum<k21>, "error out"=w1954:errorcluster)  [unwired: 10 in, 1 out]
              n1288 = call <vilib>:"DAQmx Is Task Done.vi"("task/channels in"=w1955, "error in"=w1954) -> ("task out"=w1938:refnum<k21>, "error out"=w1937:errorcluster)  [unwired: 11 in, 1 out]
            }
          }
          n1289 = event shown="[0] \"Pane\": Mouse Move" {
            selector: _ -> [_ _ _]
            dyn-events: _ -> [_ _ _]
            timeout: _ -> [_ _ _]
            event Mouse Move {
              n1290 = event-data() -> ("Coords"=w1916:T5)  [unwired: 1 in]
              n1291 = local write "Real Coordinates"(w1916) -> ()
            }
            event Mouse Down {
              n1292 = event-data() -> ("Coords"=w1917:T5)  [unwired: 1 in]
              n1293 = local write "CoordinatesMousePressed"(w1917) -> ()
            }
            event "Pause Mouse/Mirror Connection": Value Change {
              n1294 = event-data() -> ()  [unwired: 1 in, 3 out]
            }
          }
          n1295 = local read "Stop"() -> (w1903:bool)
          n1296 = Not(x="Pause Mouse/Mirror Connection") -> (.not. x?=w1904:bool)
          n1297 = Or(x=w1904, y=w1903) -> (x .or. y?=w1906:bool)
        }
        n1298 = call <vilib>:"DAQmx Clear Task.vi"("task in"=w1897, "error in"=w1896) -> ("error out"=w1898:errorcluster)  [unwired: 13 in]
        n1299 = call <vilib>:"Simple Error Handler.vi"("error in (no error)"=w1898) -> ()  [unwired: 4 in, 5 out]
        n1300 = call-poly <vilib>:"Close Input Device.vi"("error in (no error)"=w1894, "device ID"=w1893) -> ("error out"=w1895:errorcluster)  [unwired: 8 in]
        n1301 = call <vilib>:"Simple Error Handler.vi"("error in (no error)"=w1895) -> ()  [unwired: 4 in, 5 out]
      }
    }
    n1302 = node-c288() -> ()  [unwired: 1 in, 1 out]
  }
  n1303 = node-c288(i64 100 ("Period")) -> (w95:T13)  [unwired: 3 in]
  n1304 = timed-loop {
    tunnel: w97 -> [w1986]
    tunnel: [w1985] -> w96
    tunnel: w100 -> [w1988]
    tunnel: [w1987] -> w99
    timing: w95 -> [_]
    timing-out: [_] -> w94
    stop <- w1984 stop-if-true
    n1305 = node-c288() -> ()  [unwired: 1 in, 1 out]
    n1306 = event shown="[1] \"Shutter 2 (A)\": Value Change" {
      selector: _ -> [_ _ _]
      dyn-events: _ -> [_ _ _]
      timeout: _ -> [_ _ _]
      tunnel: w1988 -> [w1992 _ w2029]
      tunnel: [w1991 _ w2029] -> w1987
      tunnel: w1986 -> [_ w2012 w2030]
      tunnel: [_ w2010 w2030] -> w1985
      tunnel: [_ _ w2031] -> w1984
      event "Shutter 1 (B)": Value Change {
        n1307 = event-data() -> ()  [unwired: 1 in, 1 out]
        n1308 = flat-sequence {
          tunnel: [w1998] -> w1995
          tunnel: w1992 -> [w1997]
          tunnel: [w2002] -> w1994
          tunnel: [w2005] -> w1993
          tunnel: w1995 -> [w2000]
          tunnel: w1994 -> [w2009]
          tunnel: w1993 -> [w2007]
          tunnel: [w2006] -> w1991
          frame #0 {
            n1309 = call-poly <vilib>:"DAQmx Write.vi"("task/channels in"=w1997, "data"=FALSE) -> ("task out"=w1998:refnum<k21>)  [unwired: 11 in, 2 out]
            n1310 = Wait (ms)(milliseconds to wait=100) -> ()  [unwired: 1 out]
          }
          frame #1 {
            n1311 = Or(x="Shutter 1 (B)", y=TRUE) -> (x .or. y?=w2002:bool)
            n1312 = call-poly <vilib>:"DAQmx Write.vi"("task/channels in"=w2000, "data"=w2002) -> ("task out"=w2005:refnum<k21>)  [unwired: 11 in, 2 out]
            n1313 = Wait (ms)(milliseconds to wait=100) -> ()  [unwired: 1 out]
          }
          frame #2 {
            n1314 = Not(x=w2009) -> (.not. x?=w2008:bool)
            n1315 = call-poly <vilib>:"DAQmx Write.vi"("task/channels in"=w2007, "data"=w2008) -> ("task out"=w2006:refnum<k21>)  [unwired: 11 in, 2 out]
          }
        }
      }
      event "Shutter 2 (A)": Value Change {
        n1316 = event-data() -> ()  [unwired: 1 in, 1 out]
        n1317 = flat-sequence {
          tunnel: w2012 -> [w2017]
          tunnel: [w2016] -> w2011
          tunnel: [w2021] -> w2014
          tunnel: [w2024] -> w2013
          tunnel: w2011 -> [w2019]
          tunnel: w2014 -> [w2028]
          tunnel: w2013 -> [w2026]
          tunnel: [w2025] -> w2010
          frame #0 {
            n1318 = call-poly <vilib>:"DAQmx Write.vi"("task/channels in"=w2017, "data"=FALSE) -> ("task out"=w2016:refnum<k21>)  [unwired: 11 in, 2 out]
            n1319 = Wait (ms)(milliseconds to wait=100) -> ()  [unwired: 1 out]
          }
          frame #1 {
            n1320 = Or(x="Shutter 2 (A)", y=TRUE) -> (x .or. y?=w2021:bool)
            n1321 = call-poly <vilib>:"DAQmx Write.vi"("task/channels in"=w2019, "data"=w2021) -> ("task out"=w2024:refnum<k21>)  [unwired: 11 in, 2 out]
            n1322 = Wait (ms)(milliseconds to wait=100) -> ()  [unwired: 1 out]
          }
          frame #2 {
            n1323 = Not(x=w2028) -> (.not. x?=w2027:bool)
            n1324 = call-poly <vilib>:"DAQmx Write.vi"("task/channels in"=w2026, "data"=w2027) -> ("task out"=w2025:refnum<k21>)  [unwired: 11 in, 2 out]
          }
        }
      }
      event "Stop": Value Change {
        n1325 = event-data() -> ("NewVal"=w2031:bool)  [unwired: 1 in, 5 out]
      }
    }
    n1326 = node-c288() -> ()  [unwired: 1 in, 1 out]
  }
  n1327 = node-c288(w94) -> ()  [unwired: 1 out]
  n1328 = node-c288(w81) -> ()  [unwired: 1 out]
  n1329 = call <vilib>:"DAQmx Clear Task.vi"("task in"=w96) -> ()  [unwired: 14 in, 1 out]
  n1330 = call <vilib>:"DAQmx Clear Task.vi"("task in"=w99) -> ()  [unwired: 14 in, 1 out]
  n1331 = node-c288(w33) -> ()  [unwired: 1 out]
  n1332 = node-c288(w29) -> ()  [unwired: 1 out]
  n1333 = local write "Tether"(FALSE ("Tether")) -> ()
  n1334 = local read "Path"() -> (w88:path)
  n1335 = node-c288(i64 1 ("Period"), 2 ("Processor")) -> (w93:T13)  [unwired: 2 in]
  n1336 = timed-loop {
    timing: w93 -> [_]
    timing-out: [_] -> w92
    tunnel: w88 -> [w2033]
    stop <- w2032 stop-if-true
    n1337 = node-c288() -> ()  [unwired: 1 in, 1 out]
    n1338 = event shown="[1] \"Read Cal\": Value Change" {
      selector: _ -> [_ _ _ _ _ _ _ _ _ _]
      dyn-events: _ -> [_ _ _ _ _ _ _ _ _ _]
      timeout: _ -> [_ _ _ _ _ _ _ _ _ _]
      tunnel: w2033 -> [_ w2037 _ _ _ _ _ _ _ _]
      tunnel: [_ _ w2057 _ _ _ _ _ _ _] -> w2032
      event Timeout {
        n1339 = event-data() -> ()  [unwired: 1 in, 2 out]
      }
      event "Read Cal": Value Change {
        n1340 = event-data() -> ()  [unwired: 1 in, 6 out]
        n1341 = Path To String(path=w2037) -> (string=w2036:string)
        n1342 = Format Date/Time String(time format string (%c)="%y%m%d") -> (date/time string=w2038:string)  [unwired: 2 in]
        n1343 = Concatenate Strings(w2036, "\\" ("string"), w2038, "\\" ("string"), "current.cal") -> (w2056:string)
        n1344 = String To Path(string=w2056) -> (path=w2055:path)
        n1345 = Open/Create/Replace File(file path (use dialog)=w2055, operation (0:open)=T18."open", access (0:read/write)=enum16{"read/write", "read-only", "write-only"}."read-only") -> (refnum out=w2051:refnum<file>, error out=w2052:errorcluster)  [unwired: 3 in, 1 out]
        n1346 = Deny Access(4:w2052, 7:w2051) -> (0:w2050:errorcluster, 3:w2049:refnum<file>)  [unwired: 1 in]
        n1347 = Read from Binary File(5:0.0, 8:w2050, 9:T19."big-endian, network order" ("byte order (0:big-endian, network order)"), 10:12 ("count"), 11:w2049) -> (0:w2045:errorcluster, 2:w2043:dbl[], 3:w2046:refnum<file>)  [unwired: 1 in, 1 out]
        n1348 = Array To Cluster(array=w2043) -> (cluster=→"Cal values":T26)
        n1349 = Close File(refnum=w2046, error in=w2045) -> ()  [unwired: 2 out]
        n1350 = local write "Read Cal"(FALSE ("Read Cal")) -> ()
      }
      event "Stop": Value Change {
        n1351 = event-data() -> ("NewVal"=w2057:bool)  [unwired: 1 in, 5 out]
      }
      event "Trap position (V)": Value Change {
        # "Need to rotate so X and Y don't get mixed up."
        n1352 = event-data() -> ()  [unwired: 1 in, 6 out]
        n1353 = local read "Mirror task"() -> (w2058:refnum<k21>)
        n1354 = Cluster To Array(cluster="Trap position (V)") -> (array=w2061:dbl[])
        n1355 = Rotate 1D Array(1:w2061, 2:1 ("n")) -> (0:w2059:dbl[])
        n1356 = call-poly <vilib>:"DAQmx Write.vi"("task/channels in"=w2058, "data"=w2059) -> ("task out"=w2064:refnum<k21>, "error out"=w2063:errorcluster)  [unwired: 11 in, 1 out]
        n1357 = call <vilib>:"DAQmx Stop Task.vi"("task/channels in"=w2064, "error in"=w2063) -> ("error out"=w2062:errorcluster)  [unwired: 12 in, 1 out]
        n1358 = call <vilib>:"Simple Error Handler.vi"("error in (no error)"=w2062) -> ()  [unwired: 4 in, 5 out]
      }
      event "Trap delta (nm)": Value Change {
        n1359 = event-data() -> ()  [unwired: 1 in, 6 out]
        n1360 = local read "Pulling direction"() -> (w2066:bool)
        n1361 = local read "Conv Y (nm/V)"() -> (w2067:dbl)
        n1362 = local read "Conv X (nm/V)"() -> (w2068:dbl)
        n1363 = Select(t=w2067, s=w2066, f=w2068) -> (s? t:f=w2069:dbl)
        n1364 = local read "Fixed Y"() -> (w2075:dbl)
        n1365 = Divide(x="Trap delta (nm)", y=w2069) -> (x/y=w2070:dbl)
        n1366 = local read "Fixed X"() -> (w2074:dbl)
        n1367 = Select(t=w2075, s=w2066, f=w2074) -> (s? t:f=w2073:dbl)
        n1368 = Add(x=w2070, y=w2073) -> (x+y=w2071:dbl)
        n1369 = case shown="False" w2066 {
          tunnel: w2071 -> [w2076 w2077]
          frame False {
            n1370 = property on="X" class="DigNum (strict)"("Val(Sgnl)"=w2076) -> ()  [unwired: 2 in, 2 out]
          }
          frame True {
            n1371 = property on="Y" class="DigNum (strict)"("Val(Sgnl)"=w2077) -> ()  [unwired: 2 in, 2 out]
          }
        }
      }
      event "Fish": Value Change {
        n1372 = event-data() -> ()  [unwired: 1 in, 6 out]
        n1373 = local read "Fish"() -> (w2078:bool)
        n1374 = case shown="True" w2078 {
          frame False {
          }
          frame True {
            w2088 = 0.0 ("minimum value")
            w2089 = 10.0 ("maximum value")
            # "Grab offset in pulling\ndirection and add to \ndelta values"
            n1375 = call-poly <vilib>:"DAQmx Create Virtual Channel.vi"("maximum value"=w2089, "minimum value"=w2088, "physical channels"=tag "Dev1/ao0") -> ("task out"=w2093:refnum<k21>, "error out"=w2092:errorcluster)  [unwired: 11 in]
            n1376 = call-poly <vilib>:"DAQmx Create Virtual Channel.vi"("task in"=w2093, "maximum value"=w2089, "minimum value"=w2088, "physical channels"=tag "Dev1/ao1", "error in"=w2092) -> ("task out"=w2087:refnum<k21>, "error out"=w2086:errorcluster)  [unwired: 9 in]
            n1377 = node-c288(i64 1 ("Period")) -> (w2095:T13)  [unwired: 3 in]
            n1378 = timed-loop {
              timing: w2095 -> [_]
              timing-out: [_] -> w2094
              tunnel: w2087 -> [w2164]
              tunnel: w2086 -> [w2163]
              tunnel: [w2162] -> w2083
              tunnel: [w2161] -> w2082
              tunnel: [w2121] -> w2084
              tunnel: [w2122] -> w2081
              i -> [w2147]
              stop <- w2122 stop-if-true
              # "x direction"
              # "y direction"
              # "Send offset in direction\nof not-pulling to DAQ"
              n1379 = node-c288() -> ()  [unwired: 1 in, 1 out]
              n1380 = local read "Pulling direction"() -> (w2126:bool)
              n1381 = local read "Conv Y (nm/V)"() -> (w2128:dbl)
              n1382 = local read "Conv X (nm/V)"() -> (w2127:dbl)
              n1383 = local read "Fixed X"() -> (w2135:dbl)
              n1384 = local read "Fixed Y"() -> (w2134:dbl)
              n1385 = Select(t=w2134, s=w2126, f=w2135) -> (s? t:f=w2136:dbl)
              n1386 = Select(t=w2135, s=w2126, f=w2134) -> (s? t:f=w2133:dbl)
              n1387 = Select(t=w2128, s=w2126, f=w2127) -> (s? t:f=w2123:dbl)
              n1388 = Divide(x="Max fish\ndelta (nm)", y=w2123) -> (x/y=w2125:dbl)
              n1389 = Divide(x="Min fish\ndelta (nm)", y=w2123) -> (x/y=w2124:dbl)
              n1390 = Add(x=w2136, y=w2125) -> (x+y=w2138:dbl)
              n1391 = Subtract(x=w2125, y=w2124) -> (x-y=w2140:dbl)
              n1392 = Divide(x=w2140, y="Fish Speed (ms)") -> (x/y=w2141:dbl)
              n1393 = flat-sequence {
                tunnel: w2126 -> [w2184]
                tunnel: w2133 -> [w2183]
                tunnel: w2164 -> [w2182]
                tunnel: w2163 -> [w2181]
                tunnel: w2141 -> [w2180]
                tunnel: w2138 -> [w2179]
                tunnel: "Fish Speed (ms)" -> [w2174]
                tunnel: [w2178] -> w2160
                tunnel: [w2177] -> w2159
                tunnel: [w2176] -> w2158
                tunnel: [w2175] -> w2157
                tunnel: [w2168] -> w2146
                tunnel: [w2167] -> w2132
                tunnel: [w2166] -> w2129
                tunnel: [w2165] -> w2119
                tunnel: [w2237] -> w2156
                tunnel: w2160 -> [w2237]
                tunnel: [w2236] -> w2155
                tunnel: w2159 -> [w2236]
                tunnel: [w2235] -> w2154
                tunnel: w2158 -> [w2235]
                tunnel: [w2234] -> w2153
                tunnel: w2157 -> [w2234]
                tunnel: w2146 -> [w2233]
                tunnel: [w2233] -> w2145
                tunnel: w2132 -> [w2232]
                tunnel: [w2231] -> w2130
                tunnel: w2129 -> [w2231]
                tunnel: [w2230] -> w2120
                tunnel: w2119 -> [w2230]
                tunnel: w2156 -> [w2249]
                tunnel: w2155 -> [w2248]
                tunnel: w2154 -> [w2247]
                tunnel: w2153 -> [w2246]
                tunnel: w2143 -> [w2245]
                tunnel: [w2244] -> w2162
                tunnel: [w2243] -> w2161
                tunnel: w2145 -> [w2242]
                tunnel: [w2241] -> w2131
                tunnel: w2130 -> [w2240]
                tunnel: [w2239] -> w2118
                tunnel: w2120 -> [w2239]
                frame #0 {
                  n1394 = local read "Mean force (pN)"() -> (w2173:dbl)
                  n1395 = local read "Cutoff force (pN)"() -> (w2172:dbl)
                  n1396 = Less Or Equal?(x=w2173, y=w2172) -> (x <= y?=w2170:bool)
                  n1397 = And(x="Fish", y=w2170) -> (x .and. y?=w2171:bool)
                  n1398 = case shown="True" w2171 {
                    selector: w2171 -> [w2187 _]
                    tunnel: w2184 -> [w2190 w2207]
                    tunnel: w2183 -> [_ w2206]
                    tunnel: w2182 -> [w2192 w2205]
                    tunnel: w2181 -> [w2191 w2204]
                    tunnel: w2180 -> [w2189 w2203]
                    tunnel: w2179 -> [w2188 w2202]
                    tunnel: [w2192 w2201] -> w2178
                    tunnel: [w2191 w2200] -> w2177
                    tunnel: [w2190 w2199] -> w2176
                    tunnel: [w2188 w2198] -> w2166
                    tunnel: [w2189 w2197] -> w2175
                    tunnel: w2174 -> [_ w2196]
                    tunnel: [w2187 w2195] -> w2168
                    tunnel: [FALSE w2194] -> w2167
                    tunnel: [FALSE w2193] -> w2165
                    frame False {
                    }
                    frame True {
                      n1399 = while {
                        tunnel: w2207 -> [w2219]
                        tunnel: w2206 -> [w2218]
                        tunnel: w2205 -> [w2226]
                        tunnel: w2204 -> [w2225]
                        tunnel: w2203 -> [w2217]
                        tunnel: w2202 -> [w2223]
                        tunnel: [w2221] -> w2201
                        tunnel: [w2220] -> w2200
                        tunnel: [w2219] -> w2199
                        tunnel: [w2218] -> w2198
                        tunnel: [w2217] -> w2197
                        tunnel: w2196 -> [w2216]
                        tunnel: [w2209] -> w2195
                        tunnel: [w2209] -> w2194
                        tunnel: [w2208] -> w2193
                        i -> [w2215]
                        stop <- w2212 stop-if-true
                        # "top: x"
                        # "x direction"
                        # "y direction"
                        n1400 = Multiply(x=w2217, y=w2215) -> (x*y=w2224:dbl)
                        n1401 = local read "Cutoff force (pN)"() -> (w2210:dbl)
                        n1402 = local read "Mean force (pN)"() -> (w2211:dbl)
                        n1403 = Subtract(x=w2223, y=w2224) -> (x-y=w2222:dbl)
                        n1404 = Build Array(w2218, w2222) -> (w2229:dbl[])
                        n1405 = Build Array(w2222, w2218) -> (w2228:dbl[])
                        n1406 = Greater Or Equal?(x=w2215, y=w2216) -> (x >= y?=w2209:bool)
                        n1407 = Select(t=w2229, s=w2219, f=w2228) -> (s? t:f=w2227:dbl[])
                        n1408 = Greater?(x=w2211, y=w2210) -> (0:w2208:bool)
                        n1409 = local read "Fish"() -> (w2213:bool)
                        n1410 = Not(x=w2213) -> (.not. x?=w2214:bool)
                        n1411 = call-poly <vilib>:"DAQmx Write.vi"("task/channels in"=w2226, "data"=w2227, "error in"=w2225) -> ("task out"=w2221:refnum<k21>, "error out"=w2220:errorcluster)  [unwired: 10 in, 1 out]
                        n1412 = Compound Arithmetic op=OR(w2209, w2214, w2208) -> (w2212:bool)
                      }
                    }
                  }
                }
                frame #1 {
                  n1413 = case shown="True" w2232 {
                    frame False {
                    }
                    frame True {
                      n1414 = Wait (ms)(milliseconds to wait="Wait (ms)") -> ()  [unwired: 1 out]
                    }
                  }
                }
                frame #2 {
                  n1415 = case shown="True" w2242 {
                    tunnel: w2249 -> [w2252 w2261]
                    tunnel: w2248 -> [w2251 w2260]
                    tunnel: w2247 -> [_ w2259]
                    tunnel: w2246 -> [_ w2258]
                    tunnel: w2245 -> [_ w2257]
                    tunnel: [w2252 w2256] -> w2244
                    tunnel: [w2251 w2255] -> w2243
                    tunnel: [FALSE w2254] -> w2241
                    tunnel: w2240 -> [_ w2253]
                    frame False {
                    }
                    frame True {
                      n1416 = while {
                        tunnel: w2261 -> [w2293]
                        tunnel: w2260 -> [w2292]
                        tunnel: w2259 -> [w2264]
                        tunnel: w2258 -> [w2290]
                        tunnel: w2257 -> [w2289]
                        tunnel: [w2287] -> w2256
                        tunnel: [w2286] -> w2255
                        tunnel: [w2271] -> w2254
                        tunnel: w2253 -> [w2262]
                        i -> [w2278]
                        stop <- w2283 stop-if-true
                        # "y direction"
                        # "If tether formed,\nimmediately change\nto new delta."
                        n1417 = local read "Conv Y (nm/V)"() -> (w2265:dbl)
                        n1418 = local read "Conv X (nm/V)"() -> (w2263:dbl)
                        n1419 = local read "Fixed Y"() -> (w2272:dbl)
                        n1420 = local read "Fixed X"() -> (w2277:dbl)
                        n1421 = Select(t=w2265, s=w2264, f=w2263) -> (s? t:f=w2266:dbl)
                        n1422 = local read "Cutoff force (pN)"() -> (w2279:dbl)
                        n1423 = Divide(x="Delta after tether", y=w2266) -> (x/y=w2267:dbl)
                        n1424 = Multiply(x=w2290, y=w2278) -> (x*y=w2291:dbl)
                        n1425 = local read "Mean force (pN)"() -> (w2280:dbl)
                        n1426 = Add(x=w2289, y=w2291) -> (x+y=w2274:dbl)
                        n1427 = Select(t=w2272, s=w2264, f=w2277) -> (s? t:f=w2276:dbl)
                        n1428 = Greater?(x=w2280, y=w2279) -> (0:w2271:bool)
                        n1429 = Add(x=w2276, y=w2267) -> (x+y=w2275:dbl)
                        n1430 = Select(t=w2275, s=w2271, f=w2274) -> (s? t:f=w2273:dbl)
                        n1431 = local read "Fish Speed (ms)"() -> (w2285:i32)
                        n1432 = Build Array(w2262, w2273) -> (w2288:dbl[])
                        n1433 = Build Array(w2273, w2262) -> (w2269:dbl[])
                        n1434 = Select(t=w2288, s=w2264, f=w2269) -> (s? t:f=w2268:dbl[])
                        n1435 = case shown="True" w2271 {
                          tunnel: w2267 -> [_ _]
                          tunnel: w2268 -> [_ w2295]
                          frame False {
                          }
                          frame True {
                            n1436 = Array To Cluster(array=w2295) -> (cluster=w2294:cluster{"[0]":dbl, "[1]":dbl})
                            n1437 = property on="Trap position (V)" class="Clust (strict)"("Val(Sgnl)"=w2294) -> ()  [unwired: 2 in, 2 out]
                          }
                        }
                        n1438 = local read "Fish"() -> (w2282:bool)
                        n1439 = Greater Or Equal?(x=w2278, y=w2285) -> (x >= y?=w2284:bool)
                        n1440 = Not(x=w2282) -> (.not. x?=w2281:bool)
                        n1441 = call-poly <vilib>:"DAQmx Write.vi"("task/channels in"=w2293, "data"=w2268, "error in"=w2292) -> ("task out"=w2287:refnum<k21>, "error out"=w2286:errorcluster)  [unwired: 10 in, 1 out]
                        n1442 = Compound Arithmetic op=OR(w2284, w2281, w2271) -> (w2283:bool)
                      }
                    }
                  }
                }
              }
              n1443 = Add(x=w2136, y=w2124) -> (x+y=w2143:dbl)
              n1444 = Decrement(x="# attempts") -> (x-1=w2151:dbl)
              n1445 = Greater Or Equal?(x=w2147, y=w2151) -> (x >= y?=w2150:bool)
              n1446 = local read "Mean force (pN)"() -> (w2149:dbl)
              n1447 = Greater?(x=w2149, y="Cutoff force (pN)") -> (0:w2144:bool)
              n1448 = Compound Arithmetic op=OR(w2118, w2131, w2144, w2150) -> (w2122:bool)
              n1449 = Or(x=w2131, y=w2118) -> (x .or. y?=w2121:bool)
              "Tether" <- w2121
              n1450 = case shown="True" w2121 {
                frame False {
                }
                frame True {
                  n1451 = call <vilib>:"Beep.vi"() -> ()  [unwired: 12 in]
                }
              }
              n1452 = node-c288() -> ()  [unwired: 1 in, 1 out]
              "Attempt #" <- w2147
            }
            n1453 = node-c288(w2094) -> ()  [unwired: 1 out]
            n1454 = flat-sequence {
              tunnel: w2084 -> [w2102]
              tunnel: [w2102] -> w2080
              tunnel: w2083 -> [w2099]
              tunnel: w2082 -> [w2098]
              tunnel: w2081 -> [w2096]
              tunnel: w2080 -> [w2104]
              tunnel: [w2104] -> w2079
              tunnel: w2079 -> [w2106]
              frame #0 {
                w2101 = T24 1 items=["no dialog", "OK message", "continue or stop message", "OK message + warnings", "continue/stop + warnings"] ("type of dialog (OK msg:1)")
                n1455 = call <vilib>:"DAQmx Clear Task.vi"("task in"=w2099, "error in"=w2098) -> ("error out"=w2100:errorcluster)  [unwired: 13 in]
                n1456 = Not(x=w2096) -> (.not. x?=w2097:bool)
                n1457 = local write "Fish"(w2097) -> ()
                n1458 = call <vilib>:"Simple Error Handler.vi"("type of dialog (OK msg:1)"=w2101, "error in (no error)"=w2100) -> ()  [unwired: 3 in, 5 out]
              }
              frame #1 {
                n1459 = Wait (ms)(milliseconds to wait=u32 500) -> ()  [unwired: 1 out]
              }
              frame #2 {
                n1460 = And(x=w2106, y="Raster after\n tether?") -> (x .and. y?=w2107:bool)
                n1461 = case shown="True" w2107 {
                  selector: w2107 -> [_ w2108]
                  frame False {
                  }
                  frame True {
                    n1462 = stacked-sequence {
                      tunnel: w2108 -> [_ _ _ _ w2117]
                      frame #0 {
                        n1463 = local read "Raster set"() -> (w2112:i32)
                        n1464 = property on="Inject Sample" class="Bool (strict)"("Val(Sgnl)"=FALSE ("Value (Signaling)")) -> ()  [unwired: 2 in, 2 out]
                        n1465 = Replace Array Subset(array=i32[] [0], new element=w2112, index=0) -> (w2109:i32[])
                        n1466 = property on="Scan Parameters" class="Arr (strict)"("Index Values"=w2109) -> ()  [unwired: 2 in, 2 out]
                      }
                      frame #1 {
                        n1467 = Wait (ms)(milliseconds to wait=u32 500) -> ()  [unwired: 1 out]
                      }
                      frame #2 {
                        n1468 = property on="Load param" class="Bool (strict)"("Val(Sgnl)"=TRUE ("Value (Signaling)")) -> ()  [unwired: 2 in, 2 out]
                      }
                      frame #3 {
                        n1469 = Wait (ms)(milliseconds to wait=u32 500) -> ()  [unwired: 1 out]
                      }
                      frame #4 {
                        n1470 = property on="Raster scan" class="Bool (strict)"("Val(Sgnl)"=w2117) -> ()  [unwired: 2 in, 2 out]
                      }
                    }
                  }
                }
              }
            }
          }
        }
      }
      event "Load param": Value Change {
        n1471 = event-data() -> ()  [unwired: 1 in, 6 out]
        n1472 = property on="Scan Parameters" class="Arr (strict)"() -> ("Index Values"=w2311:u32[])  [unwired: 2 in, 2 out]
        n1473 = Index Array(array=w2311, index=0) -> (element=w2308:u32)
        n1474 = Index Array(array="Scan Parameters", index=w2308) -> (element=w2307:T27)
        n1475 = Unbundle(w2307) -> ("Scan range 1"=w2305:dbl, "Step size 1"=w2304:dbl, "Scan speed 1"=w2302:i32, "# scans 2"=w2303:i32)  [unwired: 1 out]
        n1476 = property on="# scans" class="DigNum (strict)"("Val(Sgnl)"=w2303) -> ()  [unwired: 2 in, 2 out]
        n1477 = property on="Scan range (nm)" class="DigNum (strict)"("Val(Sgnl)"=w2305) -> ()  [unwired: 2 in, 2 out]
        n1478 = property on="Step size 1" class="DigNum (strict)"("Val(Sgnl)"=w2304) -> ()  [unwired: 2 in, 2 out]
        n1479 = property on="Scan speed (nm/s)" class="DigNum (strict)"("Val(Sgnl)"=w2302) -> ()  [unwired: 2 in, 2 out]
        n1480 = local write "Load param"(FALSE ("Load param")) -> ()
      }
      event "# scans", "Scan range (nm)", "Step size (nm)", "Scan speed (nm/s)": Value Change {
        n1481 = event-data() -> ()  [unwired: 1 in, 6 out]
        n1482 = local read "Pulling direction"() -> (w2342:bool)
        n1483 = Reciprocal(x="Scan speed (nm/s)") -> (1/x=w2334:dbl)
        n1484 = local read "Conv Y (nm/V)"() -> (w2340:dbl)
        n1485 = local read "Conv X (nm/V)"() -> (w2341:dbl)
        n1486 = Multiply(x="Step size (nm)", y=w2334) -> (x*y=w2332:dbl)
        n1487 = Divide(x="Scan range (nm)", y="Step size (nm)") -> (x/y=w2339:dbl)
        n1488 = Absolute Value(x=w2339) -> (abs(x)=w2338:dbl)
        n1489 = Multiply(x=w2332, y=1000.0) -> (x*y=w2319:dbl)
        n1490 = Select(t=w2340, s=w2342, f=w2341) -> (s? t:f=w2330:dbl)
        n1491 = Multiply(x="# scans", y=2) -> (x*y=w2318:i32)
        n1492 = To Unsigned Quad Integer(1:w2338) -> (0:w2328:u64)
        "Scan steps (mirror)" <- w2328
        n1493 = Divide(x="Scan range (nm)", y=w2330) -> (x/y=→"Scan range (V)":dbl)
        n1494 = Multiply(x=w2328, y=w2319) -> (x*y=w2327:dbl)
        n1495 = Divide(x="Step size (nm)", y=w2330) -> (x/y=→"Scan increment (V)":dbl)
        n1496 = Round Toward +Infinity(x=w2319) -> (ceil(x): smallest int >= x=w2316:dbl)
        "Time per step (ms)" <- w2316
        n1497 = local read "Data update period (s/set)"() -> (w2322:dbl)
        n1498 = Multiply(x=w2318, y=w2327) -> (x*y=w2325:dbl)
        n1499 = Divide(x=w2325, y=1000.0) -> (x/y=w2323:dbl)
        "Total raster time (s)" <- w2323
        n1500 = local read "Data update period (s/set)"() -> (w2314:dbl)
        n1501 = Divide(x=w2323, y=w2322) -> (x/y=w2321:dbl)
        n1502 = Round Toward -Infinity(1:w2321) -> (0:→"N sets to be saved":dbl)
        n1503 = Multiply(x=w2314, y=1000.0) -> (x*y=w2312:dbl)
        n1504 = Less?(x=w2316, y=w2312) -> (x < y?=w2315:bool)
        n1505 = case shown="True" w2315 {
          selector: w2315 -> [_ w2343]
          frame False {
          }
          frame True {
            n1506 = call "Display Message to User"("Enable"=w2343) -> ()  [unwired: 9 in, 2 out]
          }
        }
      }
      event "Pulling direction": Value Change {
        n1507 = event-data() -> ()  [unwired: 1 in, 6 out]
        n1508 = local read "Pulling direction"() -> (w2349:bool)
        n1509 = local read "Conv Y (nm/V)"() -> (w2351:dbl)
        n1510 = local read "Conv X (nm/V)"() -> (w2350:dbl)
        n1511 = local read "Scan range (nm)"() -> (w2348:dbl)
        n1512 = Select(t=w2351, s=w2349, f=w2350) -> (s? t:f=w2345:dbl)
        n1513 = local read "Step size (nm)"() -> (w2346:dbl)
        n1514 = case shown="False" w2349 {
          frame False {
            n1515 = local read "Fixed Y"() -> (w2354:dbl)
            n1516 = local read "Trap delta (nm)"() -> (w2359:dbl)
            n1517 = local read "Conv X (nm/V)"() -> (w2358:dbl)
            n1518 = local read "Fixed X"() -> (w2356:dbl)
            n1519 = Divide(x=w2359, y=w2358) -> (x/y=w2357:dbl)
            n1520 = Add(x=w2357, y=w2356) -> (x+y=w2355:dbl)
            n1521 = Build Array(w2355, w2354) -> (w2353:dbl[])
            n1522 = Array To Cluster(array=w2353) -> (cluster=w2352:cluster{"[0]":dbl, "[1]":dbl})
            n1523 = property on="Trap position (V)" class="Clust (strict)"("Val(Sgnl)"=w2352) -> ()  [unwired: 2 in, 2 out]
          }
          frame True {
            n1524 = local read "Trap delta (nm)"() -> (w2367:dbl)
            n1525 = local read "Conv Y (nm/V)"() -> (w2366:dbl)
            n1526 = local read "Fixed X"() -> (w2362:dbl)
            n1527 = local read "Fixed Y"() -> (w2364:dbl)
            n1528 = Divide(x=w2367, y=w2366) -> (x/y=w2365:dbl)
            n1529 = Add(x=w2365, y=w2364) -> (x+y=w2363:dbl)
            n1530 = Build Array(w2362, w2363) -> (w2361:dbl[])
            n1531 = Array To Cluster(array=w2361) -> (cluster=w2360:cluster{"[0]":dbl, "[1]":dbl})
            n1532 = property on="Trap position (V)" class="Clust (strict)"("Val(Sgnl)"=w2360) -> ()  [unwired: 2 in, 2 out]
          }
        }
        n1533 = Divide(x=w2348, y=w2345) -> (x/y=w2347:dbl)
        n1534 = Divide(x=w2346, y=w2345) -> (x/y=w2344:dbl)
        n1535 = local write "Scan range (V)"(w2347) -> ()
        n1536 = local write "Scan increment (V)"(w2344) -> ()
      }
      event "Averaging Number": Value Change {
        n1537 = event-data() -> ()  [unwired: 1 in, 6 out]
        n1538 = local read "# Samples/channel (in)"() -> (w2371:i32)
        n1539 = local read "Averaging Number"() -> (w2369:i32)
        n1540 = Quotient & Remainder(x=w2371, y=w2369) -> (floor(x/y)=w2370:i32)  [unwired: 1 out]
        n1541 = Multiply(x=w2370, y=w2369) -> (x*y=w2368:i32)
        n1542 = local write "# Samples/channel (in)"(w2368) -> ()
      }
    }
    n1543 = node-c288() -> ()  [unwired: 1 in, 1 out]
  }
  n1544 = VISA Close(VISA resource name=w27) -> (error out=w105:errorcluster)  [unwired: 1 in]
  n1545 = call <vilib>:"Simple Error Handler.vi"("error in (no error)"=w105) -> ()  [unwired: 4 in, 5 out]
  n1546 = disable-structure shown="Enabled" {
    frame Disabled {
      n1547 = node-c288(2 ("Processor")) -> (w2377:T13)  [unwired: 3 in]
      n1548 = timed-loop "Pump Control" {
        timing: w2377 -> [_]
        timing-out: [_] -> w2376
        tunnel: refnum<visa-resource-name> "COM6" ("VISA resource name") -> [w2379]
        stop <- w2378 stop-if-true
        n1549 = node-c288() -> ()  [unwired: 1 in, 1 out]
        n1550 = event shown="[2] \"Stop\": Value Change" {
          selector: _ -> [_ _ _ _ _ _ _ _ _]
          dyn-events: _ -> [_ _ _ _ _ _ _ _ _]
          timeout: _ -> [_ _ _ _ _ _ _ _ _]
          tunnel: w2379 -> [w2387 w2483 _ w2559 w2687 w2830 w2875 w2933 w2992]
          tunnel: [_ _ w2558 _ _ _ _ _ _] -> w2378
          event "Flush Pump 1": Value Change {
            w2388 = "\r"
            n1551 = event-data() -> ()  [unwired: 1 in, 5 out]
            n1552 = call-poly "VISA Configure Serial Port"("VISA resource name"=w2387) -> ("VISA resource name out"=w2401:refnum<visa-resource-name>, "error out"=w2402:errorcluster)  [unwired: 13 in]
            n1553 = local read "Write Wait"() -> (w2380:i32)
            n1554 = Concatenate Strings("enter pump1", w2388) -> (w2389:string)
            n1555 = flat-sequence {
              tunnel: w2402 -> [w2421]
              tunnel: w2401 -> [w2423]
              tunnel: [w2422] -> w2418
              tunnel: [w2420] -> w2417
              tunnel: w2389 -> [w2419]
              tunnel: w2418 -> [w2426]
              tunnel: [w2426] -> w2416
              tunnel: w2417 -> [w2425]
              tunnel: [w2425] -> w2415
              tunnel: w2380 -> [w2424]
              tunnel: [w2431] -> w2414
              tunnel: w2394 -> [w2430]
              tunnel: [w2427] -> w2413
              tunnel: w2416 -> [w2429]
              tunnel: w2415 -> [w2428]
              tunnel: w2414 -> [w2434]
              tunnel: [w2434] -> w2412
              tunnel: [w2433] -> w2411
              tunnel: w2413 -> [w2433]
              tunnel: w2380 -> [w2432]
              tunnel: w2412 -> [w2439]
              tunnel: [w2438] -> w2410
              tunnel: w2397 -> [w2437]
              tunnel: w2411 -> [w2436]
              tunnel: [w2435] -> w2409
              tunnel: w2410 -> [w2442]
              tunnel: [w2442] -> w2408
              tunnel: [w2441] -> w2407
              tunnel: w2409 -> [w2441]
              tunnel: w2380 -> [w2440]
              tunnel: w2408 -> [w2447]
              tunnel: [w2446] -> w2406
              tunnel: w2400 -> [w2445]
              tunnel: w2407 -> [w2444]
              tunnel: [w2443] -> w2405
              tunnel: [w2450] -> w2404
              tunnel: w2406 -> [w2450]
              tunnel: [w2449] -> w2403
              tunnel: w2405 -> [w2449]
              tunnel: w2380 -> [w2448]
              tunnel: w2404 -> [w2455]
              tunnel: w2403 -> [w2452]
              tunnel: [w2454] -> w2383
              tunnel: [w2453] -> w2381
              tunnel: [w2460] -> w2384
              tunnel: w2383 -> [w2460]
              tunnel: [w2459] -> w2382
              tunnel: w2381 -> [w2459]
              tunnel: w2380 -> [w2458]
              tunnel: w2384 -> [w2462]
              tunnel: w2382 -> [w2461]
              frame #0 {
                n1556 = VISA Write(VISA resource name=w2423, write buffer=w2419, error in (no error)=w2421) -> (VISA resource name out=w2422:refnum<visa-resource-name>, error out=w2420:errorcluster)  [unwired: 1 out]
              }
              frame #1 {
                n1557 = Wait (ms)(milliseconds to wait=w2424) -> ()  [unwired: 1 out]
              }
              frame #2 {
                n1558 = VISA Write(VISA resource name=w2429, write buffer=w2430, error in (no error)=w2428) -> (VISA resource name out=w2431:refnum<visa-resource-name>, error out=w2427:errorcluster)  [unwired: 1 out]
              }
              frame #3 {
                n1559 = Wait (ms)(milliseconds to wait=w2432) -> ()  [unwired: 1 out]
              }
              frame #4 {
                n1560 = VISA Write(VISA resource name=w2439, write buffer=w2437, error in (no error)=w2436) -> (VISA resource name out=w2438:refnum<visa-resource-name>, error out=w2435:errorcluster)  [unwired: 1 out]
              }
              frame #5 {
                n1561 = Wait (ms)(milliseconds to wait=w2440) -> ()  [unwired: 1 out]
              }
              frame #6 {
                n1562 = VISA Write(VISA resource name=w2447, write buffer=w2445, error in (no error)=w2444) -> (VISA resource name out=w2446:refnum<visa-resource-name>, error out=w2443:errorcluster)  [unwired: 1 out]
              }
              frame #7 {
                n1563 = Wait (ms)(milliseconds to wait=w2448) -> ()  [unwired: 1 out]
              }
              frame #8 {
                n1564 = Concatenate Strings("start ", "\r") -> (w2451:string)
                n1565 = VISA Write(VISA resource name=w2455, write buffer=w2451, error in (no error)=w2452) -> (VISA resource name out=w2454:refnum<visa-resource-name>, error out=w2453:errorcluster)  [unwired: 1 out]
              }
              frame #9 {
                n1566 = Wait (ms)(milliseconds to wait=w2458) -> ()  [unwired: 1 out]
              }
              frame #10 {
                n1567 = local write "Flush Pump 1"(FALSE ("Flush Pump 1")) -> ()
                n1568 = Concatenate Strings("enter main ", "\r") -> (w2466:string)
                n1569 = VISA Write(VISA resource name=w2462, write buffer=w2466, error in (no error)=w2461) -> (VISA resource name out=w2465:refnum<visa-resource-name>, error out=w2464:errorcluster)  [unwired: 1 out]
                n1570 = VISA Close(VISA resource name=w2465, error in (no error)=w2464) -> ()  [unwired: 1 out]
              }
            }
            n1571 = Concatenate Strings("set units 4 ", w2388) -> (w2394:string)
            n1572 = Multiply(x="Flush\nRate (ul/min)", y=60) -> (x*y=w2392:dbl)
            n1573 = Number To Decimal String(number=w2392) -> (decimal integer string=w2395:string)  [unwired: 1 in]
            n1574 = Concatenate Strings("set rate ", w2395, w2388) -> (w2397:string)
            n1575 = Number To Decimal String(number="Flush\nVolume (ul)") -> (decimal integer string=w2399:string)  [unwired: 1 in]
            n1576 = Concatenate Strings("set volume ", w2399, w2388) -> (w2400:string)
          }
          event "Flush Pump 2": Value Change {
            w2474 = "\r"
            n1577 = event-data() -> ()  [unwired: 1 in, 5 out]
            n1578 = call-poly "VISA Configure Serial Port"("VISA resource name"=w2483) -> ("VISA resource name out"=w2494:refnum<visa-resource-name>, "error out"=w2495:errorcluster)  [unwired: 13 in]
            n1579 = local read "Write Wait"() -> (w2469:i32)
            n1580 = Concatenate Strings("enter pump2", w2474) -> (w2475:string)
            n1581 = flat-sequence {
              tunnel: w2495 -> [w2510]
              tunnel: w2494 -> [w2512]
              tunnel: [w2511] -> w2480
              tunnel: [w2509] -> w2478
              tunnel: w2475 -> [w2508]
              tunnel: w2480 -> [w2515]
              tunnel: [w2515] -> w2479
              tunnel: w2478 -> [w2514]
              tunnel: [w2514] -> w2477
              tunnel: w2469 -> [w2513]
              tunnel: [w2520] -> w2507
              tunnel: w2487 -> [w2519]
              tunnel: [w2516] -> w2506
              tunnel: w2479 -> [w2518]
              tunnel: w2477 -> [w2517]
              tunnel: w2507 -> [w2523]
              tunnel: [w2523] -> w2505
              tunnel: [w2522] -> w2504
              tunnel: w2506 -> [w2522]
              tunnel: w2469 -> [w2521]
              tunnel: w2505 -> [w2528]
              tunnel: [w2527] -> w2503
              tunnel: w2490 -> [w2526]
              tunnel: w2504 -> [w2525]
              tunnel: [w2524] -> w2502
              tunnel: w2503 -> [w2531]
              tunnel: [w2531] -> w2501
              tunnel: [w2530] -> w2500
              tunnel: w2502 -> [w2530]
              tunnel: w2469 -> [w2529]
              tunnel: w2501 -> [w2536]
              tunnel: [w2535] -> w2499
              tunnel: w2493 -> [w2534]
              tunnel: w2500 -> [w2533]
              tunnel: [w2532] -> w2498
              tunnel: [w2539] -> w2497
              tunnel: w2499 -> [w2539]
              tunnel: [w2538] -> w2496
              tunnel: w2498 -> [w2538]
              tunnel: w2469 -> [w2537]
              tunnel: w2497 -> [w2546]
              tunnel: w2496 -> [w2545]
              tunnel: [w2541] -> w2473
              tunnel: [w2540] -> w2471
              tunnel: w2473 -> [w2549]
              tunnel: [w2549] -> w2472
              tunnel: w2471 -> [w2548]
              tunnel: [w2548] -> w2470
              tunnel: w2469 -> [w2547]
              tunnel: w2472 -> [w2553]
              tunnel: w2470 -> [w2552]
              frame #0 {
                n1582 = VISA Write(VISA resource name=w2512, write buffer=w2508, error in (no error)=w2510) -> (VISA resource name out=w2511:refnum<visa-resource-name>, error out=w2509:errorcluster)  [unwired: 1 out]
              }
              frame #1 {
                n1583 = Wait (ms)(milliseconds to wait=w2513) -> ()  [unwired: 1 out]
              }
              frame #2 {
                n1584 = VISA Write(VISA resource name=w2518, write buffer=w2519, error in (no error)=w2517) -> (VISA resource name out=w2520:refnum<visa-resource-name>, error out=w2516:errorcluster)  [unwired: 1 out]
              }
              frame #3 {
                n1585 = Wait (ms)(milliseconds to wait=w2521) -> ()  [unwired: 1 out]
              }
              frame #4 {
                n1586 = VISA Write(VISA resource name=w2528, write buffer=w2526, error in (no error)=w2525) -> (VISA resource name out=w2527:refnum<visa-resource-name>, error out=w2524:errorcluster)  [unwired: 1 out]
              }
              frame #5 {
                n1587 = Wait (ms)(milliseconds to wait=w2529) -> ()  [unwired: 1 out]
              }
              frame #6 {
                n1588 = VISA Write(VISA resource name=w2536, write buffer=w2534, error in (no error)=w2533) -> (VISA resource name out=w2535:refnum<visa-resource-name>, error out=w2532:errorcluster)  [unwired: 1 out]
              }
              frame #7 {
                n1589 = Wait (ms)(milliseconds to wait=w2537) -> ()  [unwired: 1 out]
              }
              frame #8 {
                n1590 = Concatenate Strings("start ", "\r") -> (w2544:string)
                n1591 = VISA Write(VISA resource name=w2546, write buffer=w2544, error in (no error)=w2545) -> (VISA resource name out=w2541:refnum<visa-resource-name>, error out=w2540:errorcluster)  [unwired: 1 out]
              }
              frame #9 {
                n1592 = Wait (ms)(milliseconds to wait=w2547) -> ()  [unwired: 1 out]
              }
              frame #10 {
                n1593 = local write "Flush Pump 2"(FALSE ("Flush Pump 1")) -> ()
                n1594 = Concatenate Strings("enter main ", "\r") -> (w2554:string)
                n1595 = VISA Write(VISA resource name=w2553, write buffer=w2554, error in (no error)=w2552) -> (VISA resource name out=w2551:refnum<visa-resource-name>, error out=w2550:errorcluster)  [unwired: 1 out]
                n1596 = VISA Close(VISA resource name=w2551, error in (no error)=w2550) -> ()  [unwired: 1 out]
              }
            }
            n1597 = Concatenate Strings("set units 4 ", w2474) -> (w2487:string)
            n1598 = Multiply(x="Flush \nRate (ul/min)  2", y=60) -> (x*y=w2485:dbl)
            n1599 = Number To Decimal String(number=w2485) -> (decimal integer string=w2488:string)  [unwired: 1 in]
            n1600 = Concatenate Strings("set rate ", w2488, w2474) -> (w2490:string)
            n1601 = Number To Decimal String(number="Flush\nVolume (ul)  2") -> (decimal integer string=w2492:string)  [unwired: 1 in]
            n1602 = Concatenate Strings("set volume ", w2492, w2474) -> (w2493:string)
          }
          event "Stop": Value Change {
            n1603 = event-data() -> ()  [unwired: 1 in, 5 out]
            n1604 = local read "Stop"() -> (w2558:bool)
          }
          event "Inject Pump 2": Value Change {
            n1605 = event-data() -> ()  [unwired: 1 in, 5 out]
            n1606 = case shown="True" "Inject Pump 2" {
              tunnel: w2559 -> [w2562 w2604]
              frame False {
                n1607 = local read "Write Wait"() -> (w2561:i32)
                n1608 = call-poly "VISA Configure Serial Port"("VISA resource name"=w2562) -> ("VISA resource name out"=w2566:refnum<visa-resource-name>, "error out"=w2567:errorcluster)  [unwired: 13 in]
                n1609 = Concatenate Strings("enter pump2", "\r") -> (w2564:string)
                n1610 = flat-sequence {
                  tunnel: w2567 -> [w2578]
                  tunnel: w2566 -> [w2580]
                  tunnel: [w2579] -> w2575
                  tunnel: [w2577] -> w2574
                  tunnel: w2564 -> [w2576]
                  tunnel: w2575 -> [w2583]
                  tunnel: w2574 -> [w2582]
                  tunnel: [w2583] -> w2573
                  tunnel: [w2582] -> w2572
                  tunnel: w2561 -> [w2581]
                  tunnel: [w2587] -> w2571
                  tunnel: [w2586] -> w2570
                  tunnel: w2573 -> [w2585]
                  tunnel: w2572 -> [w2584]
                  tunnel: w2571 -> [w2593]
                  tunnel: [w2593] -> w2569
                  tunnel: w2570 -> [w2592]
                  tunnel: [w2592] -> w2568
                  tunnel: w2561 -> [w2591]
                  tunnel: w2569 -> [w2597]
                  tunnel: w2568 -> [w2596]
                  frame #0 {
                    n1611 = VISA Write(VISA resource name=w2580, write buffer=w2576, error in (no error)=w2578) -> (VISA resource name out=w2579:refnum<visa-resource-name>, error out=w2577:errorcluster)  [unwired: 1 out]
                  }
                  frame #1 {
                    n1612 = Wait (ms)(milliseconds to wait=w2581) -> ()  [unwired: 1 out]
                  }
                  frame #2 {
                    n1613 = Concatenate Strings("stop ", "\r") -> (w2590:string)
                    n1614 = VISA Write(VISA resource name=w2585, write buffer=w2590, error in (no error)=w2584) -> (VISA resource name out=w2587:refnum<visa-resource-name>, error out=w2586:errorcluster)  [unwired: 1 out]
                  }
                  frame #3 {
                    n1615 = Wait (ms)(milliseconds to wait=w2591) -> ()  [unwired: 1 out]
                  }
                  frame #4 {
                    n1616 = Concatenate Strings("enter main ", "\r") -> (w2598:string)
                    n1617 = VISA Write(VISA resource name=w2597, write buffer=w2598, error in (no error)=w2596) -> (VISA resource name out=w2595:refnum<visa-resource-name>, error out=w2594:errorcluster)  [unwired: 1 out]
                    n1618 = VISA Close(VISA resource name=w2595, error in (no error)=w2594) -> ()  [unwired: 1 out]
                  }
                }
              }
              frame True {
                w2617 = "\r"
                n1619 = call-poly "VISA Configure Serial Port"("VISA resource name"=w2604) -> ("VISA resource name out"=w2606:refnum<visa-resource-name>, "error out"=w2605:errorcluster)  [unwired: 13 in]
                n1620 = local read "Write Wait"() -> (w2601:i32)
                n1621 = Concatenate Strings("enter pump2", w2617) -> (w2616:string)
                n1622 = flat-sequence {
                  tunnel: w2605 -> [w2640]
                  tunnel: w2606 -> [w2642]
                  tunnel: [w2641] -> w2637
                  tunnel: [w2639] -> w2636
                  tunnel: w2616 -> [w2638]
                  tunnel: w2637 -> [w2645]
                  tunnel: [w2645] -> w2635
                  tunnel: w2636 -> [w2644]
                  tunnel: [w2644] -> w2634
                  tunnel: w2601 -> [w2643]
                  tunnel: [w2650] -> w2633
                  tunnel: w2613 -> [w2649]
                  tunnel: [w2646] -> w2632
                  tunnel: w2635 -> [w2648]
                  tunnel: w2634 -> [w2647]
                  tunnel: w2633 -> [w2653]
                  tunnel: [w2653] -> w2631
                  tunnel: [w2652] -> w2630
                  tunnel: w2632 -> [w2652]
                  tunnel: w2601 -> [w2651]
                  tunnel: w2631 -> [w2658]
                  tunnel: [w2657] -> w2629
                  tunnel: w2610 -> [w2656]
                  tunnel: w2630 -> [w2655]
                  tunnel: [w2654] -> w2628
                  tunnel: w2629 -> [w2661]
                  tunnel: [w2661] -> w2627
                  tunnel: [w2660] -> w2626
                  tunnel: w2628 -> [w2660]
                  tunnel: w2601 -> [w2659]
                  tunnel: w2627 -> [w2666]
                  tunnel: [w2665] -> w2625
                  tunnel: w2607 -> [w2664]
                  tunnel: w2626 -> [w2663]
                  tunnel: [w2662] -> w2624
                  tunnel: [w2669] -> w2623
                  tunnel: w2625 -> [w2669]
                  tunnel: [w2668] -> w2622
                  tunnel: w2624 -> [w2668]
                  tunnel: w2601 -> [w2667]
                  tunnel: w2623 -> [w2676]
                  tunnel: w2622 -> [w2675]
                  tunnel: [w2671] -> w2621
                  tunnel: [w2670] -> w2620
                  tunnel: w2621 -> [w2679]
                  tunnel: [w2679] -> w2619
                  tunnel: w2620 -> [w2678]
                  tunnel: [w2678] -> w2618
                  tunnel: w2601 -> [w2677]
                  tunnel: w2619 -> [w2683]
                  tunnel: w2618 -> [w2682]
                  frame #0 {
                    n1623 = VISA Write(VISA resource name=w2642, write buffer=w2638, error in (no error)=w2640) -> (VISA resource name out=w2641:refnum<visa-resource-name>, error out=w2639:errorcluster)  [unwired: 1 out]
                  }
                  frame #1 {
                    n1624 = Wait (ms)(milliseconds to wait=w2643) -> ()  [unwired: 1 out]
                  }
                  frame #2 {
                    n1625 = VISA Write(VISA resource name=w2648, write buffer=w2649, error in (no error)=w2647) -> (VISA resource name out=w2650:refnum<visa-resource-name>, error out=w2646:errorcluster)  [unwired: 1 out]
                  }
                  frame #3 {
                    n1626 = Wait (ms)(milliseconds to wait=w2651) -> ()  [unwired: 1 out]
                  }
                  frame #4 {
                    n1627 = VISA Write(VISA resource name=w2658, write buffer=w2656, error in (no error)=w2655) -> (VISA resource name out=w2657:refnum<visa-resource-name>, error out=w2654:errorcluster)  [unwired: 1 out]
                  }
                  frame #5 {
                    n1628 = Wait (ms)(milliseconds to wait=w2659) -> ()  [unwired: 1 out]
                  }
                  frame #6 {
                    n1629 = VISA Write(VISA resource name=w2666, write buffer=w2664, error in (no error)=w2663) -> (VISA resource name out=w2665:refnum<visa-resource-name>, error out=w2662:errorcluster)  [unwired: 1 out]
                  }
                  frame #7 {
                    n1630 = Wait (ms)(milliseconds to wait=w2667) -> ()  [unwired: 1 out]
                  }
                  frame #8 {
                    n1631 = Concatenate Strings("start ", "\r") -> (w2674:string)
                    n1632 = VISA Write(VISA resource name=w2676, write buffer=w2674, error in (no error)=w2675) -> (VISA resource name out=w2671:refnum<visa-resource-name>, error out=w2670:errorcluster)  [unwired: 1 out]
                  }
                  frame #9 {
                    n1633 = Wait (ms)(milliseconds to wait=w2677) -> ()  [unwired: 1 out]
                  }
                  frame #10 {
                    n1634 = Concatenate Strings("enter main ", "\r") -> (w2684:string)
                    n1635 = VISA Write(VISA resource name=w2683, write buffer=w2684, error in (no error)=w2682) -> (VISA resource name out=w2681:refnum<visa-resource-name>, error out=w2680:errorcluster)  [unwired: 1 out]
                    n1636 = VISA Close(VISA resource name=w2681, error in (no error)=w2680) -> ()  [unwired: 1 out]
                  }
                }
                n1637 = local read "Normal \nRate (ul/hr)  2"() -> (w2602:dbl)
                n1638 = Concatenate Strings("set units 4 ", w2617) -> (w2613:string)
                n1639 = local read "Normal \nVolume (ul) 2"() -> (w2603:dbl)
                n1640 = Number To Decimal String(number=w2602) -> (decimal integer string=w2612:string)  [unwired: 1 in]
                n1641 = Concatenate Strings("set rate ", w2612, w2617) -> (w2610:string)
                n1642 = Number To Decimal String(number=w2603) -> (decimal integer string=w2608:string)  [unwired: 1 in]
                n1643 = Concatenate Strings("set volume ", w2608, w2617) -> (w2607:string)
              }
            }
          }
          event "Inject Pump 1": Value Change {
            n1644 = event-data() -> ()  [unwired: 1 in, 5 out]
            n1645 = case shown="True" "Inject Pump 1" {
              tunnel: w2687 -> [w2690 w2732]
              frame False {
                n1646 = local read "Write Wait"() -> (w2689:i32)
                n1647 = call-poly "VISA Configure Serial Port"("VISA resource name"=w2690) -> ("VISA resource name out"=w2694:refnum<visa-resource-name>, "error out"=w2695:errorcluster)  [unwired: 13 in]
                n1648 = Concatenate Strings("enter pump1", "\r") -> (w2692:string)
                n1649 = flat-sequence {
                  tunnel: w2695 -> [w2706]
                  tunnel: w2694 -> [w2708]
                  tunnel: [w2707] -> w2703
                  tunnel: [w2705] -> w2702
                  tunnel: w2692 -> [w2704]
                  tunnel: w2703 -> [w2711]
                  tunnel: w2702 -> [w2710]
                  tunnel: [w2711] -> w2701
                  tunnel: [w2710] -> w2700
                  tunnel: w2689 -> [w2709]
                  tunnel: [w2715] -> w2699
                  tunnel: [w2714] -> w2698
                  tunnel: w2701 -> [w2713]
                  tunnel: w2700 -> [w2712]
                  tunnel: w2699 -> [w2721]
                  tunnel: [w2721] -> w2697
                  tunnel: w2698 -> [w2720]
                  tunnel: [w2720] -> w2696
                  tunnel: w2689 -> [w2719]
                  tunnel: w2697 -> [w2725]
                  tunnel: w2696 -> [w2724]
                  frame #0 {
                    n1650 = VISA Write(VISA resource name=w2708, write buffer=w2704, error in (no error)=w2706) -> (VISA resource name out=w2707:refnum<visa-resource-name>, error out=w2705:errorcluster)  [unwired: 1 out]
                  }
                  frame #1 {
                    n1651 = Wait (ms)(milliseconds to wait=w2709) -> ()  [unwired: 1 out]
                  }
                  frame #2 {
                    n1652 = Concatenate Strings("stop ", "\r") -> (w2718:string)
                    n1653 = VISA Write(VISA resource name=w2713, write buffer=w2718, error in (no error)=w2712) -> (VISA resource name out=w2715:refnum<visa-resource-name>, error out=w2714:errorcluster)  [unwired: 1 out]
                  }
                  frame #3 {
                    n1654 = Wait (ms)(milliseconds to wait=w2719) -> ()  [unwired: 1 out]
                  }
                  frame #4 {
                    n1655 = Concatenate Strings("enter main ", "\r") -> (w2726:string)
                    n1656 = VISA Write(VISA resource name=w2725, write buffer=w2726, error in (no error)=w2724) -> (VISA resource name out=w2723:refnum<visa-resource-name>, error out=w2722:errorcluster)  [unwired: 1 out]
                    n1657 = VISA Close(VISA resource name=w2723, error in (no error)=w2722) -> ()  [unwired: 1 out]
                  }
                }
              }
              frame True {
                w2745 = "\r"
                n1658 = call-poly "VISA Configure Serial Port"("VISA resource name"=w2732) -> ("VISA resource name out"=w2734:refnum<visa-resource-name>, "error out"=w2733:errorcluster)  [unwired: 13 in]
                n1659 = local read "Write Wait"() -> (w2729:i32)
                n1660 = flat-sequence {
                  tunnel: w2733 -> [w2768]
                  tunnel: w2734 -> [w2770]
                  tunnel: [w2769] -> w2765
                  tunnel: [w2767] -> w2764
                  tunnel: w2744 -> [w2766]
                  tunnel: w2765 -> [w2773]
                  tunnel: [w2773] -> w2763
                  tunnel: w2764 -> [w2772]
                  tunnel: [w2772] -> w2762
                  tunnel: w2729 -> [w2771]
                  tunnel: [w2778] -> w2761
                  tunnel: w2741 -> [w2777]
                  tunnel: [w2774] -> w2760
                  tunnel: w2763 -> [w2776]
                  tunnel: w2762 -> [w2775]
                  tunnel: w2761 -> [w2781]
                  tunnel: [w2781] -> w2759
                  tunnel: [w2780] -> w2758
                  tunnel: w2760 -> [w2780]
                  tunnel: w2729 -> [w2779]
                  tunnel: w2759 -> [w2786]
                  tunnel: [w2785] -> w2757
                  tunnel: w2738 -> [w2784]
                  tunnel: w2758 -> [w2783]
                  tunnel: [w2782] -> w2756
                  tunnel: w2757 -> [w2789]
                  tunnel: [w2789] -> w2755
                  tunnel: [w2788] -> w2754
                  tunnel: w2756 -> [w2788]
                  tunnel: w2729 -> [w2787]
                  tunnel: w2755 -> [w2794]
                  tunnel: [w2793] -> w2753
                  tunnel: w2735 -> [w2792]
                  tunnel: w2754 -> [w2791]
                  tunnel: [w2790] -> w2752
                  tunnel: [w2797] -> w2751
                  tunnel: w2753 -> [w2797]
                  tunnel: [w2796] -> w2750
                  tunnel: w2752 -> [w2796]
                  tunnel: w2729 -> [w2795]
                  tunnel: w2751 -> [w2804]
                  tunnel: w2750 -> [w2803]
                  tunnel: [w2799] -> w2749
                  tunnel: [w2798] -> w2748
                  tunnel: w2749 -> [w2807]
                  tunnel: [w2807] -> w2747
                  tunnel: w2748 -> [w2806]
                  tunnel: [w2806] -> w2746
                  tunnel: w2729 -> [w2805]
                  tunnel: w2747 -> [w2811]
                  tunnel: w2746 -> [w2810]
                  frame #0 {
                    n1661 = VISA Write(VISA resource name=w2770, write buffer=w2766, error in (no error)=w2768) -> (VISA resource name out=w2769:refnum<visa-resource-name>, error out=w2767:errorcluster)  [unwired: 1 out]
                  }
                  frame #1 {
                    n1662 = Wait (ms)(milliseconds to wait=w2771) -> ()  [unwired: 1 out]
                  }
                  frame #2 {
                    n1663 = VISA Write(VISA resource name=w2776, write buffer=w2777, error in (no error)=w2775) -> (VISA resource name out=w2778:refnum<visa-resource-name>, error out=w2774:errorcluster)  [unwired: 1 out]
                  }
                  frame #3 {
                    n1664 = Wait (ms)(milliseconds to wait=w2779) -> ()  [unwired: 1 out]
                  }
                  frame #4 {
                    n1665 = VISA Write(VISA resource name=w2786, write buffer=w2784, error in (no error)=w2783) -> (VISA resource name out=w2785:refnum<visa-resource-name>, error out=w2782:errorcluster)  [unwired: 1 out]
                  }
                  frame #5 {
                    n1666 = Wait (ms)(milliseconds to wait=w2787) -> ()  [unwired: 1 out]
                  }
                  frame #6 {
                    n1667 = VISA Write(VISA resource name=w2794, write buffer=w2792, error in (no error)=w2791) -> (VISA resource name out=w2793:refnum<visa-resource-name>, error out=w2790:errorcluster)  [unwired: 1 out]
                  }
                  frame #7 {
                    n1668 = Wait (ms)(milliseconds to wait=w2795) -> ()  [unwired: 1 out]
                  }
                  frame #8 {
                    n1669 = Concatenate Strings("start ", "\r") -> (w2802:string)
                    n1670 = VISA Write(VISA resource name=w2804, write buffer=w2802, error in (no error)=w2803) -> (VISA resource name out=w2799:refnum<visa-resource-name>, error out=w2798:errorcluster)  [unwired: 1 out]
                  }
                  frame #9 {
                    n1671 = Wait (ms)(milliseconds to wait=w2805) -> ()  [unwired: 1 out]
                  }
                  frame #10 {
                    n1672 = Concatenate Strings("enter main ", "\r") -> (w2812:string)
                    n1673 = VISA Write(VISA resource name=w2811, write buffer=w2812, error in (no error)=w2810) -> (VISA resource name out=w2809:refnum<visa-resource-name>, error out=w2808:errorcluster)  [unwired: 1 out]
                    n1674 = VISA Close(VISA resource name=w2809, error in (no error)=w2808) -> ()  [unwired: 1 out]
                  }
                }
                n1675 = Concatenate Strings("enter pump1", w2745) -> (w2744:string)
                n1676 = local read "Normal \nRate (ul/hr)"() -> (w2730:dbl)
                n1677 = Concatenate Strings("set units 4 ", w2745) -> (w2741:string)
                n1678 = local read "Normal \nVolume (ul)"() -> (w2731:dbl)
                n1679 = Number To Decimal String(number=w2730) -> (decimal integer string=w2740:string)  [unwired: 1 in]
                n1680 = Concatenate Strings("set rate ", w2740, w2745) -> (w2738:string)
                n1681 = Number To Decimal String(number=w2731) -> (decimal integer string=w2736:string)  [unwired: 1 in]
                n1682 = Concatenate Strings("set volume ", w2736, w2745) -> (w2735:string)
              }
            }
          }
          event "Normal \nVolume (ul)": Value Change {
            n1683 = event-data() -> ()  [unwired: 1 in, 5 out]
            n1684 = call-poly "VISA Configure Serial Port"("VISA resource name"=w2830) -> ("VISA resource name out"=w2832:refnum<visa-resource-name>, "error out"=w2831:errorcluster)  [unwired: 13 in]
            n1685 = local read "Write Wait"() -> (w2815:i32)
            n1686 = Concatenate Strings("enter pump1", "\r") -> (w2834:string)
            n1687 = flat-sequence {
              tunnel: w2831 -> [w2844]
              tunnel: w2832 -> [w2846]
              tunnel: [w2845] -> w2824
              tunnel: [w2843] -> w2823
              tunnel: w2834 -> [w2842]
              tunnel: w2824 -> [w2849]
              tunnel: [w2849] -> w2822
              tunnel: w2823 -> [w2848]
              tunnel: [w2848] -> w2820
              tunnel: w2815 -> [w2847]
              tunnel: w2822 -> [w2853]
              tunnel: [w2854] -> w2821
              tunnel: w2820 -> [w2852]
              tunnel: [w2851] -> w2819
              tunnel: w2816 -> [w2850]
              tunnel: w2821 -> [w2857]
              tunnel: w2819 -> [w2856]
              tunnel: [w2857] -> w2841
              tunnel: [w2856] -> w2840
              tunnel: w2815 -> [w2855]
              tunnel: [w2862] -> w2839
              tunnel: [w2861] -> w2838
              tunnel: w2841 -> [w2860]
              tunnel: w2840 -> [w2859]
              tunnel: w2825 -> [w2858]
              tunnel: w2839 -> [w2865]
              tunnel: [w2865] -> w2837
              tunnel: w2838 -> [w2864]
              tunnel: [w2864] -> w2836
              tunnel: w2815 -> [w2863]
              tunnel: w2837 -> [w2869]
              tunnel: w2836 -> [w2868]
              frame #0 {
                n1688 = VISA Write(VISA resource name=w2846, write buffer=w2842, error in (no error)=w2844) -> (VISA resource name out=w2845:refnum<visa-resource-name>, error out=w2843:errorcluster)  [unwired: 1 out]
              }
              frame #1 {
                n1689 = Wait (ms)(milliseconds to wait=w2847) -> ()  [unwired: 1 out]
              }
              frame #2 {
                n1690 = VISA Write(VISA resource name=w2853, write buffer=w2850, error in (no error)=w2852) -> (VISA resource name out=w2854:refnum<visa-resource-name>, error out=w2851:errorcluster)  [unwired: 1 out]
              }
              frame #3 {
                n1691 = Wait (ms)(milliseconds to wait=w2855) -> ()  [unwired: 1 out]
              }
              frame #4 {
                n1692 = VISA Write(VISA resource name=w2860, write buffer=w2858, error in (no error)=w2859) -> (VISA resource name out=w2862:refnum<visa-resource-name>, error out=w2861:errorcluster)  [unwired: 1 out]
              }
              frame #5 {
                n1693 = Wait (ms)(milliseconds to wait=w2863) -> ()  [unwired: 1 out]
              }
              frame #6 {
                n1694 = Concatenate Strings("enter main ", "\r") -> (w2870:string)
                n1695 = VISA Write(VISA resource name=w2869, write buffer=w2870, error in (no error)=w2868) -> (VISA resource name out=w2867:refnum<visa-resource-name>, error out=w2866:errorcluster)  [unwired: 1 out]
                n1696 = VISA Close(VISA resource name=w2867, error in (no error)=w2866) -> ()  [unwired: 1 out]
              }
            }
            n1697 = Concatenate Strings("set units 4", "\r") -> (w2816:string)
            n1698 = Number To Decimal String(number="Normal \nVolume (ul)") -> (decimal integer string=w2827:string)  [unwired: 1 in]
            n1699 = Concatenate Strings("set volume", w2827, "\r") -> (w2825:string)
          }
          event "Normal \nRate (ul/hr)": Value Change {
            n1700 = event-data() -> ()  [unwired: 1 in, 5 out]
            n1701 = call-poly "VISA Configure Serial Port"("VISA resource name"=w2875) -> ("VISA resource name out"=w2883:refnum<visa-resource-name>, "error out"=w2882:errorcluster)  [unwired: 13 in]
            n1702 = local read "Write Wait"() -> (w2873:i32)
            n1703 = Concatenate Strings("enter pump1", "\r") -> (w2885:string)
            n1704 = flat-sequence {
              tunnel: w2882 -> [w2902]
              tunnel: w2883 -> [w2904]
              tunnel: [w2903] -> w2898
              tunnel: [w2901] -> w2897
              tunnel: w2885 -> [w2900]
              tunnel: w2898 -> [w2907]
              tunnel: [w2907] -> w2896
              tunnel: w2897 -> [w2906]
              tunnel: [w2906] -> w2895
              tunnel: w2873 -> [w2905]
              tunnel: w2896 -> [w2911]
              tunnel: [w2912] -> w2894
              tunnel: w2895 -> [w2910]
              tunnel: [w2909] -> w2893
              tunnel: w2876 -> [w2908]
              tunnel: w2894 -> [w2915]
              tunnel: w2893 -> [w2914]
              tunnel: [w2915] -> w2892
              tunnel: [w2914] -> w2891
              tunnel: w2873 -> [w2913]
              tunnel: [w2920] -> w2890
              tunnel: [w2919] -> w2889
              tunnel: w2892 -> [w2918]
              tunnel: w2891 -> [w2917]
              tunnel: w2879 -> [w2916]
              tunnel: w2890 -> [w2923]
              tunnel: [w2923] -> w2888
              tunnel: w2889 -> [w2922]
              tunnel: [w2922] -> w2887
              tunnel: w2873 -> [w2921]
              tunnel: w2888 -> [w2927]
              tunnel: w2887 -> [w2926]
              frame #0 {
                n1705 = VISA Write(VISA resource name=w2904, write buffer=w2900, error in (no error)=w2902) -> (VISA resource name out=w2903:refnum<visa-resource-name>, error out=w2901:errorcluster)  [unwired: 1 out]
              }
              frame #1 {
                n1706 = Wait (ms)(milliseconds to wait=w2905) -> ()  [unwired: 1 out]
              }
              frame #2 {
                n1707 = VISA Write(VISA resource name=w2911, write buffer=w2908, error in (no error)=w2910) -> (VISA resource name out=w2912:refnum<visa-resource-name>, error out=w2909:errorcluster)  [unwired: 1 out]
              }
              frame #3 {
                n1708 = Wait (ms)(milliseconds to wait=w2913) -> ()  [unwired: 1 out]
              }
              frame #4 {
                n1709 = VISA Write(VISA resource name=w2918, write buffer=w2916, error in (no error)=w2917) -> (VISA resource name out=w2920:refnum<visa-resource-name>, error out=w2919:errorcluster)  [unwired: 1 out]
              }
              frame #5 {
                n1710 = Wait (ms)(milliseconds to wait=w2921) -> ()  [unwired: 1 out]
              }
              frame #6 {
                n1711 = Concatenate Strings("enter main ", "\r") -> (w2928:string)
                n1712 = VISA Write(VISA resource name=w2927, write buffer=w2928, error in (no error)=w2926) -> (VISA resource name out=w2925:refnum<visa-resource-name>, error out=w2924:errorcluster)  [unwired: 1 out]
                n1713 = VISA Close(VISA resource name=w2925, error in (no error)=w2924) -> ()  [unwired: 1 out]
              }
            }
            n1714 = Concatenate Strings("set units 4", "\r") -> (w2876:string)
            n1715 = Number To Decimal String(number="Normal \nRate (ul/hr)") -> (decimal integer string=w2874:string)  [unwired: 1 in]
            n1716 = Concatenate Strings("set rate", w2874, "\r") -> (w2879:string)
          }
          event "Normal \nRate (ul/hr)  2": Value Change {
            n1717 = event-data() -> ()  [unwired: 1 in, 5 out]
            n1718 = call-poly "VISA Configure Serial Port"("VISA resource name"=w2933) -> ("VISA resource name out"=w2941:refnum<visa-resource-name>, "error out"=w2940:errorcluster)  [unwired: 13 in]
            n1719 = local read "Write Wait"() -> (w2931:i32)
            n1720 = Concatenate Strings("enter pump2", "\r") -> (w2943:string)
            n1721 = flat-sequence {
              tunnel: w2940 -> [w2960]
              tunnel: w2941 -> [w2962]
              tunnel: [w2961] -> w2956
              tunnel: [w2959] -> w2955
              tunnel: w2943 -> [w2958]
              tunnel: w2956 -> [w2965]
              tunnel: [w2965] -> w2954
              tunnel: w2955 -> [w2964]
              tunnel: [w2964] -> w2953
              tunnel: w2931 -> [w2963]
              tunnel: w2954 -> [w2969]
              tunnel: [w2970] -> w2952
              tunnel: w2953 -> [w2968]
              tunnel: [w2967] -> w2951
              tunnel: w2934 -> [w2966]
              tunnel: w2952 -> [w2973]
              tunnel: w2951 -> [w2972]
              tunnel: [w2973] -> w2950
              tunnel: [w2972] -> w2949
              tunnel: w2931 -> [w2971]
              tunnel: [w2978] -> w2948
              tunnel: [w2977] -> w2947
              tunnel: w2950 -> [w2976]
              tunnel: w2949 -> [w2975]
              tunnel: w2937 -> [w2974]
              tunnel: w2948 -> [w2981]
              tunnel: [w2981] -> w2946
              tunnel: w2947 -> [w2980]
              tunnel: [w2980] -> w2945
              tunnel: w2931 -> [w2979]
              tunnel: w2946 -> [w2985]
              tunnel: w2945 -> [w2984]
              frame #0 {
                n1722 = VISA Write(VISA resource name=w2962, write buffer=w2958, error in (no error)=w2960) -> (VISA resource name out=w2961:refnum<visa-resource-name>, error out=w2959:errorcluster)  [unwired: 1 out]
              }
              frame #1 {
                n1723 = Wait (ms)(milliseconds to wait=w2963) -> ()  [unwired: 1 out]
              }
              frame #2 {
                n1724 = VISA Write(VISA resource name=w2969, write buffer=w2966, error in (no error)=w2968) -> (VISA resource name out=w2970:refnum<visa-resource-name>, error out=w2967:errorcluster)  [unwired: 1 out]
              }
              frame #3 {
                n1725 = Wait (ms)(milliseconds to wait=w2971) -> ()  [unwired: 1 out]
              }
              frame #4 {
                n1726 = VISA Write(VISA resource name=w2976, write buffer=w2974, error in (no error)=w2975) -> (VISA resource name out=w2978:refnum<visa-resource-name>, error out=w2977:errorcluster)  [unwired: 1 out]
              }
              frame #5 {
                n1727 = Wait (ms)(milliseconds to wait=w2979) -> ()  [unwired: 1 out]
              }
              frame #6 {
                n1728 = Concatenate Strings("enter main ", "\r") -> (w2986:string)
                n1729 = VISA Write(VISA resource name=w2985, write buffer=w2986, error in (no error)=w2984) -> (VISA resource name out=w2983:refnum<visa-resource-name>, error out=w2982:errorcluster)  [unwired: 1 out]
                n1730 = VISA Close(VISA resource name=w2983, error in (no error)=w2982) -> ()  [unwired: 1 out]
              }
            }
            n1731 = Concatenate Strings("set units 4", "\r") -> (w2934:string)
            n1732 = Number To Decimal String(number="Normal \nRate (ul/hr)  2") -> (decimal integer string=w2932:string)  [unwired: 1 in]
            n1733 = Concatenate Strings("set rate", w2932, "\r") -> (w2937:string)
          }
          event "Normal \nVolume (ul) 2": Value Change {
            n1734 = event-data() -> ()  [unwired: 1 in, 5 out]
            n1735 = call-poly "VISA Configure Serial Port"("VISA resource name"=w2992) -> ("VISA resource name out"=w2996:refnum<visa-resource-name>, "error out"=w2997:errorcluster)  [unwired: 13 in]
            n1736 = local read "Write Wait"() -> (w2989:i32)
            n1737 = Concatenate Strings("enter pump2", "\r") -> (w2994:string)
            n1738 = flat-sequence {
              tunnel: w2997 -> [w3018]
              tunnel: w2996 -> [w3020]
              tunnel: [w3019] -> w3015
              tunnel: [w3017] -> w3014
              tunnel: w2994 -> [w3016]
              tunnel: w3015 -> [w3023]
              tunnel: [w3023] -> w3013
              tunnel: w3014 -> [w3022]
              tunnel: [w3022] -> w3012
              tunnel: w2989 -> [w3021]
              tunnel: w3013 -> [w3027]
              tunnel: [w3028] -> w3011
              tunnel: w3012 -> [w3026]
              tunnel: [w3025] -> w3010
              tunnel: w3003 -> [w3024]
              tunnel: w3011 -> [w3031]
              tunnel: w3010 -> [w3030]
              tunnel: [w3031] -> w3009
              tunnel: [w3030] -> w3008
              tunnel: w2989 -> [w3029]
              tunnel: [w3036] -> w3007
              tunnel: [w3035] -> w3006
              tunnel: w3009 -> [w3034]
              tunnel: w3008 -> [w3033]
              tunnel: w3000 -> [w3032]
              tunnel: w3007 -> [w3039]
              tunnel: [w3039] -> w3005
              tunnel: w3006 -> [w3038]
              tunnel: [w3038] -> w3004
              tunnel: w2989 -> [w3037]
              tunnel: w3005 -> [w3043]
              tunnel: w3004 -> [w3042]
              frame #0 {
                n1739 = VISA Write(VISA resource name=w3020, write buffer=w3016, error in (no error)=w3018) -> (VISA resource name out=w3019:refnum<visa-resource-name>, error out=w3017:errorcluster)  [unwired: 1 out]
              }
              frame #1 {
                n1740 = Wait (ms)(milliseconds to wait=w3021) -> ()  [unwired: 1 out]
              }
              frame #2 {
                n1741 = VISA Write(VISA resource name=w3027, write buffer=w3024, error in (no error)=w3026) -> (VISA resource name out=w3028:refnum<visa-resource-name>, error out=w3025:errorcluster)  [unwired: 1 out]
              }
              frame #3 {
                n1742 = Wait (ms)(milliseconds to wait=w3029) -> ()  [unwired: 1 out]
              }
              frame #4 {
                n1743 = VISA Write(VISA resource name=w3034, write buffer=w3032, error in (no error)=w3033) -> (VISA resource name out=w3036:refnum<visa-resource-name>, error out=w3035:errorcluster)  [unwired: 1 out]
              }
              frame #5 {
                n1744 = Wait (ms)(milliseconds to wait=w3037) -> ()  [unwired: 1 out]
              }
              frame #6 {
                n1745 = Concatenate Strings("enter main ", "\r") -> (w3044:string)
                n1746 = VISA Write(VISA resource name=w3043, write buffer=w3044, error in (no error)=w3042) -> (VISA resource name out=w3041:refnum<visa-resource-name>, error out=w3040:errorcluster)  [unwired: 1 out]
                n1747 = VISA Close(VISA resource name=w3041, error in (no error)=w3040) -> ()  [unwired: 1 out]
              }
            }
            n1748 = Concatenate Strings("set units 4", "\r") -> (w3003:string)
            n1749 = Number To Decimal String(number="Normal \nVolume (ul) 2") -> (decimal integer string=w2990:string)  [unwired: 1 in]
            n1750 = Concatenate Strings("set volume", w2990, "\r") -> (w3000:string)
          }
        }
        n1751 = node-c288() -> ()  [unwired: 1 in, 1 out]
      }
      n1752 = node-c288(w2376) -> ()  [unwired: 1 out]
    }
    frame Enabled {
      n1753 = node-c288(2 ("Processor")) -> (w3056:T13)  [unwired: 3 in]
      n1754 = timed-loop "Pump Control" {
        timing: w3056 -> [_]
        timing-out: [_] -> w3055
        tunnel: refnum<visa-resource-name> "COM4" ("VISA resource name") -> [w3058]
        stop <- w3057 stop-if-true
        n1755 = node-c288() -> ()  [unwired: 1 in, 1 out]
        n1756 = event shown="[2] \"Inject Sample\": Value Change" {
          selector: _ -> [_ _ _ _ _]
          dyn-events: _ -> [_ _ _ _ _]
          timeout: _ -> [_ _ _ _ _]
          tunnel: w3058 -> [w3064 _ w3138 w3171 w3176]
          tunnel: [_ w3136 _ _ _] -> w3057
          event "Flush Sample": Value Change {
            n1757 = event-data() -> ()  [unwired: 1 in, 5 out]
            n1758 = local read "Write Wait"() -> (w3078:i32)
            n1759 = flat-sequence {
              tunnel: [w3102] -> w3098
              tunnel: [w3101] -> w3097
              tunnel: "CLD" -> [w3100]
              tunnel: w3064 -> [w3099]
              tunnel: w3098 -> [w3105]
              tunnel: [w3105] -> w3096
              tunnel: w3097 -> [w3104]
              tunnel: [w3104] -> w3095
              tunnel: w3078 -> [w3103]
              tunnel: [w3110] -> w3094
              tunnel: [w3107] -> w3093
              tunnel: w3096 -> [w3109]
              tunnel: w3095 -> [w3108]
              tunnel: "MODVOL" -> [w3106]
              tunnel: w3094 -> [w3113]
              tunnel: [w3113] -> w3092
              tunnel: [w3112] -> w3091
              tunnel: w3093 -> [w3112]
              tunnel: w3078 -> [w3111]
              tunnel: w3092 -> [w3118]
              tunnel: [w3117] -> w3090
              tunnel: w3080 -> [w3116]
              tunnel: w3091 -> [w3115]
              tunnel: [w3114] -> w3089
              tunnel: w3090 -> [w3121]
              tunnel: [w3121] -> w3088
              tunnel: [w3120] -> w3087
              tunnel: w3089 -> [w3120]
              tunnel: w3078 -> [w3119]
              tunnel: w3088 -> [w3126]
              tunnel: [w3125] -> w3086
              tunnel: w3082 -> [w3124]
              tunnel: w3087 -> [w3123]
              tunnel: [w3122] -> w3085
              tunnel: [w3129] -> w3083
              tunnel: w3086 -> [w3129]
              tunnel: [w3128] -> w3084
              tunnel: w3085 -> [w3128]
              tunnel: w3078 -> [w3127]
              tunnel: w3084 -> [w3134]
              tunnel: w3083 -> [w3135]
              tunnel: [w3133] -> w3073
              tunnel: "RUN " -> [w3132]
              frame #0 {
                n1760 = call "Write to pump 2.vi"("String to write"=w3100, "VISA resource name"=w3099) -> ("error out"=w3101:errorcluster, "VISA resource name out"=w3102:refnum<visa-resource-name>)  [unwired: 8 in]
              }
              frame #1 {
                n1761 = Wait (ms)(milliseconds to wait=w3103) -> ()  [unwired: 1 out]
              }
              frame #2 {
                n1762 = call "Write to pump 2.vi"("error in (no error)"=w3108, "String to write"=w3106, "VISA resource name"=w3109) -> ("error out"=w3107:errorcluster, "VISA resource name out"=w3110:refnum<visa-resource-name>)  [unwired: 7 in]
              }
              frame #3 {
                n1763 = Wait (ms)(milliseconds to wait=w3111) -> ()  [unwired: 1 out]
              }
              frame #4 {
                n1764 = call "Write to pump 2.vi"("error in (no error)"=w3115, "String to write"=w3116, "VISA resource name"=w3118) -> ("error out"=w3114:errorcluster, "VISA resource name out"=w3117:refnum<visa-resource-name>)  [unwired: 7 in]
              }
              frame #5 {
                n1765 = Wait (ms)(milliseconds to wait=w3119) -> ()  [unwired: 1 out]
              }
              frame #6 {
                n1766 = call "Write to pump 2.vi"("error in (no error)"=w3123, "String to write"=w3124, "VISA resource name"=w3126) -> ("error out"=w3122:errorcluster, "VISA resource name out"=w3125:refnum<visa-resource-name>)  [unwired: 7 in]
              }
              frame #7 {
                n1767 = Wait (ms)(milliseconds to wait=w3127) -> ()  [unwired: 1 out]
              }
              frame #8 {
                w3131 = TRUE ("Inject Pump 3")
                n1768 = Tick Count (ms)() -> (millisecond timer value=→"Flush Sample Start Time":u32)
                n1769 = call "Write to pump 2.vi"("error in (no error)"=w3134, "String to write"=w3132, "VISA resource name"=w3135) -> ("error out"=w3133:errorcluster)  [unwired: 7 in, 1 out]
                n1770 = local write "Inject Sample"(w3131) -> ()
                "Flushing Sample" <- w3131
              }
            }
            n1771 = Number To Fractional String(number="Flush \nRate (ul/min)  3") -> (F-format string=w3066:string)  [unwired: 3 in]
            n1772 = String Subset(string=w3066, length (rest)=6 ("length (rest)")) -> (substring=w3065:string)  [unwired: 1 in]
            n1773 = Concatenate Strings("RAT", w3065, "UM") -> (w3080:string)
            n1774 = Divide(x="Flush\nVolume (ul)  3", y=1000.0) -> (x/y=w3071:dbl)
            n1775 = Number To Fractional String(number=w3071) -> (F-format string=w3070:string)  [unwired: 3 in]
            n1776 = Divide(x="Flush\nVolume (ul)  3", y="Flush \nRate (ul/min)  3") -> (x/y=w3061:dbl)
            n1777 = Multiply(x=w3061, y=60.0) -> (x*y=→"Sample flush time (s)":dbl)
            n1778 = String Subset(string=w3070, length (rest)=6 ("length (rest)")) -> (substring=w3069:string)  [unwired: 1 in]
            n1779 = Concatenate Strings("TGT", w3069) -> (w3082:string)
            "error out" <- w3073
          }
          event "Stop": Value Change {
            n1780 = event-data() -> ()  [unwired: 1 in, 5 out]
            n1781 = local read "Stop"() -> (w3136:bool)
          }
          event "Inject Sample": Value Change {
            n1782 = event-data() -> ()  [unwired: 1 in, 5 out]
            n1783 = case shown="True" "Inject Sample" {
              tunnel: w3138 -> [w3140 w3144]
              frame False {
                n1784 = call "Write to pump 2.vi"("String to write"="STP", "VISA resource name"=w3140) -> ()  [unwired: 8 in, 2 out]
              }
              frame True {
                n1785 = local read "Normal \nRate (ul/hr)  3"() -> (w3145:dbl)
                n1786 = Number To Fractional String(number=w3145) -> (F-format string=w3148:string)  [unwired: 3 in]
                n1787 = String Subset(string=w3148, length (rest)=6 ("length (rest)")) -> (substring=w3146:string)  [unwired: 1 in]
                n1788 = flat-sequence {
                  tunnel: w3144 -> [w3162]
                  tunnel: [w3161] -> w3143
                  tunnel: [w3160] -> w3142
                  tunnel: w3141 -> [w3159]
                  tunnel: "RUN " -> [w3165]
                  tunnel: w3143 -> [w3164]
                  tunnel: w3142 -> [w3163]
                  frame #0 {
                    n1789 = call "Write to pump 2.vi"("String to write"=w3159, "VISA resource name"=w3162) -> ("error out"=w3160:errorcluster, "VISA resource name out"=w3161:refnum<visa-resource-name>)  [unwired: 8 in]
                  }
                  frame #1 {
                    n1790 = call "Write to pump 2.vi"("error in (no error)"=w3163, "String to write"=w3165, "VISA resource name"=w3164) -> ()  [unwired: 7 in, 2 out]
                  }
                }
                n1791 = Concatenate Strings("RAT", w3146, "UH" ("string")) -> ()  [unwired: 1 out]
                n1792 = local read "Normal \nVolume (ul) 3"() -> (w3154:dbl)
                n1793 = Divide(x=w3154, y=1000.0) -> (x/y=w3149:dbl)
                n1794 = Number To Fractional String(number=w3149) -> (F-format string=w3152:string)  [unwired: 3 in]
                n1795 = String Subset(string=w3152, length (rest)=6 ("length (rest)")) -> (substring=w3150:string)  [unwired: 1 in]
                n1796 = Concatenate Strings("TGT", w3150) -> (w3141:string)
              }
            }
          }
          event "Normal \nRate (ul/hr)  3": Value Change {
            n1797 = event-data() -> ()  [unwired: 1 in, 5 out]
            n1798 = Number To Fractional String(number="Normal \nRate (ul/hr)  3") -> (F-format string=w3169:string)  [unwired: 3 in]
            n1799 = String Subset(string=w3169, length (rest)=6 ("length (rest)")) -> (substring=w3167:string)  [unwired: 1 in]
            n1800 = Concatenate Strings("RAT", w3167, "UH") -> (w3170:string)
            n1801 = call "Write to pump 2.vi"("String to write"=w3170, "VISA resource name"=w3171) -> ()  [unwired: 8 in, 2 out]
          }
          event "Clear Volume": Value Change {
            n1802 = event-data() -> ()  [unwired: 1 in, 5 out]
            n1803 = Divide(x="Normal \nVolume (ul) 3", y=1000.0) -> (x/y=w3189:dbl)
            n1804 = Number To Fractional String(number=w3189) -> (F-format string=w3192:string)  [unwired: 3 in]
            n1805 = String Subset(string=w3192, length (rest)=6 ("length (rest)")) -> (substring=w3190:string)  [unwired: 1 in]
            n1806 = flat-sequence {
              tunnel: [w3199] -> w3187
              tunnel: [w3198] -> w3186
              tunnel: w3176 -> [w3197]
              tunnel: w3175 -> [w3196]
              tunnel: [w3201] -> w3184
              tunnel: [w3200] -> w3185
              tunnel: w3181 -> [w3202]
              tunnel: w3187 -> [w3201]
              tunnel: w3186 -> [w3200]
              tunnel: w3185 -> [w3206]
              tunnel: w3184 -> [w3207]
              tunnel: [w3205] -> _
              tunnel: [w3204] -> _
              tunnel: w3174 -> [w3203]
              frame #0 {
                n1807 = call "Write to pump 2.vi"("String to write"=w3196, "VISA resource name"=w3197) -> ("error out"=w3198:errorcluster, "VISA resource name out"=w3199:refnum<visa-resource-name>)  [unwired: 8 in]
              }
              frame #1 {
                n1808 = Wait (ms)(milliseconds to wait=w3202) -> ()  [unwired: 1 out]
              }
              frame #2 {
                n1809 = call "Write to pump 2.vi"("error in (no error)"=w3206, "String to write"=w3203, "VISA resource name"=w3207) -> ("error out"=w3204:errorcluster, "VISA resource name out"=w3205:refnum<visa-resource-name>)  [unwired: 7 in]
              }
            }
            n1810 = local read "Write Wait"() -> (w3181:i32)
            n1811 = Concatenate Strings("TGT", w3190) -> (w3175:string)
            n1812 = local read "Normal \nRate (ul/hr)  3"() -> (w3177:dbl)
            n1813 = local write "Clear Volume"(FALSE ("Clear Volume")) -> ()
            n1814 = Number To Fractional String(number=w3177) -> (F-format string=w3180:string)  [unwired: 3 in]
            n1815 = String Subset(string=w3180, length (rest)=6 ("length (rest)")) -> (substring=w3178:string)  [unwired: 1 in]
            n1816 = Concatenate Strings("RAT", w3178, "UH" ("string")) -> (w3174:string)
          }
        }
        n1817 = node-c288() -> ()  [unwired: 1 in, 1 out]
      }
      n1818 = node-c288(w3055) -> ()  [unwired: 1 out]
    }
  }
  n1819 = node-c288() -> (w90:T13)  [unwired: 4 in]
  n1820 = timed-loop {
    timing: w90 -> [_]
    timing-out: [_] -> w89
    stop <- w3214 stop-if-true
    n1821 = node-c288() -> ()  [unwired: 1 in, 1 out]
    n1822 = event shown="[1] \"Stop\": Value Change" {
      selector: _ -> [_ _]
      dyn-events: _ -> [_ _]
      timeout: _ -> [_ _]
      tunnel: [_ w3215] -> w3214
      event Timeout {
        n1823 = event-data() -> ()  [unwired: 1 in, 2 out]
      }
      event "Stop": Value Change {
        n1824 = event-data() -> ()  [unwired: 1 in, 4 out]
        n1825 = flat-sequence {
          tunnel: ["Stop"] -> w3215
          frame #0 {
            w3216 = FALSE ("Force Feedback")
            n1826 = local write "Force Feedback 1"(w3216) -> ()
            n1827 = local write "Force Feedback 2"(w3216) -> ()
            n1828 = property on="Cancel dwell" class="Bool (strict)"("Val(Sgnl)"=TRUE ("Value (Signaling)")) -> ()  [unwired: 2 in, 2 out]
          }
          frame #1 {
            w3218 = FALSE
            n1829 = local write "Raster scanning..."(w3218) -> ()
            n1830 = local write "Cancel dwell"(w3218) -> ()
            n1831 = local write "Stage moving"(w3218) -> ()
            n1832 = local write "Saving Move"(w3218) -> ()
          }
        }
      }
    }
    n1833 = node-c288() -> ()  [unwired: 1 in, 1 out]
  }
  n1834 = case shown="True" w80 {
    tunnel: w85 -> [_ w3224]
    tunnel: w84 -> [_ w3223]
    tunnel: w83 -> [_ w3222]
    frame False {
    }
    frame True {
      w3226 = T24 3 items=["no dialog", "OK message", "continue or stop message", "OK message + warnings", "continue/stop + warnings"] ("type of dialog (OK msg:1)")
      w3225 = T24 3 items=["no dialog", "OK message", "continue or stop message", "OK message + warnings", "continue/stop + warnings"] ("type of dialog (OK msg:1)")
      n1835 = call <vilib>:"DAQmx Clear Task.vi"("task in"=w3224, "error in"=w3222) -> ("error out"=w3227:errorcluster)  [unwired: 13 in]
      n1836 = call <vilib>:"DAQmx Clear Task.vi"("task in"=w3223) -> ("error out"=w3228:errorcluster)  [unwired: 14 in]
      n1837 = call <vilib>:"Simple Error Handler.vi"("type of dialog (OK msg:1)"=w3226, "error in (no error)"=w3227) -> ()  [unwired: 3 in, 5 out]
      n1838 = call <vilib>:"Simple Error Handler.vi"("type of dialog (OK msg:1)"=w3225, "error in (no error)"=w3228) -> ()  [unwired: 3 in, 5 out]
    }
  }
  n1839 = case shown="\"Raster scan\"" "?" {
    frame "Force Feedback", Default {
    }
    frame "Raster scan" {
    }
  }
  n1840 = node-c288(w89) -> ()  [unwired: 1 out]
  n1841 = node-c288(w92) -> ()  [unwired: 1 out]
  n1842 = local write "Pause Mouse/Mirror Connection"(FALSE ("Pause Mouse/Mirror Connection")) -> ()
  n1843 = local write "Stop"(FALSE ("Stop all")) -> ()
  "CoordinatesMousePressed" <- T5 {"Horizontal"=0, "Vertical"=0} ("Coords when pressed")
  "Deflection" <- T5 {"Horizontal"=0, "Vertical"=0} ("Coords when pressed")
